vi "LaundryLab.vi"() -> ()   [LabVIEW 2016]
uses:
  Type Definitions/ViperHawk/ViperHawk Status.ctl
  Utility/Custom Pallet Controls/Custom Pallet String.ctl
  Utility/LabVIEW GEA2 Toolkit v1.0.0.0/type defs/Data In.ctl
  Utility/LabVIEW GEA2 Toolkit v1.0.0.0/type defs/Data Out.ctl
  Type Definitions/ViperHawk/ViperHawk Plot File.ctl
  Type Definitions/ViperHawk/ViperHawk Diagnostic Data.ctl
  Utility/Save File/Public/Type Definitions/Save File Software Version.ctl
  Type Definitions/ViperHawk/ViperHawk Summary Stats.ctl
  Utility/Save File/File Setup (Public)/Type Definition/Save File DOE File Path Control.ctl
  Utility/Save File/File Setup (Public)/Type Definition/Save File DOE Data Save Filepaths.ctl
  Type Definitions/ViperHawk/ViperHawk Data.ctl
  Type Definitions/ViperHawk/ViperHawk Search Control.ctl
  C:/Technology Lab/NI-2010/Trunk/Utility/LabVIEW GEA2 Toolkit v1.0.0.0/Appliance.NET/GeaCommunication.dll
  Utility/LabVIEW GEA2 Toolkit v1.0.0.0/Appliance.NET/GeaCommunication.dll
  Utility/GEA2 Commands/HEWH/Type Definitions/GEA2 Commands WaterHeater GEA2 Data.ctl
  Utility/GEA2 Commands/HEWH/Type Definitions/GEA2 Commands Button Status.ctl
  Utility/GEA2 Commands/HEWH/Type Definitions/GEA2 Commands Status Query.ctl
  Utility/GEA2 Commands/HEWH/Type Definitions/GEA2 Commands Service Error Codes.ctl
  Type Definitions/HCC Washer Types.ctl
  Utility/Save File/Public/Type Definitions/Save File Washer.ctl
  Utility/Save File/File Setup (Public)/Type Definition/Save File DISH Dishwasher Details.ctl
  <vilib>/Platform/fileVersionInfo.llb/FileVersionInformation.ctl
  Washer DOE/Type Definitions/DOE Appliance Common.ctl
  Utility/Save File/File Setup (Public)/Type Definition/DPT IMC Data.ctl
  Washer DOE/Type Definitions/DOE Dryer Standard.ctl
  Utility/Save File/Public/Type Definitions/Save File Appliance Display.ctl
  Utility/Save File/Public/Type Definitions/Save File Unit Type.ctl
  Type Definitions/2015 Program/Fault_Buffer_Status.ctl
  Type Definitions/2015 Program/Cycle_Diag_Buffer_Status.ctl
  Utility/LabVIEW GEA2 Toolkit v1.0.0.0/type defs/Source_Destination.ctl
  Utility/LabVIEW GEA2 Toolkit v1.0.0.0/type defs/ERD Write Data In.ctl
  Utility/LabVIEW GEA2 Toolkit v1.0.0.0/type defs/Data Type.ctl
  Utility/LabVIEW GEA2 Toolkit v1.0.0.0/type defs/ERD Read Data In.ctl
  Utility/LabVIEW GEA2 Toolkit v1.0.0.0/type defs/ERD Read Data Out.ctl
  Utility/Save File/Public/Type Definitions/Save File Headers.ctl
  Type Definitions/ViperHawk/ViperHawk Timers.ctl
  Utility/Save File/File Setup (Public)/Type Definition/Save File DOE LabView Program.ctl
  <vilib>/event_ctls.llb/lveventtype.ctl
  Type Definitions/ViperHawk/ViperHawk logData.ctl
  <vilib>/Utility/file.llb/Write Delimited Spreadsheet (string).vi
  Utility/LabVIEW GEA2 Toolkit v1.0.0.0/library/GEA2_Toolkit.lvlib
  user32.dll
  Utility/Save File/Save File.lvlib
  Utility/Save File/File Setup.lvlib
panel:
  out "Network Var Set":u8
  out "Diagnostic Data Output":T1={"Speed (RPM)"=39, "Load Size"=0, "Temperature"=105, "Water Pressure"=4130.0, "Detergent"=11000, "Fabric Softener"=11000, "Tub Direction"="CCW", "Detergent Valve"=FALSE, "Fabric Softener Valve"=FALSE, "Recirculating Pump"=FALSE, "Drain Valve"=FALSE, "Hot Valve"=FALSE, "Cold Valve"=FALSE, "Lid Closed Status"="", "Lid Lock Status"="", "Error Count"=0, "IGBT Temperature (Deg C)"=65, "Motor Speed"=21, "Latched OOB"=0, "Raw OOB"=2525, "Plaster Status"=0, "Inverter Power (W)"=453, "Target Speed(BRPM)"=0, "Latched Agitate Motor Temp (Deg C)"=123, "Current Motor Temp (Deg C)"=123, "Profiler Status"="A899", "Current Inverter Action"="Profiler", "Error Codes"="Door UnlockDoor Open", "Lid Locked"=TRUE, "Lid Closed"=TRUE, "9E Diagnostic Data"={"Total Cycle Time (Min)"=3002, "Total Cycle Count (Current)"=34, "Total Error Count"=21, "Machine Error History"=0, "Washer UI History"=0, "Inverter Error History"=342101761, "Cycle Storage Limit"=1, "Error Storage Limit"=0, "Cycle Pages Supported"=0, "Error Pages Supported"=129, "Inverter Reset Count"=0}, "9F Diagnostic Data"={"Cycle Buffer Index"="", "Page Number"="", "Total Cycle Count"=0, "Delay Start Time"=0, "Stain Selected"="", "Selected Cycle"=0, "eWash"="", "Soil Level"="", "Temperature"="", "Overnight Ready"="", "Spin Setting"="", "Control Lock Status"="", "Stain Remover"="", "Steam Assist"="", "My Cycle"="", "PreWash"="", "Debug Log Enabled"="", "Rinse"="", "Signal Level"="", "PreSoak"=""}}
  out "Diagnostic Data Local":T1={"Speed (RPM)"=0, "Load Size"=0, "Temperature"=0, "Water Pressure"=0.0, "Detergent"=0, "Fabric Softener"=0, "Tub Direction"="", "Detergent Valve"=FALSE, "Fabric Softener Valve"=FALSE, "Recirculating Pump"=FALSE, "Drain Valve"=FALSE, "Hot Valve"=FALSE, "Cold Valve"=FALSE, "Lid Closed Status"="", "Lid Lock Status"="", "Error Count"=0, "IGBT Temperature (Deg C)"=0, "Motor Speed"=0, "Latched OOB"=0, "Raw OOB"=0, "Plaster Status"=0, "Inverter Power (W)"=0, "Target Speed(BRPM)"=0, "Latched Agitate Motor Temp (Deg C)"=0, "Current Motor Temp (Deg C)"=0, "Profiler Status"="", "Current Inverter Action"="", "Error Codes"="", "Lid Locked"=FALSE, "Lid Closed"=FALSE, "9E Diagnostic Data"={"Total Cycle Time (Min)"=3002, "Total Cycle Count (Current)"=34, "Total Error Count"=21, "Machine Error History"=0, "Washer UI History"=0, "Inverter Error History"=342101761, "Cycle Storage Limit"=1, "Error Storage Limit"=0, "Cycle Pages Supported"=0, "Error Pages Supported"=129, "Inverter Reset Count"=0}, "9F Diagnostic Data"={"Cycle Buffer Index"="", "Page Number"="", "Total Cycle Count"=0, "Delay Start Time"=0, "Stain Selected"="", "Selected Cycle"=0, "eWash"="", "Soil Level"="", "Temperature"="", "Overnight Ready"="", "Spin Setting"="", "Control Lock Status"="", "Stain Remover"="", "Steam Assist"="", "My Cycle"="", "PreWash"="", "Debug Log Enabled"="", "Rinse"="", "Signal Level"="", "PreSoak"=""}}
  out "GEA Information Out":T2={"GEA Diagnostic Data - Washer"={"Speed (RPM)"=39, "Load Size"=0, "Temperature"=105, "Water Pressure"=4130.0, "Detergent"=11000, "Fabric Softener"=11000, "Tub Direction"="CCW", "Detergent Valve"=FALSE, "Fabric Softener Valve"=FALSE, "Recirculating Pump"=FALSE, "Drain Valve"=FALSE, "Hot Valve"=FALSE, "Cold Valve"=FALSE, "Lid Closed Status"="", "Lid Lock Status"="", "Error Count"=0, "IGBT Temperature (Deg C)"=65, "Motor Speed"=21, "Latched OOB"=0, "Raw OOB"=2525, "Plaster Status"=0, "Inverter Power (W)"=453, "Target Speed(BRPM)"=0, "Latched Agitate Motor Temp (Deg C)"=123, "Current Motor Temp (Deg C)"=123, "Profiler Status"="A899", "Current Inverter Action"="Profiler", "Error Codes"="Door UnlockDoor Open", "Lid Locked"=TRUE, "Lid Closed"=TRUE, "9E Diagnostic Data"={"Total Cycle Time (Min)"=3002, "Total Cycle Count (Current)"=34, "Total Error Count"=21, "Machine Error History"=0, "Washer UI History"=0, "Inverter Error History"=342101761, "Cycle Storage Limit"=1, "Error Storage Limit"=0, "Cycle Pages Supported"=0, "Error Pages Supported"=129, "Inverter Reset Count"=0}, "9F Diagnostic Data"={"Cycle Buffer Index"="", "Page Number"="", "Total Cycle Count"=0, "Delay Start Time"=0, "Stain Selected"="", "Selected Cycle"=0, "eWash"="", "Soil Level"="", "Temperature"="", "Overnight Ready"="", "Spin Setting"="", "Control Lock Status"="", "Stain Remover"="", "Steam Assist"="", "My Cycle"="", "PreWash"="", "Debug Log Enabled"="", "Rinse"="", "Signal Level"="", "PreSoak"=""}}, "Software Version"={"Critical Major SW Version"="0", "Critical Minor SW Version"="0", "Major SW Version"="41", "Minor SW Version"="1", "Parametric Data Ver. Major"="1", "Parametric Data Ver. Minor"="1", "Diagnostics Data Ver. Major"="", "Diagnostics Data Ver. Minor"="", "Current Personality Setting"=""}, "Debug Search Parameters"={"Pause"=["MchStdby", "MchPz", "MchIdl", "Machine Standby", "Machine Pause", "Machine Idle"], "Run"=["MchRn", "Machine Run", "Resume Process"], "EOC"=["EOC"], "Error Codes"=["Error1", "try", "rty", "inverr"]}, "Message Count"=0, "Number of Messages"=0, "Partial Message String"="", "Full Message to Save"="117 1MnPwrDtaStrd", "Board ID"="", "Board Index"=0, "Source Address"=228, "Destination Address"=35, "Data to send"=[], "ReceivedData"=[1, 0, 21, 0, 0, 0, 0, 9, 221, 65, 0, 1, 197, 1, 168, 153, 9, 0, 0, 123, 123], "Debug/GEA Data"=["11/06/2015", "10:20:16.735", "117 1MnPwrDtaStrd"], "Command"=0, "GEA2 Reference Out"=refnum, "GEA2 Event Registration"=refnum, "Bus Data"="11/06/15 10:20:40.531 RECV 3F E4 60 7B 7B 00 00 09 99 A8 01 C5 01 00 41 DD 09 00 00 00 00 15 00 01\r\n11/06/15 10:20:40.466 RECV 21 E4 41 27 00 00 00 06 00 EA 00 F8 2A F8 2A 01 08 00 00 0B C7 00 22 10 00 00 00 00 69\r\n11/06/15 10:20:39.988 RECV 23 FF A4 16 03 02\r\n11/06/15 10:20:39.537 RECV 3F E4 60 7B 7B 6E 00 09 99 A8 01 B7 01 00 41 64 14 00 00 00 00 69 00 01\r\n11/06/15 10:20:39.472 RECV 21 E4 41 68 00 00 00 06 00 EA 00 F8 2A F8 2A 11 08 00 00 0B C7 00 19 10 00 00 00 00 69\r\n11/06/15 10:20:38.996 RECV 23 FF A4 16 03 02\r\n11/06/15 10:20:38.871 RECV 23 E4 9E 81 00 00 01 01 0F 64 14 00 00 00 00 00 00 00 00 15 00 22 00 BA 0B 00 00\r\n11/06/15 10:20:38.577 RECV 3F E4 60 7B 7B 00 00 09 99 A8 01 96 01 00 41 87 01 00 00 00 00 24 00 00\r\n11/06/15 10:20:38.512 RECV 21 E4 41 35 00 00 00 06 00 EA 00 F8 2A F8 2A 11 08 00 00 0B C7 00 1A 10 00 00 00 00 69\r\n11/06/15 10:20:38.005 RECV 23 FF A4 16 03 02\r\n11/06/15 10:20:37.553 RECV 3F E4 60 7B 7B 6E 00 09 99 A8 01 9E 01 00 41 56 02 00 00 00 00 64 00 00\r\n11/06/15 10:20:37.486 RECV 21 E4 41 64 00 00 00 06 00 EA 00 F8 2A F8 2A 11 08 00 00 0B C7 00 21 10 00 00 00 00 6A\r\n11/06/15 10:20:37.010 RECV 23 FF A4 16 03 02\r\n11/06/15 10:20:36.558 RECV 3F E4 60 7B 7B 00 00 09 99 A8 01 C7 01 00 41 8C 3D 00 00 00 00 35 00 01\r\n11/06/15 10:20:36.493 RECV 21 E4 41 38 00 00 00 06 00 EA 00 F8 2A F8 2A 11 08 00 00 0B C7 00 1F 10 00 00 00 00 6A\r\n11/06/15 10:20:36.312 RECV 23 E4 9E 81 00 00 01 01 0F 64 14 00 00 00 00 00 00 00 00 15 00 22 00 BA 0B 00 00\r\n11/06/15 10:20:36.017 RECV 23 FF A4 16 03 02\r\n11/06/15 10:20:35.567 RECV 3F E4 60 7B 7B 6E 00 09 99 A8 01 6B 01 00 41 5F 08 00 00 00 00 5F 00 01\r\n11/06/15 10:20:35.501 RECV 21 E4 41 63 00 00 00 06 00 EA 00 F8 2A F8 2A 11 08 00 00 0B C7 00 18 10 00 00 00 00 6A\r\n11/06/15 10:20:35.024 RECV 23 FF A4 16 03 02\r\n11/06/15 10:20:34.573 RECV 3F E4 60 7B 7B 00 00 09 99 A8 01 FF 01 00 41 30 05 00 00 00 00 3D 00 00\r\n11/06/15 10:20:34.505 RECV 21 E4 41 52 00 00 00 06 00 EA 00 F8 2A F8 2A 11 08 00 00 0B C7 00 1D 10 00 00 00 00 6A\r\n11/06/15 10:20:34.031 RECV 23 FF A4 16 03 02\r\n11/06/15 10:20:33.877 RECV 23 E4 9E 81 00 00 01 01 0F 64 14 00 00 00 00 00 00 00 00 15 00 22 00 BA 0B 00 00\r\n11/06/15 10:20:33.581 RECV 3F E4 60 7B 7B 6E 00 09 99 A8 01 95 01 00 41 20 09 00 00 00 00 66 00 00\r\n11/06/15 10:20:33.515 RECV 21 E4 41 5F 00 00 00 06 00 EA 00 F8 2A F8 2A 11 08 00 00 0B C7 00 1F 10 00 00 00 00 6A\r\n11/06/15 10:20:33.038 RECV 23 FF A4 16 03 02\r\n11/06/15 10:20:32.585 RECV 3F E4 60 7B 7B 1E 00 09 99 A8 01 13 02 00 40 4C 0E 00 00 00 00 4C 00 01\r\n11/06/15 10:20:32.519 RECV 21 E4 41 5C 00 00 00 06 00 EA 00 F8 2A F8 2A 11 08 00 00 0B C7 00 1D 10 00 00 00 00 6A\r\n11/06/15 10:20:32.045 RECV 23 FF A4 16 03 02\r\n11/06/15 10:20:31.594 RECV 3F E4 60 7B 7B 6E 00 09 99 A8 01 42 01 00 40 A6 01 00 00 00 00 5F 00 01\r\n11/06/15 10:20:31.527 RECV 21 E4 41 54 00 00 00 06 00 EA 00 F8 2A F8 2A 11 08 00 00 0B C7 00 17 10 00 00 00 00 6A\r\n11/06/15 10:20:31.347 RECV 23 E4 9E 81 00 00 01 01 0F 64 14 00 00 00 00 00 00 00 00 15 00 22 00 BA 0B 00 00\r\n11/06/15 10:20:31.052 RECV 23 FF A4 16 03 02\r\n11/06/15 10:20:30.603 RECV 3F E4 60 7B 7B 1E 00 09 99 A8 01 0B 02 00 40 91 0A 00 00 00 00 6A 00 00\r\n11/06/15 10:20:30.534 RECV 21 E4 41 6E 00 00 00 06 00 EA 00 F8 2A F8 2A 11 08 00 00 0B C7 00 1C 10 00 00 00 00 6A\r\n11/06/15 10:20:30.060 RECV 23 FF A4 16 03 02\r\n11/06/15 10:20:29.607 RECV 3F E4 60 7B 7B 6E 00 09 99 A8 01 45 01 00 40 47 21 00 00 00 00 47 00 00\r\n11/06/15 10:20:29.541 RECV 21 E4 41 2C 00 00 00 06 00 EA 00 F8 2A F8 2A 01 08 00 00 0B C7 00 25 10 00 00 00 00 6A\r\n11/06/15 10:20:29.066 RECV 23 FF A4 16 03 02\r\n11/06/15 10:20:28.912 RECV 23 E4 9E 81 00 00 01 01 0F 64 14 00 00 00 00 00 00 00 00 15 00 22 00 BA 0B 00 00\r\n11/06/15 10:20:28.615 RECV 3F E4 60 7B 7B 6E 00 09 99 A8 01 E7 01 00 40 66 1A 00 00 00 00 6B 00 01\r\n11/06/15 10:20:28.549 RECV 21 E4 41 66 00 00 00 06 00 EA 00 F8 2A F8 2A 11 08 00 00 0B C7 00 25 10 00 00 00 00 6A\r\n11/06/15 10:20:28.073 RECV 23 FF A4 16 03 02\r\n11/06/15 10:20:27.619 RECV 3F E4 60 7B 7B 6E 00 09 99 A8 01 99 00 00 40 E4 20 00 00 00 00 15 00 01\r\n11/06/15 10:20:27.555 RECV 21 E4 41 03 00 00 00 06 00 EA 00 F8 2A F8 2A 01 08 00 00 0B C7 00 23 10 00 00 00 00 6A\r\n11/06/15 10:20:27.080 RECV 23 FF A4 16 03 02\r\n11/06/15 10:20:26.628 RECV 3F E4 60 68 68 00 00 09 99 A8 05 66 00 00 40 00 00 00 00 00 00 01 00 02\r\n11/06/15 10:20:26.563 RECV 21 E4 41 04 00 00 00 06 00 EA 00 F8 2A F8 2A 01 08 00 00 0B C7 00 21 10 00 00 00 00 6A\r\n11/06/15 10:20:26.384 RECV 23 E4 9E 81 00 00 01 01 0F 64 14 00 00 00 00 00 00 00 00 15 00 22 00 BA 0B 00 00\r\n11/06/15 10:20:26.086 RECV 23 FF A4 16 03 02\r\n11/06/15 10:20:25.633 RECV 3F E4 60 68 68 00 00 09 99 A8 05 17 00 00 40 0C 00 00 00 00 00 01 00 00\r\n11/06/15 10:20:25.570 RECV 21 E4 41 09 00 00 00 06 00 EA 00 F8 2A F8 2A 01 08 00 00 0B C7 00 23 10 00 00 00 00 6A\r\n11/06/15 10:20:25.093 RECV 23 FF A4 16 03 02\r\n11/06/15 10:20:24.640 RECV 3F E4 60 68 68 00 00 09 99 A8 05 A0 00 00 40 FA 01 00 00 00 00 06 00 00\r\n11/06/15 10:20:24.576 RECV 21 E4 41 0D 00 00 00 06 00 EA 00 F8 2A F8 2A 01 08 00 00 0B C7 00 20 10 00 00 00 00 6A\r\n11/06/15 10:20:24.100 RECV 23 FF A4 16 03 02\r\n11/06/15 10:20:23.947 RECV 23 E4 9E 81 00 00 01 01 0F 64 14 00 00 00 00 00 00 00 00 15 00 22 00 BA 0B 00 00\r\n11/06/15 10:20:23.651 RECV 3F E4 60 68 68 6E 00 09 99 A8 01 FF 01 00 40 8C 08 00 00 00 00 6E 00 00\r\n11/06/15 10:20:23.583 RECV 21 E4 41 6D 00 00 00 06 00 EA 00 F8 2A F8 2A 11 08 00 00 0B C7 00 1E 10 00 00 00 00 6A\r\n11/06/15 10:20:23.110 RECV 23 FF A4 16 03 02\r\n11/06/15 10:20:22.656 RECV 3F E4 60 68 68 6E 00 09 99 A8 01 C2 01 00 40 74 0B 00 00 00 00 23 00 01\r\n11/06/15 10:20:22.590 RECV 21 E4 41 51 00 00 00 06 00 EA 00 F8 2A F8 2A 11 08 00 00 0B C7 00 1B 10 00 00 00 00 6A\r\n11/06/15 10:20:22.115 RECV 23 FF A4 16 03 02\r\n11/06/15 10:20:21.662 RECV 3F E4 60 68 68 6E 00 09 99 A8 01 8D 01 00 40 F5 0D 00 00 00 00 5C 00 01\r\n11/06/15 10:20:21.596 RECV 21 E4 41 5E 00 00 00 06 00 EA 00 F8 2A F8 2A 11 08 00 00 0B C7 00 13 10 00 00 00 00 6A\r\n11/06/15 10:20:21.419 RECV 23 E4 9E 81 00 00 01 01 0F 64 14 00 00 00 00 00 00 00 00 15 00 22 00 BA 0B 00 00\r\n11/06/15 10:20:21.122 RECV 23 FF A4 16 03 02\r\n11/06/15 10:20:20.671 RECV 3F E4 60 68 68 6E 00 09 99 A8 01 F7 01 00 40 EA 0C 00 00 00 00 67 00 00\r\n11/06/15 10:20:20.605 RECV 21 E4 41 6E 00 00 00 06 00 EA 00 F8 2A F8 2A 11 08 00 00 0B C7 00 18 10 00 00 00 00 6A\r\n11/06/15 10:20:20.128 RECV 23 FF A4 16 03 02\r\n11/06/15 10:20:19.678 RECV 3F E4 60 68 68 6E 00 09 99 A8 01 54 01 00 40 96 12 00 00 00 00 35 00 00\r\n11/06/15 10:20:19.611 RECV 21 E4 41 25 00 00 00 06 00 EA 00 F8 2A F8 2A 01 08 00 00 0B C7 00 1B 10 00 00 00 00 6A\r\n11/06/15 10:20:19.135 RECV 23 FF A4 16 03 02\r\n11/06/15 10:20:19.006 RECV 23 E4 9E 81 00 00 01 01 0F 64 14 00 00 00 00 00 00 00 00 15 00 22 00 BA 0B 00 00\r\n11/06/15 10:20:18.699 RECV 3F E4 60 68 68 6E 00 09 99 A8 01 4E 01 00 40 05 05 00 00 00 00 67 00 01\r\n11/06/15 10:20:18.616 RECV 21 E4 41 67 00 00 00 06 00 EA 00 F8 2A F8 2A 11 08 00 00 0B C7 00 1C 10 00 00 00 00 6A\r\n11/06/15 10:20:18.146 RECV 23 FF A4 16 03 02\r\n11/06/15 10:20:17.717 RECV 3F E4 60 68 68 00 00 09 99 A8 01 5D 01 00 40 30 05 00 00 00 00 25 00 00\r\n11/06/15 10:20:17.616 RECV 21 E4 41 34 00 00 00 06 00 EA 00 F8 2A F8 2A 11 08 00 00 0B C7 00 1D 10 00 00 00 00 6A\r\n11/06/15 10:20:17.148 RECV 23 FF A4 16 03 02\r\n11/06/15 10:20:16.729 RECV 23 FF 74 0A 64 72 74 53 61 74 44 72 77 50 6E 4D 31 20 37 31 31\r\n11/06/15 10:20:16.700 RECV 3F E4 60 68 68 6E 00 09 99 A8 01 90 01 00 40 55 12 00 00 00 00 65 00 00\r\n11/06/15 10:20:16.629 RECV 21 E4 41 64 00 00 00 06 00 EA 00 F8 2A F8 2A 11 08 00 00 0B C7 00 17 10 00 00 00 00 6A\r\n11/06/15 10:20:16.450 RECV 23 E4 9E 81 00 00 01 01 0F 64 14 00 00 00 00 00 00 00 00 15 00 22 00 BA 0B 00 00\r\n11/06/15 10:20:16.155 RECV 23 FF A4 16 03 02\r\n11/06/15 10:20:15.738 RECV 3F E4 60 68 68 00 00 09 99 A8 01 D5 01 00 40 7E 32 00 00 00 00 36 00 01\r\n11/06/15 10:20:15.672 RECV 21 E4 41 39 00 00 00 06 00 EA 00 F8 2A F8 2A 11 08 00 00 0B C7 00 1B 10 00 00 00 00 6A\r\n11/06/15 10:20:15.163 RECV 23 FF A4 16 03 02\r\n11/06/15 10:20:14.738 RECV 3F E4 60 68 68 6E 00 09 99 A8 01 45 01 00 40 28 0A 00 00 00 00 68 00 01\r\n11/06/15 10:20:14.644 RECV 21 E4 41 63 00 00 00 06 00 EA 00 F8 2A F8 2A 11 08 00 00 0B C7 00 18 10 00 00 00 00 6A\r\n11/06/15 10:20:14.170 RECV 23 FF A4 16 03 02\r\n11/06/15 10:20:14.013 RECV 23 E4 9E 81 00 00 01 01 0F 64 14 00 00 00 00 00 00 00 00 15 00 22 00 BA 0B 00 00\r\n11/06/15 10:20:13.717 RECV 3F E4 60 68 68 1E 00 09 99 A8 01 7D 01 00 40 57 17 00 00 00 00 3D 00 00\r\n11/06/15 10:20:13.651 RECV 21 E4 41 51 00 00 00 06 00 EA 00 F8 2A F8 2A 11 08 00 00 0B C7 00 16 10 00 00 00 00 6A\r\n11/06/15 10:20:13.176 RECV 23 FF A4 16 03 02\r\n11/06/15 10:20:12.753 RECV 3F E4 60 68 68 6E 00 09 99 A8 01 3F 01 00 40 EC 09 00 00 00 00 58 00 00\r\n11/06/15 10:20:12.658 RECV 21 E4 41 54 00 00 00 06 00 EA 00 F8 2A F8 2A 11 08 00 00 0B C7 00 17 10 00 00 00 00 6A\r\n11/06/15 10:20:12.184 RECV 23 FF A4 16 03 02\r\n11/06/15 10:20:11.733 RECV 3F E4 60 68 68 1E 00 09 99 A8 01 9E 01 00 40 B6 00 00 00 00 00 59 00 01\r\n11/06/15 10:20:11.667 RECV 21 E4 41 64 00 00 00 06 00 EA 00 F8 2A F8 2A 11 08 00 00 0B C7 00 19 10 00 00 00 00 6A\r\n11/06/15 10:20:11.488 RECV 23 E4 9E 81 00 00 01 01 0F 64 14 00 00 00 00 00 00 00 00 15 00 22 00 BA 0B 00 00\r\n11/06/15 10:20:11.191 RECV 23 FF A4 16 03 02\r\n11/06/15 10:20:10.759 RECV 3F E4 60 68 68 6E 00 09 99 A8 01 0C 01 00 40 45 01 00 00 00 00 57 00 01\r\n11/06/15 10:20:10.673 RECV 21 E4 41 50 00 00 00 06 00 EA 00 F8 2A F8 2A 11 08 00 00 0B C7 00 1C 10 00 00 00 00 6A\r\n11/06/15 10:20:10.198 RECV 23 FF A4 16 03 02\r\n11/06/15 10:20:09.749 RECV 3F E4 60 68 68 1E 00 09 99 A8 01 D1 01 00 40 96 0A 00 00 00 00 6D 00 00\r\n11/06/15 10:20:09.681 RECV 21 E4 41 6F 00 00 00 06 00 EA 00 F8 2A F8 2A 11 08 00 00 0B C7 00 24 10 00 00 00 00 6A\r\n11/06/15 10:20:09.205 RECV 23 FF A4 16 03 02\r\n11/06/15 10:20:09.110 RECV 23 E4 9E 81 00 00 01 01 0F 64 14 00 00 00 00 00 00 00 00 15 00 22 00 BA 0B 00 00\r\n11/06/15 10:20:08.813 RECV 3F E4 60 68 68 6E 00 09 99 A8 01 18 01 00 40 64 04 00 00 00 00 4F 00 00\r\n11/06/15 10:20:08.749 RECV 21 E4 41 43 00 00 00 06 00 EA 00 F8 2A F8 2A 11 08 00 00 0B C7 00 1F 10 00 00 00 00 6A\r\n11/06/15 10:20:08.212 RECV 23 FF A4 16 03 02\r\n11/06/15 10:20:07.760 RECV 3F E4 60 68 68 6E 00 09 99 A8 01 C1 01 00 40 51 05 00 00 00 00 6C 00 01\r\n11/06/15 10:20:07.693 RECV 21 E4 41 6C 00 00 00 06 00 EA 00 F8 2A F8 2A 11 08 00 00 0B C7 00 19 10 00 00 00 00 6A\r\n11/06/15 10:20:07.218 RECV 23 FF A4 16 03 02\r\n11/06/15 10:20:06.764 RECV 3F E4 60 68 68 6E 00 09 99 A8 01 08 01 00 40 26 34 00 00 00 00 38 00 01\r\n11/06/15 10:20:06.698 RECV 21 E4 41 19 00 00 00 06 00 EA 00 F8 2A F8 2A 01 08 00 00 0B C7 00 15 10 00 00 00 00 6A\r\n11/06/15 10:20:06.522 RECV 23 E4 9E 81 00 00 01 01 0F 64 14 00 00 00 00 00 00 00 00 15 00 22 00 BA 0B 00 00\r\n11/06/15 10:20:06.226 RECV 23 FF A4 16 03 02\r\n11/06/15 10:20:05.775 RECV 3F E4 60 68 68 6E 00 09 99 A8 01 C9 01 00 40 4A 09 00 00 00 00 6A 00 00\r\n11/06/15 10:20:05.709 RECV 21 E4 41 6B 00 00 00 06 00 EA 00 F8 2A F8 2A 11 08 00 00 0B C7 00 17 10 00 00 00 00 6A\r\n11/06/15 10:20:05.232 RECV 23 FF A4 16 03 02\r\n11/06/15 10:20:04.714 RECV 21 E4 41 1A 00 00 00 06 00 EA 00 F8 2A F8 2A 01 08 00 00 0B C7 00 1B 10 00 00 00 00 6A\r\n11/06/15 10:20:04.239 RECV 23 FF A4 16 03 02\r\n11/06/15 10:20:04.082 RECV 23 E4 9E 81 00 00 01 01 0F 64 14 00 00 00 00 00 00 00 00 15 00 22 00 BA 0B 00 00\r\n11/06/15 10:20:03.787 RECV 3F E4 60 68 68 6E 00 09 99 A8 01 B2 01 00 40 2C 09 00 00 00 00 6B 00 01\r\n11/06/15 10:20:03.723 RECV 21 E4 41 6D 00 00 00 06 00 EA 00 F8 2A F8 2A 11 08 00 00 0B C7 00 1C 10 00 00 00 00 6A\r\n11/06/15 10:20:03.246 RECV 23 FF A4 16 03 02\r\n11/06/15 10:20:02.794 RECV 3F E4 60 68 68 6E 00 09 99 A8 01 0F 01 00 40 16 01 00 00 00 00 0C 00 01\r\n11/06/15 10:20:02.728 RECV 21 E4 41 25 00 00 00 06 00 EA 00 F8 2A F8 2A 01 08 00 00 0B C7 00 1E 10 00 00 00 00 6A\r\n11/06/15 10:20:02.253 RECV 23 FF A4 16 03 02\r\n11/06/15 10:20:01.817 RECV 3F E4 60 68 68 6E 00 09 99 A8 01 D5 01 00 40 F1 07 00 00 00 00 67 00 00\r\n11/06/15 10:20:01.736 RECV 21 E4 41 69 00 00 00 06 00 EA 00 F8 2A F8 2A 11 08 00 00 0B C7 00 1F 10 00 00 00 00 6A\r\n11/06/15 10:20:01.557 RECV 23 E4 9E 81 00 00 01 01 0F 64 14 00 00 00 00 00 00 00 00 15 00 22 00 BA 0B 00 00\r\n11/06/15 10:20:01.261 RECV 23 FF A4 16 03 02\r\n11/06/15 10:20:00.817 RECV 3F E4 60 68 68 00 00 09 99 A8 01 80 01 00 40 59 08 00 00 00 00 16 00 01\r\n11/06/15 10:20:00.741 RECV 21 E4 41 29 00 00 00 06 00 EA 00 F8 2A F8 2A 01 08 00 00 0B C7 00 1F 10 00 00 00 00 6A\r\n11/06/15 10:20:00.267 RECV 23 FF A4 16 03 02\r\n11/06/15 10:19:59.748 RECV 21 E4 41 63 00 00 00 06 00 EA 00 F8 2A F8 2A 11 08 00 00 0B C7 00 19 10 00 00 00 00 6A\r\n11/06/15 10:19:59.275 RECV 23 FF A4 16 03 02\r\n11/06/15 10:19:59.116 RECV 23 E4 9E 81 00 00 01 01 0F 64 14 00 00 00 00 00 00 00 00 15 00 22 00 BA 0B 00 00\r\n11/06/15 10:19:58.821 RECV 3F E4 60 68 68 00 00 09 99 A8 01 5F 01 00 40 AB 06 00 00 00 00 20 00 00\r\n11/06/15 10:19:58.756 RECV 21 E4 41 2E 00 00 00 06 00 EA 00 F8 2A F8 2A 01 08 00 00 0B C7 00 1C 10 00 00 00 00 6A\r\n11/06/15 10:19:58.279 RECV 23 FF A4 16 03 02\r\n11/06/15 10:19:57.869 RECV 3F E4 60 68 68 6E 00 09 99 A8 01 A8 01 00 40 5A 04 00 00 00 00 6F 00 00\r\n11/06/15 10:19:57.763 RECV 21 E4 41 69 00 00 00 06 00 EA 00 F8 2A F8 2A 11 08 00 00 0B C7 00 1C 10 00 00 00 00 6A\r\n11/06/15 10:19:57.288 RECV 23 FF A4 16 03 02\r\n11/06/15 10:19:56.853 RECV 3F E4 60 68 68 00 00 09 99 A8 01 AC 01 00 40 00 08 00 00 00 00 20 00 01\r\n11/06/15 10:19:56.771 RECV 21 E4 41 39 00 00 00 06 00 EA 00 F8 2A F8 2A 11 08 00 00 0B C7 00 1C 10 00 00 00 00 6A\r\n11/06/15 10:19:56.591 RECV 23 E4 9E 81 00 00 01 01 0F 64 14 00 00 00 00 00 00 00 00 15 00 22 00 BA 0B 00 00\r\n11/06/15 10:19:56.294 RECV 23 FF A4 16 03 02\r\n11/06/15 10:19:55.840 RECV 3F E4 60 68 68 6E 00 09 99 A8 01 8D 01 00 40 17 13 00 00 00 00 6A 00 01\r\n11/06/15 10:19:55.773 RECV 21 E4 41 67 00 00 00 06 00 EA 00 F8 2A F8 2A 11 08 00 00 0B C7 00 1C 10 00 00 00 00 6A\r\n11/06/15 10:19:55.298 RECV 23 FF A4 16 03 02\r\n11/06/15 10:19:54.865 RECV 3F E4 60 68 68 00 00 09 99 A8 01 B0 01 00 3F DE 17 00 00 00 00 36 00 00\r\n11/06/15 10:19:54.783 RECV 21 E4 41 48 00 00 00 06 00 EA 00 F8 2A F8 2A 11 08 00 00 0B C7 00 20 10 00 00 00 00 6A\r\n11/06/15 10:19:54.308 RECV 23 FF A4 16 03 02\r\n11/06/15 10:19:54.153 RECV 23 E4 9E 81 00 00 01 01 0F 64 14 00 00 00 00 00 00 00 00 15 00 22 00 BA 0B 00 00\r\n11/06/15 10:19:53.856 RECV 3F E4 60 68 68 6E 00 09 99 A8 01 83 01 00 3F CD 06 00 00 00 00 5F 00 00\r\n11/06/15 10:19:53.790 RECV 21 E4 41 5D 00 00 00 06 00 EA 00 F8 2A F8 2A 11 08 00 00 0B C7 00 1C 10 00 00 00 00 6A\r\n11/06/15 10:19:53.316 RECV 23 FF A4 16 03 02\r\n11/06/15 10:19:52.865 RECV 3F E4 60 68 68 1E 00 09 99 A8 01 DA 01 00 3F EB 22 00 00 00 00 40 00 01\r\n11/06/15 10:19:52.798 RECV 21 E4 41 5E 00 00 00 06 00 EA 00 F8 2A F8 2A 11 08 00 00 0B C7 00 1E 10 00 00 00 00 6A\r\n11/06/15 10:19:52.322 RECV 23 FF A4 16 03 02\r\n11/06/15 10:19:51.871 RECV 3F E4 60 68 68 6E 00 09 99 A8 01 48 01 00 3F EF 00 00 00 00 00 57 00 01\r\n11/06/15 10:19:51.807 RECV 21 E4 41 53 00 00 00 06 00 EA 00 F8 2A F8 2A 11 08 00 00 0B C7 00 20 10 00 00 00 00 6A\r\n11/06/15 10:19:51.626 RECV 23 E4 9E 81 00 00 01 01 0F 64 14 00 00 00 00 00 00 00 00 15 00 22 00 BA 0B 00 00\r\n11/06/15 10:19:51.329 RECV 23 FF A4 16 03 02\r\n11/06/15 10:19:50.878 RECV 3F E4 60 68 68 1E 00 09 99 A8 01 D7 01 00 3F 97 06 00 00 00 00 66 00 00\r\n11/06/15 10:19:50.811 RECV 21 E4 41 69 00 00 00 06 00 EA 00 F8 2A F8 2A 11 08 00 00 0B C7 00 1E 10 00 00 00 00 6A\r\n11/06/15 10:19:50.337 RECV 23 FF A4 16 03 02\r\n11/06/15 10:19:49.884 RECV 3F E4 60 68 68 6E 00 09 99 A8 01 3D 01 00 3F 5C 17 00 00 00 00 4D 00 00\r\n11/06/15 10:19:49.819 RECV 21 E4 41 45 00 00 00 06 00 EA 00 F8 2A F8 2A 11 08 00 00 0B C7 00 1B 10 00 00 00 00 6A\r\n11/06/15 10:19:49.343 RECV 23 FF A4 16 03 02\r\n11/06/15 10:19:49.191 RECV 23 E4 9E 81 00 00 01 01 0F 64 14 00 00 00 00 00 00 00 00 15 00 22 00 BA 0B 00 00\r\n11/06/15 10:19:48.893 RECV 3F E4 60 68 68 6E 00 09 99 A8 01 CA 01 00 3F EB 03 00 00 00 00 6C 00 01\r\n11/06/15 10:19:48.826 RECV 21 E4 41 70 00 00 00 06 00 EA 00 F8 2A F8 2A 11 08 00 00 0B C7 00 1C 10 00 00 00 00 6A\r\n11/06/15 10:19:48.350 RECV 23 FF A4 16 03 02\r\n11/06/15 10:19:47.898 RECV 3F E4 60 68 68 6E 00 09 99 A8 01 14 01 00 3F 88 08 00 00 00 00 47 00 01\r\n11/06/15 10:19:47.833 RECV 21 E4 41 24 00 00 00 06 00 EA 00 F8 2A F8 2A 01 08 00 00 0B C7 00 1C 10 00 00 00 00 6A\r\n11/06/15 10:19:47.357 RECV 23 FF A4 16 03 02\r\n11/06/15 10:19:46.906 RECV 3F E4 60 68 68 6E 00 09 99 A8 01 E3 01 00 3F 78 13 00 00 00 00 6B 00 00\r\n11/06/15 10:19:46.838 RECV 21 E4 41 6D 00 00 00 06 00 EA 00 F8 2A F8 2A 11 08 00 00 0B C7 00 1B 10 00 00 00 00 6A\r\n11/06/15 10:19:46.659 RECV 23 E4 9E 81 00 00 01 01 0F 64 14 00 00 00 00 00 00 00 00 15 00 22 00 BA 0B 00 00\r\n11/06/15 10:19:46.363 RECV 23 FF A4 16 03 02\r\n11/06/15 10:19:45.910 RECV 3F E4 60 68 68 6E 00 09 99 A8 01 2F 01 00 3F D7 1C 00 00 00 00 36 00 00\r\n11/06/15 10:19:45.845 RECV 21 E4 41 1A 00 00 00 06 00 EA 00 F8 2A F8 2A 01 08 00 00 0B C7 00 14 10 00 00 00 00 6A\r\n11/06/15 10:19:45.370 RECV 23 FF A4 16 03 02\r\n11/06/15 10:19:44.919 RECV 3F E4 60 68 68 6E 00 09 99 A8 01 1A 02 00 3F 1D 29 00 00 00 00 4E 00 01\r\n11/06/15 10:19:44.852 RECV 21 E4 41 63 00 00 00 06 00 EA 00 F8 2A F8 2A 11 08 00 00 0B C7 00 16 10 00 00 00 00 6A\r\n11/06/15 10:19:44.377 RECV 23 FF A4 16 03 02\r\n11/06/15 10:19:44.221 RECV 23 E4 9E 81 00 00 01 01 0F 64 14 00 00 00 00 00 00 00 00 15 00 22 00 BA 0B 00 00\r\n11/06/15 10:19:43.925 RECV 3F E4 60 68 68 6E 00 09 99 A8 01 1C 01 00 3F 7A 0C 00 00 00 00 0A 00 01\r\n11/06/15 10:19:43.859 RECV 21 E4 41 22 00 00 00 06 00 EA 00 F8 2A F8 2A 01 08 00 00 0B C7 00 18 10 00 00 00 00 6A\r\n11/06/15 10:19:43.384 RECV 23 FF A4 16 03 02\r\n11/06/15 10:19:42.950 RECV 3F E4 60 68 68 6E 00 09 99 A8 01 F3 01 00 3F B0 0F 00 00 00 00 69 00 00\r\n11/06/15 10:19:42.867 RECV 21 E4 41 6C 00 00 00 06 00 EA 00 F8 2A F8 2A 11 08 00 00 0B C7 00 1C 10 00 00 00 00 6A\r\n11/06/15 10:19:42.391 RECV 23 FF A4 16 03 02\r\n11/06/15 10:19:41.939 RECV 3F E4 60 68 68 6E 00 09 99 A8 01 60 01 00 3F 28 00 00 00 00 00 11 00 00\r\n11/06/15 10:19:41.875 RECV 21 E4 41 21 00 00 00 06 00 EA 00 F8 2A F8 2A 01 08 00 00 0B C7 00 1C 10 00 00 00 00 6A\r\n11/06/15 10:19:41.694 RECV 23 E4 9E 81 00 00 01 01 0F 64 14 00 00 00 00 00 00 00 00 15 00 22 00 BA 0B 00 00\r\n11/06/15 10:19:41.398 RECV 23 FF A4 16 03 02\r\n11/06/15 10:19:40.974 RECV 3F E4 60 68 68 6E 00 09 99 A8 01 BD 01 00 3F 5F 02 00 00 00 00 5E 00 01\r\n11/06/15 10:19:40.880 RECV 21 E4 41 6B 00 00 00 06 00 EA 00 F8 2A F8 2A 11 08 00 00 0B C7 00 1C 10 00 00 00 00 6A\r\n11/06/15 10:19:40.406 RECV 23 FF A4 16 03 02\r\n11/06/15 10:19:39.952 RECV 3F E4 60 68 68 00 00 09 99 A8 01 54 01 00 3F 70 07 00 00 00 00 14 00 00\r\n11/06/15 10:19:39.885 RECV 21 E4 41 30 00 00 00 06 00 EA 00 F8 2A F8 2A 01 08 00 00 0B C7 00 1C 10 00 00 00 00 6A\r\n11/06/15 10:19:39.413 RECV 23 FF A4 16 03 02\r\n11/06/15 10:19:39.255 RECV 23 E4 9E 81 00 00 01 01 0F 64 14 00 00 00 00 00 00 00 00 15 00 22 00 BA 0B 00 00\r\n11/06/15 10:19:38.959 RECV 3F E4 60 68 68 6E 00 09 99 A8 01 CE 01 00 3F B4 15 00 00 00 00 66 00 00\r\n11/06/15 10:19:38.893 RECV 21 E4 41 6B 00 00 00 06 00 EA 00 F8 2A F8 2A 11 08 00 00 0B C7 00 11 10 00 00 00 00 6A\r\n11/06/15 10:19:38.419 RECV 23 FF A4 16 03 02\r\n11/06/15 10:19:37.969 RECV 3F E4 60 68 68 00 00 09 99 A8 01 9F 01 00 3F E2 07 00 00 00 00 20 00 01\r\n11/06/15 10:19:37.901 RECV 21 E4 41 2C 00 00 00 06 00 EA 00 F8 2A F8 2A 01 08 00 00 0B C7 00 1A 10 00 00 00 00 6A\r\n11/06/15 10:19:37.425 RECV 23 FF A4 16 03 02\r\n11/06/15 10:19:37.003 RECV 3F E4 60 68 68 6E 00 09 99 A8 01 90 01 00 3F C3 11 00 00 00 00 5F 00 01\r\n11/06/15 10:19:36.910 RECV 21 E4 41 64 00 00 00 06 00 EA 00 F8 2A F8 2A 11 08 00 00 0B C7 00 26 10 00 00 00 00 6A\r\n11/06/15 10:19:36.741 RECV 23 E4 9E 81 00 00 01 01 0F 64 14 00 00 00 00 00 00 00 00 15 00 22 00 BA 0B 00 00\r\n11/06/15 10:19:36.433 RECV 23 FF A4 16 03 02\r\n11/06/15 10:19:35.981 RECV 3F E4 60 68 68 00 00 09 99 A8 01 B1 01 00 3F 08 14 00 00 00 00 2D 00 00\r\n11/06/15 10:19:35.914 RECV 21 E4 41 42 00 00 00 06 00 EA 00 F8 2A F8 2A 11 08 00 00 0B C7 00 23 10 00 00 00 00 6A\r\n11/06/15 10:19:35.440 RECV 23 FF A4 16 03 02\r\n11/06/15 10:19:34.989 RECV 3F E4 60 68 68 6E 00 09 99 A8 01 8A 01 00 3F 7C 05 00 00 00 00 67 00 00\r\n11/06/15 10:19:34.923 RECV 21 E4 41 64 00 00 00 06 00 EA 00 F8 2A F8 2A 11 08 00 00 0B C7 00 1E 10 00 00 00 00 6A\r\n11/06/15 10:19:34.446 RECV 23 FF A4 16 03 02\r\n11/06/15 10:19:34.286 RECV 23 E4 9E 81 00 00 01 01 0F 64 14 00 00 00 00 00 00 00 00 15 00 22 00 BA 0B 00 00\r\n11/06/15 10:19:33.992 RECV 3F E4 60 68 68 00 00 09 99 A8 01 A1 01 00 3F 7B 01 00 00 00 00 21 00 01\r\n11/06/15 10:19:33.928 RECV 21 E4 41 3E 00 00 00 06 00 EA 00 F8 2A F8 2A 11 08 00 00 0B C7 00 23 10 00 00 00 00 6A\r\n11/06/15 10:19:33.452 RECV 23 FF A4 16 03 02\r\n11/06/15 10:19:32.998 RECV 3F E4 60 68 68 6E 00 09 99 A8 01 4F 01 00 3F AC 08 00 00 00 00 62 00 01\r\n11/06/15 10:19:32.934 RECV 21 E4 41 60 00 00 00 06 00 EA 00 F8 2A F8 2A 11 08 00 00 0B C7 00 22 10 00 00 00 00 6A\r\n11/06/15 10:19:32.461 RECV 23 FF A4 16 03 02\r\n11/06/15 10:19:32.009 RECV 3F E4 60 68 68 1E 00 09 99 A8 01 BE 01 00 3F 02 1B 00 00 00 00 4E 00 00\r\n11/06/15 10:19:31.942 RECV 21 E4 41 60 00 00 00 06 00 EA 00 F8 2A F8 2A 11 08 00 00 0B C7 00 26 10 00 00 00 00 6A\r\n11/06/15 10:19:31.764 RECV 23 E4 9E 81 00 00 01 01 0F 64 14 00 00 00 00 00 00 00 00 15 00 22 00 BA 0B 00 00\r\n11/06/15 10:19:31.467 RECV 23 FF A4 16 03 02\r\n11/06/15 10:19:31.015 RECV 3F E4 60 68 68 6E 00 09 99 A8 01 45 01 00 3F 43 09 00 00 00 00 50 00 00\r\n11/06/15 10:19:30.949 RECV 21 E4 41 50 00 00 00 06 00 EA 00 F8 2A F8 2A 11 08 00 00 0B C7 00 20 10 00 00 00 00 6A\r\n11/06/15 10:19:30.475 RECV 23 FF A4 16 03 02\r\n11/06/15 10:19:30.026 RECV 3F E4 60 68 68 1E 00 09 99 A8 01 E3 01 00 3F FF 00 00 00 00 00 5B 00 01\r\n11/06/15 10:19:29.956 RECV 21 E4 41 69 00 00 00 06 00 EA 00 F8 2A F8 2A 11 08 00 00 0B C7 00 1C 10 00 00 00 00 6A\r\n11/06/15 10:19:29.481 RECV 23 FF A4 16 03 02\r\n11/06/15 10:19:29.327 RECV 23 E4 9E 81 00 00 01 01 0F 64 14 00 00 00 00 00 00 00 00 15 00 22 00 BA 0B 00 00\r\n11/06/15 10:19:29.030 RECV 3F E4 60 68 68 6E 00 09 99 A8 01 8F 01 00 3F 52 0E 00 00 00 00 4E 00 01\r\n11/06/15 10:19:28.966 RECV 21 E4 41 41 00 00 00 06 00 EA 00 F8 2A F8 2A 11 08 00 00 0B C7 00 1B 10 00 00 00 00 6A\r\n11/06/15 10:19:28.489 RECV 23 FF A4 16 03 02\r\n11/06/15 10:19:28.038 RECV 3F E4 60 68 68 6E 00 09 99 A8 01 07 02 00 3E 10 15 00 00 00 00 66 00 00\r\n11/06/15 10:19:27.973 RECV 21 E4 41 67 00 00 00 06 00 EA 00 F8 2A F8 2A 11 08 00 00 0B C7 00 1A 10 00 00 00 00 6A\r\n11/06/15 10:19:27.494 RECV 23 FF A4 16 03 02\r\n11/06/15 10:19:27.042 RECV 3F E4 60 68 68 6E 00 09 99 A8 01 CD 01 00 3E F4 25 00 00 00 00 1A 00 00\r\n11/06/15 10:19:26.977 RECV 21 E4 41 43 00 00 00 06 00 EA 00 F8 2A F8 2A 11 08 00 00 0B C7 00 20 10 00 00 00 00 6A\r\n11/06/15 10:19:26.798 RECV 23 E4 9E 81 00 00 01 01 0F 64 14 00 00 00 00 00 00 00 00 15 00 22 00 BA 0B 00 00\r\n11/06/15 10:19:26.502 RECV 23 FF A4 16 03 02\r\n11/06/15 10:19:26.049 RECV 3F E4 60 68 68 6E 00 09 99 A8 01 DE 01 00 3E FE 04 00 00 00 00 65 00 01\r\n11/06/15 10:19:25.983 RECV 21 E4 41 62 00 00 00 06 00 EA 00 F8 2A F8 2A 11 08 00 00 0B C7 00 10 10 00 00 00 00 6B\r\n11/06/15 10:19:25.508 RECV 23 FF A4 16 03 02\r\n11/06/15 10:19:25.058 RECV 3F E4 60 68 68 6E 00 09 99 A8 01 57 02 00 3E E4 0C 00 00 00 00 6E 00 00\r\n11/06/15 10:19:24.991 RECV 21 E4 41 71 00 00 00 06 00 EA 00 F8 2A F8 2A 11 08 00 00 0B C7 00 19 10 00 00 00 00 6B\r\n11/06/15 10:19:24.516 RECV 23 FF A4 16 03 02\r\n11/06/15 10:19:24.356 RECV 23 E4 9E 81 00 00 01 01 0F 64 14 00 00 00 00 00 00 00 00 15 00 22 00 BA 0B 00 00\r\n11/06/15 10:19:24.061 RECV 3F E4 60 68 68 6E 00 09 99 A8 01 AE 01 00 3E 65 10 00 00 00 00 40 00 00\r\n11/06/15 10:19:23.995 RECV 21 E4 41 33 00 00 00 06 00 EA 00 F8 2A F8 2A 11 08 00 00 0B C7 00 1B 10 00 00 00 00 6A\r\n11/06/15 10:19:23.522 RECV 23 FF A4 16 03 02\r\n11/06/15 10:19:23.072 RECV 3F E4 60 68 68 6E 00 09 99 A8 01 9F 01 00 3E D7 0F 00 00 00 00 6C 00 01\r\n11/06/15 10:19:23.004 RECV 21 E4 41 6A 00 00 00 06 00 EA 00 F8 2A F8 2A 11 08 00 00 0B C7 00 19 10 00 00 00 00 6A\r\n11/06/15 10:19:22.529 RECV 23 FF A4 16 03 02\r\n11/06/15 10:19:22.077 RECV 3F E4 60 68 68 00 00 09 99 A8 01 75 01 00 3E F5 06 00 00 00 00 25 00 00\r\n11/06/15 10:19:22.011 RECV 21 E4 41 2E 00 00 00 06 00 EA 00 F8 2A F8 2A 01 08 00 00 0B C7 00 1D 10 00 00 00 00 68\r\n11/06/15 10:19:21.834 RECV 23 E4 9E 81 00 00 01 01 0F 64 14 00 00 00 00 00 00 00 00 15 00 22 00 BA 0B 00 00\r\n11/06/15 10:19:21.538 RECV 23 FF A4 16 03 02\r\n11/06/15 10:19:21.228 RECV 3F E4 60 68 68 6E 00 09 99 A8 01 81 01 00 3E 4A 05 00 00 00 00 69 00 00\r\n11/06/15 10:19:21.021 RECV 21 E4 41 64 00 00 00 06 00 EA 00 F8 2A F8 2A 11 08 00 00 1B C7 00 18 10 00 00 00 00 68\r\n11/06/15 10:19:20.544 RECV 23 FF A4 16 03 02\r\n11/06/15 10:19:20.090 RECV 3F E4 60 68 68 00 00 09 99 A8 01 7B 01 00 3E 22 13 00 00 00 00 25 00 01\r\n11/06/15 10:19:20.027 RECV 21 E4 41 3E 00 00 00 06 00 EA 00 F8 2A F8 2A 11 08 00 00 1B C7 00 19 10 00 00 00 00 68\r\n11/06/15 10:19:19.550 RECV 23 FF A4 16 03 02\r\n11/06/15 10:19:19.396 RECV 23 E4 9E 81 00 00 01 01 0F 64 14 00 00 00 00 00 00 00 00 15 00 22 00 BA 0B 00 00\r\n11/06/15 10:19:19.034 RECV 21 E4 41 61 00 00 00 06 00 EA 00 F8 2A F8 2A 11 08 00 00 1B C7 00 16 10 00 00 00 00 68\r\n11/06/15 10:19:18.562 RECV 23 FF A4 16 03 02\r\n11/06/15 10:19:18.126 RECV 3F E4 60 68 68 00 00 09 99 A8 01 A0 01 00 3E F1 0E 00 00 00 00 3B 00 00\r\n11/06/15 10:19:18.059 RECV 21 E4 41 46 00 00 00 06 00 EA 00 F8 2A F8 2A 11 08 00 00 1B C7 00 1B 10 00 00 00 00 68\r\n11/06/15 10:19:17.566 RECV 23 FF A4 16 03 02\r\n11/06/15 10:19:17.150 RECV 23 FF 74 0A 64 72 74 53 61 74 44 72 77 50 6E 4D 31 20 36 31 31\r\n11/06/15 10:19:17.117 RECV 3F E4 60 68 68 6E 00 09 99 A8 01 6E 01 00 3E 31 0C 00 00 00 00 5F 00 00\r\n11/06/15 10:19:17.047 RECV 21 E4 41 5C 00 00 00 06 00 EA 00 F8 2A F8 2A 11 08 00 00 1B C7 00 1D 10 00 00 00 00 68\r\n11/06/15 10:19:16.868 RECV 23 E4 9E 81 00 00 01 01 0F 64 14 00 00 00 00 00 00 00 00 15 00 22 00 BA 0B 00 00\r\n11/06/15 10:19:16.571 RECV 23 FF A4 16 03 02\r\n11/06/15 10:19:16.119 RECV 3F E4 60 68 68 1E 00 09 99 A8 01 04 02 00 3E 95 1A 00 00 00 00 3E 00 01\r\n11/06/15 10:19:16.053 RECV 21 E4 41 62 00 00 00 06 00 EA 00 F8 2A F8 2A 11 08 00 00 1B C7 00 23 10 00 00 00 00 68\r\n11/06/15 10:19:15.578 RECV 23 FF A4 16 03 02\r\n11/06/15 10:19:15.126 RECV 3F E4 60 68 68 6E 00 09 99 A8 01 56 01 00 3E F5 08 00 00 00 00 5D 00 01\r\n11/06/15 10:19:15.061 RECV 21 E4 41 57 00 00 00 06 00 EA 00 F8 2A F8 2A 11 08 00 00 1B C7 00 18 10 00 00 00 00 68\r\n11/06/15 10:19:14.586 RECV 23 FF A4 16 03 02\r\n11/06/15 10:19:14.432 RECV 23 E4 9E 81 00 00 01 01 0F 64 14 00 00 00 00 00 00 00 00 15 00 22 00 BA 0B 00 00\r\n11/06/15 10:19:14.135 RECV 3F E4 60 68 68 1E 00 09 99 A8 01 FA 01 00 3E A3 03 00 00 00 00 6A 00 00\r\n11/06/15 10:19:14.067 RECV 21 E4 41 6A 00 00 00 06 00 EA 00 F8 2A F8 2A 11 08 00 00 1B C7 00 1E 10 00 00 00 00 68\r\n11/06/15 10:19:13.591 RECV 23 FF A4 16 03 02\r\n11/06/15 10:19:13.141 RECV 3F E4 60 68 68 6E 00 09 99 A8 01 43 01 00 3E 9A 07 00 00 00 00 59 00 00\r\n11/06/15 10:19:13.075 RECV 21 E4 41 4C 00 00 00 06 00 EA 00 F8 2A F8 2A 11 08 00 00 1B C7 00 1D 10 00 00 00 00 68\r\n11/06/15 10:19:12.599 RECV 23 FF A4 16 03 02\r\n11/06/15 10:19:12.144 RECV 3F E4 60 68 68 6E 00 09 99 A8 01 D3 01 00 3E 8A 2A 00 00 00 00 7A 00 01\r\n11/06/15 10:19:12.080 RECV 21 E4 41 6F 00 00 00 06 00 EA 00 F8 2A F8 2A 11 08 00 00 1B C7 00 1E 10 00 00 00 00 68\r\n11/06/15 10:19:11.897 RECV 23 E4 9E 81 00 00 01 01 0F 64 14 00 00 00 00 00 00 00 00 15 00 22 00 BA 0B 00 00\r\n11/06/15 10:19:11.603 RECV 23 FF A4 16 03 02\r\n11/06/15 10:19:11.152 RECV 3F E4 60 68 68 6E 00 09 99 A8 01 07 01 00 3E BD 12 00 00 00 00 3F 00 01\r\n11/06/15 10:19:11.088 RECV 21 E4 41 19 00 00 00 06 00 EA 00 F8 2A F8 2A 01 08 00 00 1B C7 00 1E 10 00 00 00 00 68\r\n11/06/15 10:19:10.614 RECV 23 FF A4 16 03 02\r\n11/06/15 10:19:10.162 RECV 3F E4 60 68 68 6E 00 09 99 A8 01 D5 01 00 3E 58 02 00 00 00 00 68 00 00\r\n11/06/15 10:19:10.096 RECV 21 E4 41 6D 00 00 00 06 00 EA 00 F8 2A F8 2A 11 08 00 00 1B C7 00 19 10 00 00 00 00 68\r\n11/06/15 10:19:09.620 RECV 23 FF A4 16 03 02\r\n11/06/15 10:19:09.465 RECV 23 E4 9E 81 00 00 01 01 0F 64 14 00 00 00 00 00 00 00 00 15 00 22 00 BA 0B 00 00\r\n11/06/15 10:19:09.169 RECV 3F E4 60 68 68 6E 00 09 99 A8 01 31 01 00 3E E1 30 00 00 00 00 34 00 00\r\n11/06/15 10:19:09.102 RECV 21 E4 41 1E 00 00 00 06 00 EA 00 F8 2A F8 2A 01 08 00 00 1B C7 00 1E 10 00 00 00 00 68\r\n11/06/15 10:19:08.627 RECV 23 FF A4 16 03 02\r\n11/06/15 10:19:08.210 RECV 3F E4 60 68 68 6E 00 09 99 A8 01 F6 01 00 3E 2D 30 00 00 00 00 77 00 01\r\n11/06/15 10:19:08.145 RECV 21 E4 41 6A 00 00 00 06 00 EA 00 F8 2A F8 2A 11 08 00 00 1B C7 00 1C 10 00 00 00 00 68\r\n11/06/15 10:19:07.633 RECV 23 FF A4 16 03 02\r\n11/06/15 10:19:07.181 RECV 3F E4 60 68 68 6E 00 09 99 A8 01 30 01 00 3E F5 04 00 00 00 00 09 00 01\r\n11/06/15 10:19:07.116 RECV 21 E4 41 21 00 00 00 06 00 EA 00 F8 2A F8 2A 01 08 00 00 1B C7 00 1B 10 00 00 00 00 68\r\n11/06/15 10:19:06.937 RECV 23 E4 9E 81 00 00 01 01 0F 64 14 00 00 00 00 00 00 00 00 15 00 22 00 BA 0B 00 00\r\n11/06/15 10:19:06.640 RECV 23 FF A4 16 03 02\r\n11/06/15 10:19:06.204 RECV 3F E4 60 68 68 6E 00 09 99 A8 01 DA 01 00 3E C4 09 00 00 00 00 6C 00 00\r\n11/06/15 10:19:06.121 RECV 21 E4 41 6C 00 00 00 06 00 EA 00 F8 2A F8 2A 11 08 00 00 1B C7 00 12 10 00 00 00 00 68\r\n11/06/15 10:19:05.647 RECV 23 FF A4 16 03 02\r\n11/06/15 10:19:05.196 RECV 3F E4 60 68 68 6E 00 09 99 A8 01 53 01 00 3E 59 02 00 00 00 00 10 00 00\r\n11/06/15 10:19:05.130 RECV 21 E4 41 24 00 00 00 06 00 EA 00 F8 2A F8 2A 01 08 00 00 1B C7 00 16 10 00 00 00 00 68\r\n11/06/15 10:19:04.654 RECV 23 FF A4 16 03 02\r\n11/06/15 10:19:04.498 RECV 23 E4 9E 81 00 00 01 01 0F 64 14 00 00 00 00 00 00 00 00 15 00 22 00 BA 0B 00 00\r\n11/06/15 10:19:04.201 RECV 3F E4 60 68 68 6E 00 09 99 A8 01 BC 01 00 3E AA 00 00 00 00 00 6E 00 01\r\n11/06/15 10:19:04.136 RECV 21 E4 41 6B 00 00 00 06 00 EA 00 F8 2A F8 2A 11 08 00 00 1B C7 00 1F 10 00 00 00 00 68\r\n11/06/15 10:19:03.661 RECV 23 FF A4 16 03 02\r\n11/06/15 10:19:03.209 RECV 3F E4 60 68 68 00 00 09 99 A8 01 3B 01 00 3E 4D 02 00 00 00 00 14 00 00\r\n11/06/15 10:19:03.143 RECV 21 E4 41 2C 00 00 00 06 00 EA 00 F8 2A F8 2A 01 08 00 00 1B C7 00 1C 10 00 00 00 00 68\r\n11/06/15 10:19:02.668 RECV 23 FF A4 16 03 02\r\n11/06/15 10:19:02.216 RECV 3F E4 60 68 68 6E 00 09 99 A8 01 B1 01 00 3E 5D 01 00 00 00 00 65 00 00\r\n11/06/15 10:19:02.150 RECV 21 E4 41 65 00 00 00 06 00 EA 00 F8 2A F8 2A 11 08 00 00 1B C7 00 19 10 00 00 00 00 68\r\n11/06/15 10:19:01.973 RECV 23 E4 9E 81 00 00 01 01 0F 64 14 00 00 00 00 00 00 00 00 15 00 22 00 BA 0B 00 00\r\n11/06/15 10:19:01.676 RECV 23 FF A4 16 03 02\r\n11/06/15 10:19:01.259 RECV 3F E4 60 68 68 00 00 09 99 A8 01 54 01 00 3E CC 03 00 00 00 00 1A 00 01\r\n11/06/15 10:19:01.192 RECV 21 E4 41 35 00 00 00 06 00 EA 00 F8 2A F8 2A 11 08 00 00 1B C7 00 1C 10 00 00 00 00 68\r\n11/06/15 10:19:00.683 RECV 23 FF A4 16 03 02\r\n11/06/15 10:19:00.249 RECV 3F E4 60 68 68 6E 00 09 99 A8 01 73 01 00 3E 48 06 00 00 00 00 66 00 01\r\n11/06/15 10:19:00.166 RECV 21 E4 41 65 00 00 00 06 00 EA 00 F8 2A F8 2A 11 08 00 00 1B C7 00 18 10 00 00 00 00 68\r\n11/06/15 10:18:59.536 RECV 23 E4 9E 81 00 00 01 01 0F 64 14 00 00 00 00 00 00 00 00 15 00 22 00 BA 0B 00 00\r\n11/06/15 10:18:59.239 RECV 3F E4 60 68 68 00 00 09 99 A8 01 79 01 00 3D C1 0F 00 00 00 00 2D 00 00\r\n11/06/15 10:18:59.173 RECV 21 E4 41 3F 00 00 00 06 00 EA 00 F8 2A F8 2A 11 08 00 00 1B C7 00 1A 10 00 00 00 00 68\r\n11/06/15 10:18:58.695 RECV 23 FF A4 16 03 02\r\n11/06/15 10:18:58.248 RECV 3F E4 60 68 68 6E 00 09 99 A8 01 7A 01 00 3D 4A 08 00 00 00 00 62 00 00\r\n11/06/15 10:18:58.178 RECV 21 E4 41 5F 00 00 00 06 00 EA 00 F8 2A F8 2A 11 08 00 00 1B C7 00 1C 10 00 00 00 00 68\r\n11/06/15 10:18:57.702 RECV 23 FF A4 16 03 02\r\n11/06/15 10:18:57.250 RECV 3F E4 60 68 68 00 00 09 99 A8 01 CC 01 00 3D F4 23 00 00 00 00 39 00 01\r\n11/06/15 10:18:57.184 RECV 21 E4 41 50 00 00 00 06 00 EA 00 F8 2A F8 2A 11 08 00 00 1B C7 00 1F 10 00 00 00 00 68\r\n11/06/15 10:18:57.008 RECV 23 E4 9E 81 00 00 01 01 0F 64 14 00 00 00 00 00 00 00 00 15 00 22 00 BA 0B 00 00\r\n11/06/15 10:18:56.710 RECV 23 FF A4 16 03 02\r\n11/06/15 10:18:56.260 RECV 3F E4 60 68 68 6E 00 09 99 A8 01 7E 01 00 3D E2 00 00 00 00 00 68 00 01\r\n11/06/15 10:18:56.193 RECV 21 E4 41 60 00 00 00 06 00 EA 00 F8 2A F8 2A 11 08 00 00 1B C7 00 19 10 00 00 00 00 68\r\n11/06/15 10:18:55.717 RECV 23 FF A4 16 03 02\r\n11/06/15 10:18:55.264 RECV 3F E4 60 68 68 1E 00 09 99 A8 01 F7 01 00 3D 6C 24 00 00 00 00 56 00 00\r\n11/06/15 10:18:55.199 RECV 21 E4 41 58 00 00 00 06 00 EA 00 F8 2A F8 2A 11 08 00 00 1B C7 00 1D 10 00 00 00 00 68\r\n11/06/15 10:18:54.724 RECV 23 FF A4 16 03 02\r\n11/06/15 10:18:54.569 RECV 23 E4 9E 81 00 00 01 01 0F 64 14 00 00 00 00 00 00 00 00 15 00 22 00 BA 0B 00 00\r\n11/06/15 10:18:54.271 RECV 3F E4 60 68 68 6E 00 09 99 A8 01 6F 01 00 3D 41 03 00 00 00 00 5B 00 00\r\n11/06/15 10:18:54.204 RECV 21 E4 41 54 00 00 00 06 00 EA 00 F8 2A F8 2A 11 08 00 00 1B C7 00 19 10 00 00 00 00 68\r\n11/06/15 10:18:53.730 RECV 23 FF A4 16 03 02\r\n11/06/15 10:18:53.711 RECV 3F E4 60 68 68 1E 00 09 99 A8 01 F6 01 00 3D D3 1E 00 00 00 00 5A 00 01\r\n11/06/15 10:18:53.214 RECV 21 E4 41 68 00 00 00 06 00 EA 00 F8 2A F8 2A 11 08 00 00 1B C7 00 1B 10 00 00 00 00 68\r\n11/06/15 10:18:52.737 RECV 23 FF A4 16 03 02\r\n11/06/15 10:18:52.286 RECV 3F E4 60 68 68 6E 00 09 99 A8 01 36 01 00 3D C4 02 00 00 00 00 56 00 01\r\n11/06/15 10:18:52.220 RECV 21 E4 41 4A 00 00 00 06 00 EA 00 F8 2A F8 2A 11 08 00 00 1B C7 00 15 10 00 00 00 00 68\r\n11/06/15 10:18:52.040 RECV 23 E4 9E 81 00 00 01 01 0F 64 14 00 00 00 00 00 00 00 00 15 00 22 00 BA 0B 00 00\r\n11/06/15 10:18:51.745 RECV 23 FF A4 16 03 02\r\n11/06/15 10:18:51.295 RECV 3F E4 60 68 68 6E 00 09 99 A8 01 04 02 00 3D 5D 17 00 00 00 00 6F 00 00\r\n11/06/15 10:18:51.227 RECV 21 E4 41 6D 00 00 00 06 00 EA 00 F8 2A F8 2A 11 08 00 00 1B C7 00 1B 10 00 00 00 00 6A\r\n11/06/15 10:18:50.751 RECV 23 FF A4 16 03 02\r\n11/06/15 10:18:50.300 RECV 3F E4 60 68 68 6E 00 09 99 A8 01 29 01 00 3D D6 05 00 00 00 00 47 00 00\r\n11/06/15 10:18:50.233 RECV 21 E4 41 22 00 00 00 06 00 EA 00 F8 2A F8 2A 01 08 00 00 1B C7 00 19 10 00 00 00 00 6A\r\n11/06/15 10:18:49.757 RECV 23 FF A4 16 03 02\r\n11/06/15 10:18:49.597 RECV 23 E4 9E 81 00 00 01 01 0F 64 14 00 00 00 00 00 00 00 00 15 00 22 00 BA 0B 00 00\r\n11/06/15 10:18:49.303 RECV 3F E4 60 68 68 6E 00 09 99 A8 01 AD 01 00 3D 96 07 00 00 00 00 6F 00 01\r\n11/06/15 10:18:49.239 RECV 21 E4 41 6A 00 00 00 06 00 EA 00 F8 2A F8 2A 11 08 00 00 1B C7 00 1E 10 00 00 00 00 6A\r\n11/06/15 10:18:48.764 RECV 23 FF A4 16 03 02\r\n11/06/15 10:18:48.311 RECV 3F E4 60 68 68 6E 00 09 99 A8 01 F7 00 00 3D CE 09 00 00 00 00 31 00 01\r\n11/06/15 10:18:48.245 RECV 21 E4 41 19 00 00 00 06 00 EA 00 F8 2A F8 2A 01 08 00 00 1B C7 00 1D 10 00 00 00 00 6A\r\n11/06/15 10:18:47.773 RECV 23 FF A4 16 03 02\r\n11/06/15 10:18:47.319 RECV 3F E4 60 68 68 6E 00 09 99 A8 01 AC 01 00 3D 8D 07 00 00 00 00 69 00 00\r\n11/06/15 10:18:47.255 RECV 21 E4 41 69 00 00 00 06 00 EA 00 F8 2A F8 2A 11 08 00 00 1B C7 00 1E 10 00 00 00 00 6A\r\n11/06/15 10:18:47.074 RECV 23 E4 9E 81 00 00 01 01 0F 64 14 00 00 00 00 00 00 00 00 15 00 22 00 BA 0B 00 00\r\n11/06/15 10:18:46.778 RECV 23 FF A4 16 03 02\r\n11/06/15 10:18:46.327 RECV 3F E4 60 68 68 6E 00 09 99 A8 01 3D 01 00 3D D0 03 00 00 00 00 09 00 00\r\n11/06/15 10:18:46.263 RECV 21 E4 41 1C 00 00 00 06 00 EA 00 F8 2A F8 2A 01 08 00 00 1B C7 00 26 10 00 00 00 00 6A\r\n11/06/15 10:18:45.785 RECV 23 FF A4 16 03 02\r\n11/06/15 10:18:45.334 RECV 3F E4 60 68 68 6E 00 09 99 A8 01 C9 01 00 3D 14 07 00 00 00 00 69 00 01\r\n11/06/15 10:18:45.268 RECV 21 E4 41 6C 00 00 00 06 00 EA 00 F8 2A F8 2A 11 08 00 00 1B C7 00 24 10 00 00 00 00 6A\r\n11/06/15 10:18:44.792 RECV 23 FF A4 16 03 02\r\n11/06/15 10:18:44.639 RECV 23 E4 9E 81 00 00 01 01 0F 64 14 00 00 00 00 00 00 00 00 15 00 22 00 BA 0B 00 00\r\n11/06/15 10:18:44.343 RECV 3F E4 60 68 68 6E 00 09 99 A8 01 18 01 00 3D 72 06 00 00 00 00 13 00 01\r\n11/06/15 10:18:44.275 RECV 21 E4 41 20 00 00 00 06 00 EA 00 F8 2A F8 2A 01 08 00 00 1B C7 00 1E 10 00 00 00 00 6A\r\n11/06/15 10:18:43.800 RECV 23 FF A4 16 03 02\r\n11/06/15 10:18:43.375 RECV 3F E4 60 68 68 6E 00 09 99 A8 01 DA 01 00 3D 5F 04 00 00 00 00 6D 00 00\r\n11/06/15 10:18:43.283 RECV 21 E4 41 67 00 00 00 06 00 EA 00 F8 2A F8 2A 11 08 00 00 1B C7 00 10 10 00 00 00 00 6A\r\n11/06/15 10:18:42.806 RECV 23 FF A4 16 03 02\r\n11/06/15 10:18:42.454 RECV 3F E4 60 68 68 00 00 09 99 A8 01 3D 01 00 3D 3B 02 00 00 00 00 14 00 01\r\n11/06/15 10:18:42.359 RECV 21 E4 41 29 00 00 00 06 00 EA 00 F8 2A F8 2A 01 08 00 00 1B C7 00 18 10 00 00 00 00 6A\r\n11/06/15 10:18:42.110 RECV 23 E4 9E 81 00 00 01 01 0F 64 14 00 00 00 00 00 00 00 00 15 00 22 00 BA 0B 00 00\r\n11/06/15 10:18:41.814 RECV 23 FF A4 16 03 02\r\n11/06/15 10:18:41.397 RECV 3F E4 60 68 68 6E 00 09 99 A8 01 84 01 00 3D 06 08 00 00 00 00 67 00 01\r\n11/06/15 10:18:41.332 RECV 21 E4 41 69 00 00 00 06 00 EA 00 F8 2A F8 2A 11 08 00 00 1B C7 00 22 10 00 00 00 00 6A\r\n11/06/15 10:18:40.821 RECV 23 FF A4 16 03 02\r\n11/06/15 10:18:40.370 RECV 3F E4 60 68 68 00 00 09 99 A8 01 7F 01 00 3D 00 04 00 00 00 00 27 00 00\r\n11/06/15 10:18:40.302 RECV 21 E4 41 39 00 00 00 06 00 EA 00 F8 2A F8 2A 11 08 00 00 1B C7 00 16 10 00 00 00 00 6B\r\n11/06/15 10:18:39.828 RECV 23 FF A4 16 03 02\r\n11/06/15 10:18:39.655 RECV 23 E4 9E 81 00 00 01 01 0F 64 14 00 00 00 00 00 00 00 00 15 00 22 00 BA 0B 00 00\r\n11/06/15 10:18:39.359 RECV 3F E4 60 68 68 6E 00 09 99 A8 01 9A 01 00 3D 5D 04 00 00 00 00 66 00 00\r\n11/06/15 10:18:39.324 RECV 21 E4 41 66 00 00 00 06 00 EA 00 F8 2A F8 2A 11 08 00 00 1B C7 00 0D 10 00 00 00 00 6A\r\n11/06/15 10:18:38.834 RECV 23 FF A4 16 03 02\r\n11/06/15 10:18:38.384 RECV 3F E4 60 68 68 00 00 09 99 A8 01 A1 01 00 3D 99 24 00 00 00 00 2F 00 01\r\n11/06/15 10:18:38.318 RECV 21 E4 41 3E 00 00 00 06 00 EA 00 F8 2A F8 2A 11 08 00 00 1B C7 00 19 10 00 00 00 00 6A\r\n11/06/15 10:18:37.842 RECV 23 FF A4 16 03 02\r\n11/06/15 10:18:37.389 RECV 3F E4 60 68 68 6E 00 09 99 A8 01 88 01 00 3D 52 0B 00 00 00 00 63 00 01\r\n11/06/15 10:18:37.323 RECV 21 E4 41 61 00 00 00 06 00 EA 00 F8 2A F8 2A 11 08 00 00 1B C7 00 21 10 00 00 00 00 6A\r\n11/06/15 10:18:37.145 RECV 23 E4 9E 81 00 00 01 01 0F 64 14 00 00 00 00 00 00 00 00 15 00 22 00 BA 0B 00 00\r\n11/06/15 10:18:36.848 RECV 23 FF A4 16 03 02\r\n11/06/15 10:18:36.396 RECV 3F E4 60 68 68 00 00 09 99 A8 01 E7 01 00 3D C2 06 00 00 00 00 43 00 00\r\n11/06/15 10:18:36.331 RECV 21 E4 41 4F 00 00 00 06 00 EA 00 F8 2A F8 2A 11 08 00 00 1B C7 00 20 10 00 00 00 00 6A\r\n11/06/15 10:18:35.854 RECV 23 FF A4 16 03 02\r\n11/06/15 10:18:35.430 RECV 3F E4 60 68 68 6E 00 09 99 A8 01 80 01 00 3C 95 12 00 00 00 00 57 00 00\r\n11/06/15 10:18:35.337 RECV 21 E4 41 5C 00 00 00 06 00 EA 00 F8 2A F8 2A 11 08 00 00 1B C7 00 1C 10 00 00 00 00 6A\r\n11/06/15 10:18:34.862 RECV 23 FF A4 16 03 02\r\n11/06/15 10:18:34.705 RECV 23 E4 9E 81 00 00 01 01 0F 64 14 00 00 00 00 00 00 00 00 15 00 22 00 BA 0B 00 00\r\n11/06/15 10:18:34.410 RECV 3F E4 60 68 68 1E 00 09 99 A8 01 F6 01 00 3C 1C 0C 00 00 00 00 58 00 01\r\n11/06/15 10:18:34.344 RECV 21 E4 41 61 00 00 00 06 00 EA 00 F8 2A F8 2A 11 08 00 00 1B C7 00 1D 10 00 00 00 00 6A\r\n11/06/15 10:18:33.870 RECV 23 FF A4 16 03 02\r\n11/06/15 10:18:33.417 RECV 3F E4 60 68 68 6E 00 09 99 A8 01 B5 01 00 3C B9 06 00 00 00 00 55 00 01\r\n11/06/15 10:18:33.351 RECV 21 E4 41 51 00 00 00 06 00 EA 00 F8 2A F8 2A 11 08 00 00 1B C7 00 1E 10 00 00 00 00 6A\r\n11/06/15 10:18:32.876 RECV 23 FF A4 16 03 02\r\n11/06/15 10:18:32.423 RECV 3F E4 60 68 68 6E 00 09 99 A8 01 FB 01 00 3C 5B 00 00 00 00 00 6B 00 00\r\n11/06/15 10:18:32.357 RECV 21 E4 41 6A 00 00 00 06 00 EA 00 F8 2A F8 2A 11 08 00 00 1B C7 00 15 10 00 00 00 00 6A\r\n11/06/15 10:18:32.192 RECV 23 E4 9E 81 00 00 01 01 0F 64 14 00 00 00 00 00 00 00 00 15 00 22 00 BA 0B 00 00\r\n11/06/15 10:18:31.882 RECV 23 FF A4 16 03 02\r\n11/06/15 10:18:31.432 RECV 3F E4 60 68 68 6E 00 09 99 A8 01 C1 01 00 3C F5 2F 00 00 00 00 0F 00 00\r\n11/06/15 10:18:31.366 RECV 21 E4 41 2F 00 00 00 06 00 EA 00 F8 2A F8 2A 01 08 00 00 1B C7 00 1B 10 00 00 00 00 6A\r\n11/06/15 10:18:30.890 RECV 23 FF A4 16 03 02\r\n11/06/15 10:18:30.437 RECV 3F E4 60 68 68 6E 00 09 99 A8 01 8D 01 00 3C 7F 0C 00 00 00 00 60 00 01\r\n11/06/15 10:18:30.372 RECV 21 E4 41 61 00 00 00 06 00 EA 00 F8 2A F8 2A 11 08 00 00 1B C7 00 1C 10 00 00 00 00 6A\r\n11/06/15 10:18:29.896 RECV 23 FF A4 16 03 02\r\n11/06/15 10:18:29.741 RECV 23 E4 9E 81 00 00 01 01 0F 64 14 00 00 00 00 00 00 00 00 15 00 22 00 BA 0B 00 00\r\n11/06/15 10:18:29.446 RECV 3F E4 60 68 68 6E 00 09 99 A8 01 E7 01 00 3C DC 03 00 00 00 00 72 00 00\r\n11/06/15 10:18:29.379 RECV 21 E4 41 70 00 00 00 06 00 EA 00 F8 2A F8 2A 11 08 00 00 1B C7 00 17 10 00 00 00 00 6A\r\n11/06/15 10:18:28.903 RECV 23 FF A4 16 03 02\r\n11/06/15 10:18:28.451 RECV 3F E4 60 68 68 6E 00 09 99 A8 01 83 01 00 3C 97 24 00 00 00 00 3D 00 00\r\n11/06/15 10:18:28.385 RECV 21 E4 41 25 00 00 00 06 00 EA 00 F8 2A F8 2A 01 08 00 00 1B C7 00 1B 10 00 00 00 00 6A\r\n11/06/15 10:18:27.911 RECV 23 FF A4 16 03 02\r\n11/06/15 10:18:27.491 RECV 3F E4 60 68 68 6E 00 09 99 A8 01 78 01 00 3C E9 15 00 00 00 00 65 00 01\r\n11/06/15 10:18:27.426 RECV 21 E4 41 69 00 00 00 06 00 EA 00 F8 2A F8 2A 11 08 00 00 1B C7 00 15 10 00 00 00 00 6A\r\n11/06/15 10:18:27.209 RECV 23 E4 9E 81 00 00 01 01 0F 64 14 00 00 00 00 00 00 00 00 15 00 22 00 BA 0B 00 00\r\n11/06/15 10:18:26.914 RECV 23 FF A4 16 03 02\r\n11/06/15 10:18:26.461 RECV 3F E4 60 68 68 00 00 09 99 A8 01 31 01 00 3C EE 03 00 00 00 00 1A 00 00\r\n11/06/15 10:18:26.398 RECV 21 E4 41 2E 00 00 00 06 00 EA 00 F8 2A F8 2A 01 08 00 00 1B C7 00 20 10 00 00 00 00 6A\r\n11/06/15 10:18:25.924 RECV 23 FF A4 16 03 02\r\n11/06/15 10:18:25.506 RECV 3F E4 60 68 68 6E 00 09 99 A8 01 5F 01 00 3C A1 00 00 00 00 00 66 00 00\r\n11/06/15 10:18:25.442 RECV 21 E4 41 68 00 00 00 06 00 EA 00 F8 2A F8 2A 11 08 00 00 1B C7 00 1A 10 00 00 00 00 6A\r\n11/06/15 10:18:24.932 RECV 23 FF A4 16 03 02\r\n11/06/15 10:18:24.777 RECV 23 E4 9E 81 00 00 01 01 0F 64 14 00 00 00 00 00 00 00 00 15 00 22 00 BA 0B 00 00\r\n11/06/15 10:18:24.480 RECV 3F E4 60 68 68 00 00 09 99 A8 01 40 01 00 3C B8 09 00 00 00 00 20 00 01\r\n11/06/15 10:18:24.413 RECV 21 E4 41 39 00 00 00 06 00 EA 00 F8 2A F8 2A 11 08 00 00 1B C7 00 1A 10 00 00 00 00 6A\r\n11/06/15 10:18:23.938 RECV 23 FF A4 16 03 02\r\n11/06/15 10:18:23.487 RECV 3F E4 60 68 68 6E 00 09 99 A8 01 47 01 00 3C 03 0C 00 00 00 00 69 00 01\r\n11/06/15 10:18:23.421 RECV 21 E4 41 67 00 00 00 06 00 EA 00 F8 2A F8 2A 11 08 00 00 1B C7 00 18 10 00 00 00 00 6A\r\n11/06/15 10:18:22.946 RECV 23 FF A4 16 03 02\r\n11/06/15 10:18:22.521 RECV 3F E4 60 68 68 00 00 09 99 A8 01 5F 01 00 3C F7 0A 00 00 00 00 30 00 00\r\n11/06/15 10:18:22.426 RECV 21 E4 41 47 00 00 00 06 00 EA 00 F8 2A F8 2A 11 08 00 00 1B C7 00 18 10 00 00 00 00 6A\r\n11/06/15 10:18:22.249 RECV 23 E4 9E 81 00 00 01 01 0F 64 14 00 00 00 00 00 00 00 00 15 00 22 00 BA 0B 00 00\r\n11/06/15 10:18:21.952 RECV 23 FF A4 16 03 02\r\n11/06/15 10:18:21.501 RECV 3F E4 60 68 68 6E 00 09 99 A8 01 4F 01 00 3C C1 0A 00 00 00 00 60 00 00\r\n11/06/15 10:18:21.434 RECV 21 E4 41 60 00 00 00 06 00 EA 00 F8 2A F8 2A 11 08 00 00 1B C7 00 16 10 00 00 00 00 68\r\n11/06/15 10:18:20.959 RECV 23 FF A4 16 03 02\r\n11/06/15 10:18:20.508 RECV 3F E4 60 68 68 1E 00 09 99 A8 01 4D 01 00 3C 2D 07 00 00 00 00 3A 00 01\r\n11/06/15 10:18:20.442 RECV 21 E4 41 4F 00 00 00 06 00 EA 00 F8 2A F8 2A 11 08 00 00 1B C7 00 19 10 00 00 00 00 68\r\n11/06/15 10:18:19.966 RECV 23 FF A4 16 03 02\r\n11/06/15 10:18:19.812 RECV 23 E4 9E 81 00 00 01 01 0F 64 14 00 00 00 00 00 00 00 00 15 00 22 00 BA 0B 00 00\r\n11/06/15 10:18:19.515 RECV 3F E4 60 68 68 6E 00 09 99 A8 01 27 01 00 3C 48 07 00 00 00 00 61 00 01\r\n11/06/15 10:18:19.449 RECV 21 E4 41 61 00 00 00 06 00 EA 00 F8 2A F8 2A 11 08 00 00 1B C7 00 13 10 00 00 00 00 68\r\n11/06/15 10:18:18.977 RECV 23 FF A4 16 03 02\r\n11/06/15 10:18:18.526 RECV 3F E4 60 68 68 1E 00 09 99 A8 01 A4 01 00 3C F4 08 00 00 00 00 59 00 00\r\n11/06/15 10:18:18.465 RECV 21 E4 41 61 00 00 00 06 00 EA 00 F8 2A F8 2A 11 08 00 00 1B C7 00 17 10 00 00 00 00 68\r\n11/06/15 10:18:17.983 RECV 23 FF A4 16 03 02\r\n11/06/15 10:18:17.561 RECV 23 FF 74 0A 64 72 74 53 61 74 44 72 77 50 6E 4D 31 20 35 31 31\r\n11/06/15 10:18:17.532 RECV 3F E4 60 68 68 6E 00 09 99 A8 01 2D 01 00 3C 54 05 00 00 00 00 5A 00 00\r\n11/06/15 10:18:17.460 RECV 21 E4 41 56 00 00 00 06 00 EA 00 F8 2A F8 2A 11 08 00 00 1B C7 00 17 10 00 00 00 00 68\r\n11/06/15 10:18:17.280 RECV 23 E4 9E 81 00 00 01 01 0F 64 14 00 00 00 00 00 00 00 00 15 00 22 00 BA 0B 00 00\r\n11/06/15 10:18:16.986 RECV 23 FF A4 16 03 02\r\n11/06/15 10:18:16.535 RECV 3F E4 60 68 68 1E 00 09 99 A8 01 92 01 00 3C A4 03 00 00 00 00 6B 00 01\r\n11/06/15 10:18:16.470 RECV 21 E4 41 6D 00 00 00 06 00 EA 00 F8 2A F8 2A 11 08 00 00 1B C7 00 1F 10 00 00 00 00 68\r\n11/06/15 10:18:15.991 RECV 23 FF A4 16 03 02\r\n11/06/15 10:18:15.541 RECV 3F E4 60 68 68 6E 00 09 99 A8 01 09 01 00 3C 3F 01 00 00 00 00 4C 00 01\r\n11/06/15 10:18:15.476 RECV 21 E4 41 2D 00 00 00 06 00 EA 00 F8 2A F8 2A 01 08 00 00 1B C7 00 1D 10 00 00 00 00 68\r\n11/06/15 10:18:15.000 RECV 23 FF A4 16 03 02\r\n11/06/15 10:18:14.845 RECV 23 E4 9E 81 00 00 01 01 0F 64 14 00 00 00 00 00 00 00 00 15 00 22 00 BA 0B 00 00\r\n11/06/15 10:18:14.550 RECV 3F E4 60 68 68 6E 00 09 99 A8 01 D5 01 00 3C 59 0A 00 00 00 00 6C 00 00\r\n11/06/15 10:18:14.482 RECV 21 E4 41 6E 00 00 00 06 00 EA 00 F8 2A F8 2A 11 08 00 00 1B C7 00 1B 10 00 00 00 00 68\r\n11/06/15 10:18:14.006 RECV 23 FF A4 16 03 02\r\n11/06/15 10:18:13.555 RECV 3F E4 60 68 68 6E 00 09 99 A8 01 11 01 00 3C 0D 15 00 00 00 00 38 00 00\r\n11/06/15 10:18:13.488 RECV 21 E4 41 1A 00 00 00 06 00 EA 00 F8 2A F8 2A 01 08 00 00 1B C7 00 0C 10 00 00 00 00 68\r\n11/06/15 10:18:13.014 RECV 23 FF A4 16 03 02\r\n11/06/15 10:18:12.560 RECV 3F E4 60 68 68 6E 00 09 99 A8 01 E5 01 00 3C 62 23 00 00 00 00 66 00 01\r\n11/06/15 10:18:12.494 RECV 21 E4 41 6E 00 00 00 06 00 EA 00 F8 2A F8 2A 11 08 00 00 1B C7 00 14 10 00 00 00 00 68\r\n", "GEA Data"=[["Date", "11/06/2015"], ["Time", "10:20:40.471"], ["Timer", "147.452744"], ["IGBT Temp (Deg C)", "65"], ["Speed", "39"], ["Load Size", "0"], ["Temperature", "105"], ["Water Pressure", "4130"], ["Detergent", "11000"], ["Fabric Softener", "11000"], ["Direction", "CCW"], ["Detergent Valve", "Detergent Off"], ["Fabric Softener Valve", "Fabric Softener Off"], ["Recirculating Pump Valve", "Recirculating Pump Off"], ["Drain Valve", "Drain Off"], ["Hot Valve", "Hot Off"], ["Cold Valve", "Cold Off"], ["Lid Closed", ""], ["Lid Locked", ""], ["Machine Status", "Pause"], ["Serial Number", "15HL2790"], ["Cycle Count", "34"], ["Station Label", "2M1"], ["Board ID", "04125059"], ["Cycle Buffer Index", ""], ["Page Number", ""], ["Delay Start Time", "0"], ["Stain Selected", ""], ["Selected Cycle", "0"], ["eWash", ""], ["Soil Level", ""], ["Temperature", ""], ["Overnight Ready", ""], ["Spin Setting", ""], ["Control Lock Status", ""], ["Stain Remover", ""], ["Steam Assist", ""], ["My Cycle", ""], ["PreWash", ""], ["Debug Log Enabled", ""], ["Rinse", ""], ["Signal Level", ""], ["PreSoak", ""], ["Motor Speed", "105"], ["Latched OOB", "0"], ["Raw OOB", "5220"], ["Plaster Status", "0"], ["Inverter Power (W)", "439"], ["Target Speed (BRPM)", "110"], ["Latched Agitate Motor Temp (Deg C)", "123"], ["Current Motor Temp (Deg C)", "123"], ["Profiler Status", "A899"], ["Current Inverter Action", "Profiler"], ["Error Codes", "Door UnlockDoor Open"], ["Total Cycle Time (Min)", "3002"], ["Total Cycle Count (Current)", "34"], ["Total Error Count", "21"], ["Machine Error History", "0"], ["Washer UI History", "0"], ["Inverter Error History", "342101761"], ["Cycle Storage Limit", "1"], ["Error Storage Limit", "0"], ["Cycle Pages Supported", "0"], ["Error Pages Supported", "129"], ["Inverter Reset Count", "0"]], "Network Variable Location"=0, "Water Heater GEA2 Data"={"GEA2 Label Array"=[], "PID_PARAMETERS"=[], "SUPPORTED_MODES"=[], "Button Status"={"Switch 1"=FALSE, "Switch 2"=FALSE, "Switch 3"=FALSE, "Switch 4"=FALSE, "Switch 5"=FALSE, "Switch 6"=FALSE, "Switch 7"=FALSE, "Switch 8"=FALSE, "Switch 9"=FALSE, "Switch 10"=FALSE, "Switch 11"=FALSE, "Switch 12"=FALSE, "Switch 13"=FALSE, "Switch 14"=FALSE, "Switch 15"=FALSE, "Switch 16"=FALSE}, "Status Query"={"Days Remaining (For Std Electric and Vacation)"=0, "Unit Status"="", "Current Tank Temp in Deg F"=0, "Current Setpoint in Deg F"=0, "Filter Status (% used)"=0, "Fallback Status (Fallback heating mode)"="", "Fallback Temp"=0, "\"Set Mode\" Selection"=""}, "Service Error Codes"={"Reserved"=FALSE, "Reserved 1"=FALSE, "Reserved 2"=FALSE, "Reserved 3"=FALSE, "Reserved 4"=FALSE, "Reserved 5"=FALSE, "Reserved 6"=FALSE, "Reserved 7"=FALSE, "DataFlash Fail Status"=FALSE, "Stuck Key Fail Status"=FALSE, "Dry Tank Fail Status"=FALSE, "Miswire Fail Status"=FALSE, "Reserved 8"=FALSE, "Reserved 9"=FALSE, "Reserved 10"=FALSE, "Reserved 11"=FALSE, "UE Fail Status"=FALSE, "LE Fail Status"=FALSE, "Filter Fail Status"=FALSE, "T3A Fail Status"=FALSE, "T3B Fail Status"=FALSE, "T4 Fail Status"=FALSE, "T5 Fail Status"=FALSE, "T2 Fail Status"=FALSE, "SS Cond A Status"=FALSE, "SS Cond B Status"=FALSE, "SS Cond C Status"=FALSE, "SS Cond D Status"=FALSE, "SS Cond E Status"=FALSE, "SS Cond F Status"=FALSE, "SS Fan Status"=FALSE, "CMP Fail Status"=FALSE}, "HEM_KWH_DATA"=[], "OTHER_FAULT_COUNTS"=[], "GEA2 Raw Message"="", "Hyperterminal Data"={"Source"=0, "Destination"=0, "Command"=0, "Length"=0, "CRC"=0, "UE - state (1/0 on off)"=0, "LE - state (1/0 on off)"=0, "Comp - state (1/0 on off)"=0, "Fan  - state (1/0 on off)"=0, "Setpoint Deg F"=0, "T2(TankSensor)"=0.0, "T3A(EvapIn)"=0.0, "T3B(EvapOut)"=0.0, "T4(CompressorDischarge)"=0.0, "T5(Ambient)"=0.0, "Current"=0.0, "Voltage (Volts)"=0, "EEV Position (0-480)"=0, "Reason for last heating cycle termination"=0, "Reason Data word 1"="", "Reason Data word 2"="", "Reason Data word 3"="", "Reason Data word 4"="", "SW Debug Data"="", "Flow Events (Bit Encoded)"=0, "Heating Control Mode"=0}, "Extra Data"={"Water Capacity (Gallons)"=0, "Max Vacation Duration Days"=0, "Min Vacation Duration Days"=0, "Max Set Point (Deg F)"=0, "Min Set Point (Deg F)"=0, "T5 Resistance"=0, "T4 Resistance"=0, "T3B Resistance"=0, "T2 Resistance"=0, "STD_ELEC_RANGE"="", "SS_FAULT_COUNTS"="", "SERIAL_NUMBER"="", "READ_PERSONALITY"=0, "RQST_OVERRIDE_STATUS"="", "MODEL_SELECT_AD_VALUE"=0, "MODEL NUMBER"="", "IDLB_RESISTANCE"=0, "DSM Override Status"="", "RQST_DATA_FROM_Memory"="", "RQST_DATA_FROM_DATA_FLASH"="", "RQST_CURRENT_PID_SH_TARGET"=0, "Unit System Mode"=""}}} {"Water Heater GEA2 Data"."Hyperterminal Data"."CRC" format="%x"; "Water Heater GEA2 Data"."Hyperterminal Data"."Length" format="%x"; "Water Heater GEA2 Data"."Hyperterminal Data"."Command" format="%x"; "Water Heater GEA2 Data"."Hyperterminal Data"."Destination" format="%x"; "Water Heater GEA2 Data"."Hyperterminal Data"."Source" format="%x"; "Destination Address" format="%x"; "Source Address" format="%x"; "Command" format="%.0x"; "Data to send" format="%x"; "ReceivedData" format="%x"}
  in  "Tab Control 3":enum32{"Main", "Configuration"}(tab)
  in  "Reset Washer":bool
  in  "Personality Number":u8
  in  "Enable Diagnostic Data":T9
  out "Disable 15/17 Washer":bool=TRUE
  in  "Save Data":bool
  in  "Tab Control 4":T10(tab)
  in  "Debug Data":string caption="Debug Log"
  in  "Bus Data":string
  in  "Display Debug":bool=TRUE
  in  "Display Bus Log":bool=TRUE
  out "GEA Data":string[][](array[string])=[["Date", "11/06/2015"], ["Time", "10:20:40.533"], ["Timer", "147.515750"], ["IGBT Temp (Deg C)", "65"], ["Speed", "39"], ["Load Size", "0"], ["Temperature", "105"], ["Water Pressure", "4130"], ["Detergent", "11000"], ["Fabric Softener", "11000"], ["Direction", "CCW"], ["Detergent Valve", "Detergent Off"], ["Fabric Softener Valve", "Fabric Softener Off"], ["Recirculating Pump Valve", "Recirculating Pump Off"], ["Drain Valve", "Drain Off"], ["Hot Valve", "Hot Off"], ["Cold Valve", "Cold Off"], ["Lid Closed", ""], ["Lid Locked", ""], ["Machine Status", "Pause"], ["Serial Number", "15HL2790"], ["Cycle Count", "34"], ["Station Label", "2M1"], ["Board ID", "04125059"], ["Cycle Buffer Index", ""], ["Page Number", ""], ["Delay Start Time", "0"], ["Stain Selected", ""], ["Selected Cycle", "0"], ["eWash", ""], ["Soil Level", ""], ["Temperature", ""], ["Overnight Ready", ""], ["Spin Setting", ""], ["Control Lock Status", ""], ["Stain Remover", ""], ["Steam Assist", ""], ["My Cycle", ""], ["PreWash", ""], ["Debug Log Enabled", ""], ["Rinse", ""], ["Signal Level", ""], ["PreSoak", ""], ["Motor Speed", "21"], ["Latched OOB", "0"], ["Raw OOB", "2525"], ["Plaster Status", "0"], ["Inverter Power (W)", "453"], ["Target Speed (BRPM)", "0"], ["Latched Agitate Motor Temp (Deg C)", "123"], ["Current Motor Temp (Deg C)", "123"], ["Profiler Status", "A899"], ["Current Inverter Action", "Profiler"], ["Error Codes", "Door UnlockDoor Open"], ["Total Cycle Time (Min)", "3002"], ["Total Cycle Count (Current)", "34"], ["Total Error Count", "21"], ["Machine Error History", "0"], ["Washer UI History", "0"], ["Inverter Error History", "342101761"], ["Cycle Storage Limit", "1"], ["Error Storage Limit", "0"], ["Cycle Pages Supported", "0"], ["Error Pages Supported", "129"], ["Inverter Reset Count", "0"]]
  in  "Enable Fault Data":bool
  in  "Clear Table Buffer":bool
  in  "Clear Seq Buffer":bool
  out "Fault Table Buffer":string[][](table)
  out "Fault Sequence Buffer":string
  out "Seq Buffer Status":T11
  out "Fault Set?":bool
  out "Table Buffer Status":T11
  out "Diagnostics Table":string[][](table)
  out "Cycle Buffer Status":T12
  in  "Clear Cycle Buffer Status":bool
  in  "Get Cycle History":bool
  in  "Read ERD":bool
  in  "Write ERD":bool
  in  "GEA Inputs":T13={"Source"=228, "Destination"=35} {"Destination" format="%.0x"; "Source" format="%.0x"}
  in  "Write ERD List":T14[](array[typedef])=[{"ERD Number"=0, "Data Type"=enum."string", "Data"=""}] {"ERD Number" format="%.0x"}
  in  "Read ERD List":T16[](array[typedef])=[{"ERD Number"=0, "Data Type"=enum."string"}] {"ERD Number" format="%.0x"}
  out "Read ERD Data Out":T17[](array[typedef]) {"ERD Number" format="%.0x"}
  in  "Input Data":T18 caption="GEA2 Input Data" {"Command" format="%02x"; "Destination" format="%02x"; "Source" format="%02x"}
  out "GEA2 Output Data":T19 {"CRC" format="%04x"; "Length" format="%02x"; "Command" format="%02x"; "Destination" format="%02x"; "Source" format="%02x"}
  in  "GEA2 Send":bool
  in  "Plot File":T20
  in  "Y-Axis":string(combo)
  out "XY Graph":cluster{"Time Stamp":timestamp[], "DBL":dbl[]}(graph)
  out "Serial Number Front Panel":string="15HL2790" caption="Serial Number"
  out "Lab ID Front Panel":string="15HL2790" caption="Lab ID"
  out "TR Number  Front Panel":string="15HL2790" caption="TR Number"
  out "Board ID.":string
  in  "Personality (0xFF00)":bool
  out "Check Path":bool=TRUE
  out "New File Created":bool
  in  "Run Local 1":bool
  out "UI Events":i32=2
  in  "Cycles/ File":i32=1
  in  "Record Current Status":bool
  in  "File Locations In":T21={"General Setup Paths"={"Calibration File Path"=path "", "DOE Capacity Path"=path "", "Data Folder Path"=path "", "RLT Backup Data Path"=path "", "Tool Base Path"=path "", "General Startup Config Path"=path "", "File Save Previous Run Path"=path "", "File Save Configuration Data Path"=path ""}, "Data File Paths"={"Data File Path"=path "", "Debug File Path"=path "", "Bus Log Path"=path "", "Current"=path "", "Summary"=path ""}, "New Summary Created"=FALSE, "Check Location Interval (Second)"=2}
  out "Number of events discarded":u32
  out "Software Version":T3={"Critical Major SW Version"="0", "Critical Minor SW Version"="0", "Major SW Version"="41", "Minor SW Version"="1", "Parametric Data Ver. Major"="1", "Parametric Data Ver. Minor"="1", "Diagnostics Data Ver. Major"="", "Diagnostics Data Ver. Minor"="", "Current Personality Setting"=""}
  out "UnRead ERDs":i32
  out "File  Version":string="Version"
  out "Status":T23="Not Collecting Data...."
  in  "Tab Control":T24(tab)
  in  "Read Debug States":bool
  out "Control States":string[](array[string])
  in  "Diagnostic Scan Rate":i32=1000
  out "Data Save Loop":i32=197
  out "Data Save Loop":string[](array[string])
  out "HEWH Appliance Data":string[][](array[string])
  out "Cycle Count (0x008E)":i32
  out "Current RMS (Amps) (0xF30D)":dbl
  out "Basket Speed (RPM) (0xF30B)":i32
  out "Machine Status Color":u32(colorbox)
  in  "Use GEA Cycle Counter":bool=TRUE
  in  "#ERDs per message":i32=2
  in  "UI Event SM":string
  out "Last 10 Data Save":string[](array[string])
  out "Last 10 Control":string[](array[string])
  out "Converted Data Out":T19={"Source"=25, "Destination"=228, "Command"=158, "Length"=0, "CRC"=0, "Message"=" 81 00 00 01 01 0F 64 14 00 00 00 00 00 00 00 00 15 00 22 00 BA 0B 00 00"} {"CRC" format="%04x"; "Length" format="%02x"; "Command" format="%02x"; "Destination" format="%02x"; "Source" format="%02x"}
  out "Max Values":T25={"RPM Max"=0, "Cycle Time"=2.4585958321889243, "IGBT Temperature"=0.0, "Load Size"=0.0, "Temperature"=0.0, "Water Pressure"=0.0, "Detergent"=0.0, "Fabric Softener"=0.0, "Inverter Power (W)"=0.0, "Raw OOB"=0.0, "Current Motor Temp (Deg C)"=0.0}
  out "Full Message to Save":string="117 1MnPwrDtaStrd"
  out "Cycle Timer":dbl=148.31282997131348 format="%<%H:%M:%S>t"
  in  "Error In":errorcluster
  out "Washer In":T26={"Appliance Details"={"FileVersionInfo"={"FileVersion"="", "ProductName"="", "InternalName"="", "CompanyName"="", "LegalCopyright"="", "FileDescription"=""}, "Dishwasher Info"={"Open Cup Weight (gm):"=0.0, "Auto Cup Weight (gm):"=0.0, "Detergent-Dish:"="", "Inlet Temperature-Dish:"="", "Cycle Mode-Dish:"="", "Unit Control-Dish:"="", "Manufacturer-Dish:"=""}, "Washer Info"={"Hot Water Temperature (Fahrenheit):"="", "Cold Water Temperature (Fahrenheit):"="", "Capacity (cu.ft):"=0.0, "Initial Cloth Weight:"=0.0, "Cloth Lot:"=0, "Model Family:"="", "Program Name:"="", "Cycle Selection:"="", "Wash Temperature:"="", "Rinse Temperature:"="", "Load Size:"=""}, "File Name Output Array"=[], "Calibration Output Array"=[], "Appliance Common"={"Engineer:"="", "Model Number:"="", "Serial Number:"="", "Comments:"="", "Station ID:"="", "Technician:"="", "TR Number:"="", "Lab ID:"="", "Voltage:"="", "Water Pressure (PSI):"="", "Test Date:"="", "Computer Name:"="", "IP Address:"="", "Ambient RH:"="", "Frequency:"="", "Build:"="", "Filename:"="", "Test Type:"="", "Load Run #:"=0, "Ambient Temperature (F):"="", "File Path:"=path "", "Cycles Per Year"=60}, "Water Heater"={"Heating Mode:"=""}, "Dryer"={"Heat Setting:"="", "Washer Water Temperature (60 ± 5°F):"=60, "Water Hardness (PPM):"=17, "Dryness Setting:"="", "Dryer Type:"="", "Exhaust:"="", "Drying Cycle:"="", "Load Type:"="", "Nominal Load Weight"="", "Dryer Initial IMC Data"={"Measured IMC (lbs)"=7.0, "Actual Initial RMC (%)"=7.0, "RMC (Desired %)"=100.0, "Bone Dry Wt(lbs)"=7.0, "Tolerance(%)"=5.0, "Actual Final RMC (%)"=7.0, "CEF (lbf/kWh)"=0.0, "Minimum Weight (lbf)"=0.0, "Average Weight (lbf)"=0.0, "Maximum Weight (lbf)"=0.0, "Measured IMC In Range?"=FALSE, "Moisture Reduction Factor"=55.5, "Field Use Factor"=1.04, "Empty Dryer Cold Weigth"=0.0, "Energy Standard"=enum."D2-Automatic Dryer", "Weight Cloth (lbs)"=0.0, "Relative Moisture Content (%)"=0.0, "Relative Moisture Content - Avg (%)"=0.0}}}, "Display Data (RLT)"={"Status Color"=0, "Serial Number Display"="", "Cycle Count Display"=0, "Station Label Display"="", "Current Run Start Time Display"=0.0, "Board ID Display"="", "RPM Display"=0, "Current Display"=0.0, "Current Path Display"=path "", "Saving Display"=FALSE, "Unit Type Display"=enum."", "Total Time On Display"=0.0, "UI Button"=FALSE}} {"Display Data (RLT)"."Current Display" format="%.2f"; "Display Data (RLT)"."Cycle Count Display" format="%04d"; "Appliance Details"."Dryer"."Dryer Initial IMC Data"."Maximum Weight (lbf)" format="%03_6g"; "Appliance Details"."Dryer"."Dryer Initial IMC Data"."Average Weight (lbf)" format="%03_6g"; "Appliance Details"."Dryer"."Dryer Initial IMC Data"."Minimum Weight (lbf)" format="%03_6g"; "Appliance Details"."Dryer"."Dryer Initial IMC Data"."CEF (lbf/kWh)" format="%03_6g"; "Appliance Details"."Dryer"."Dryer Initial IMC Data"."Actual Final RMC (%)" format="%03_6g"; "Appliance Details"."Dryer"."Dryer Initial IMC Data"."Tolerance(%)" format="%0#_6g"; "Appliance Details"."Dryer"."Dryer Initial IMC Data"."Bone Dry Wt(lbs)" format="%03_6g"; "Appliance Details"."Dryer"."Dryer Initial IMC Data"."RMC (Desired %)" format="%0#_6g"; "Appliance Details"."Dryer"."Dryer Initial IMC Data"."Actual Initial RMC (%)" format="%03_6g"; "Appliance Details"."Dryer"."Dryer Initial IMC Data"."Measured IMC (lbs)" format="%0#_6g"}
  out "Front Panel Station Label":string="2M1"
  out "Start UI Loop":bool=TRUE
  in  "Status":T34
  out "Handle":dbl
  out "Error":i32
  out "Newfi Timer":dbl=156.3636350631714 format="%<%H:%M:%S>t"
  # "Viper/Hawk"
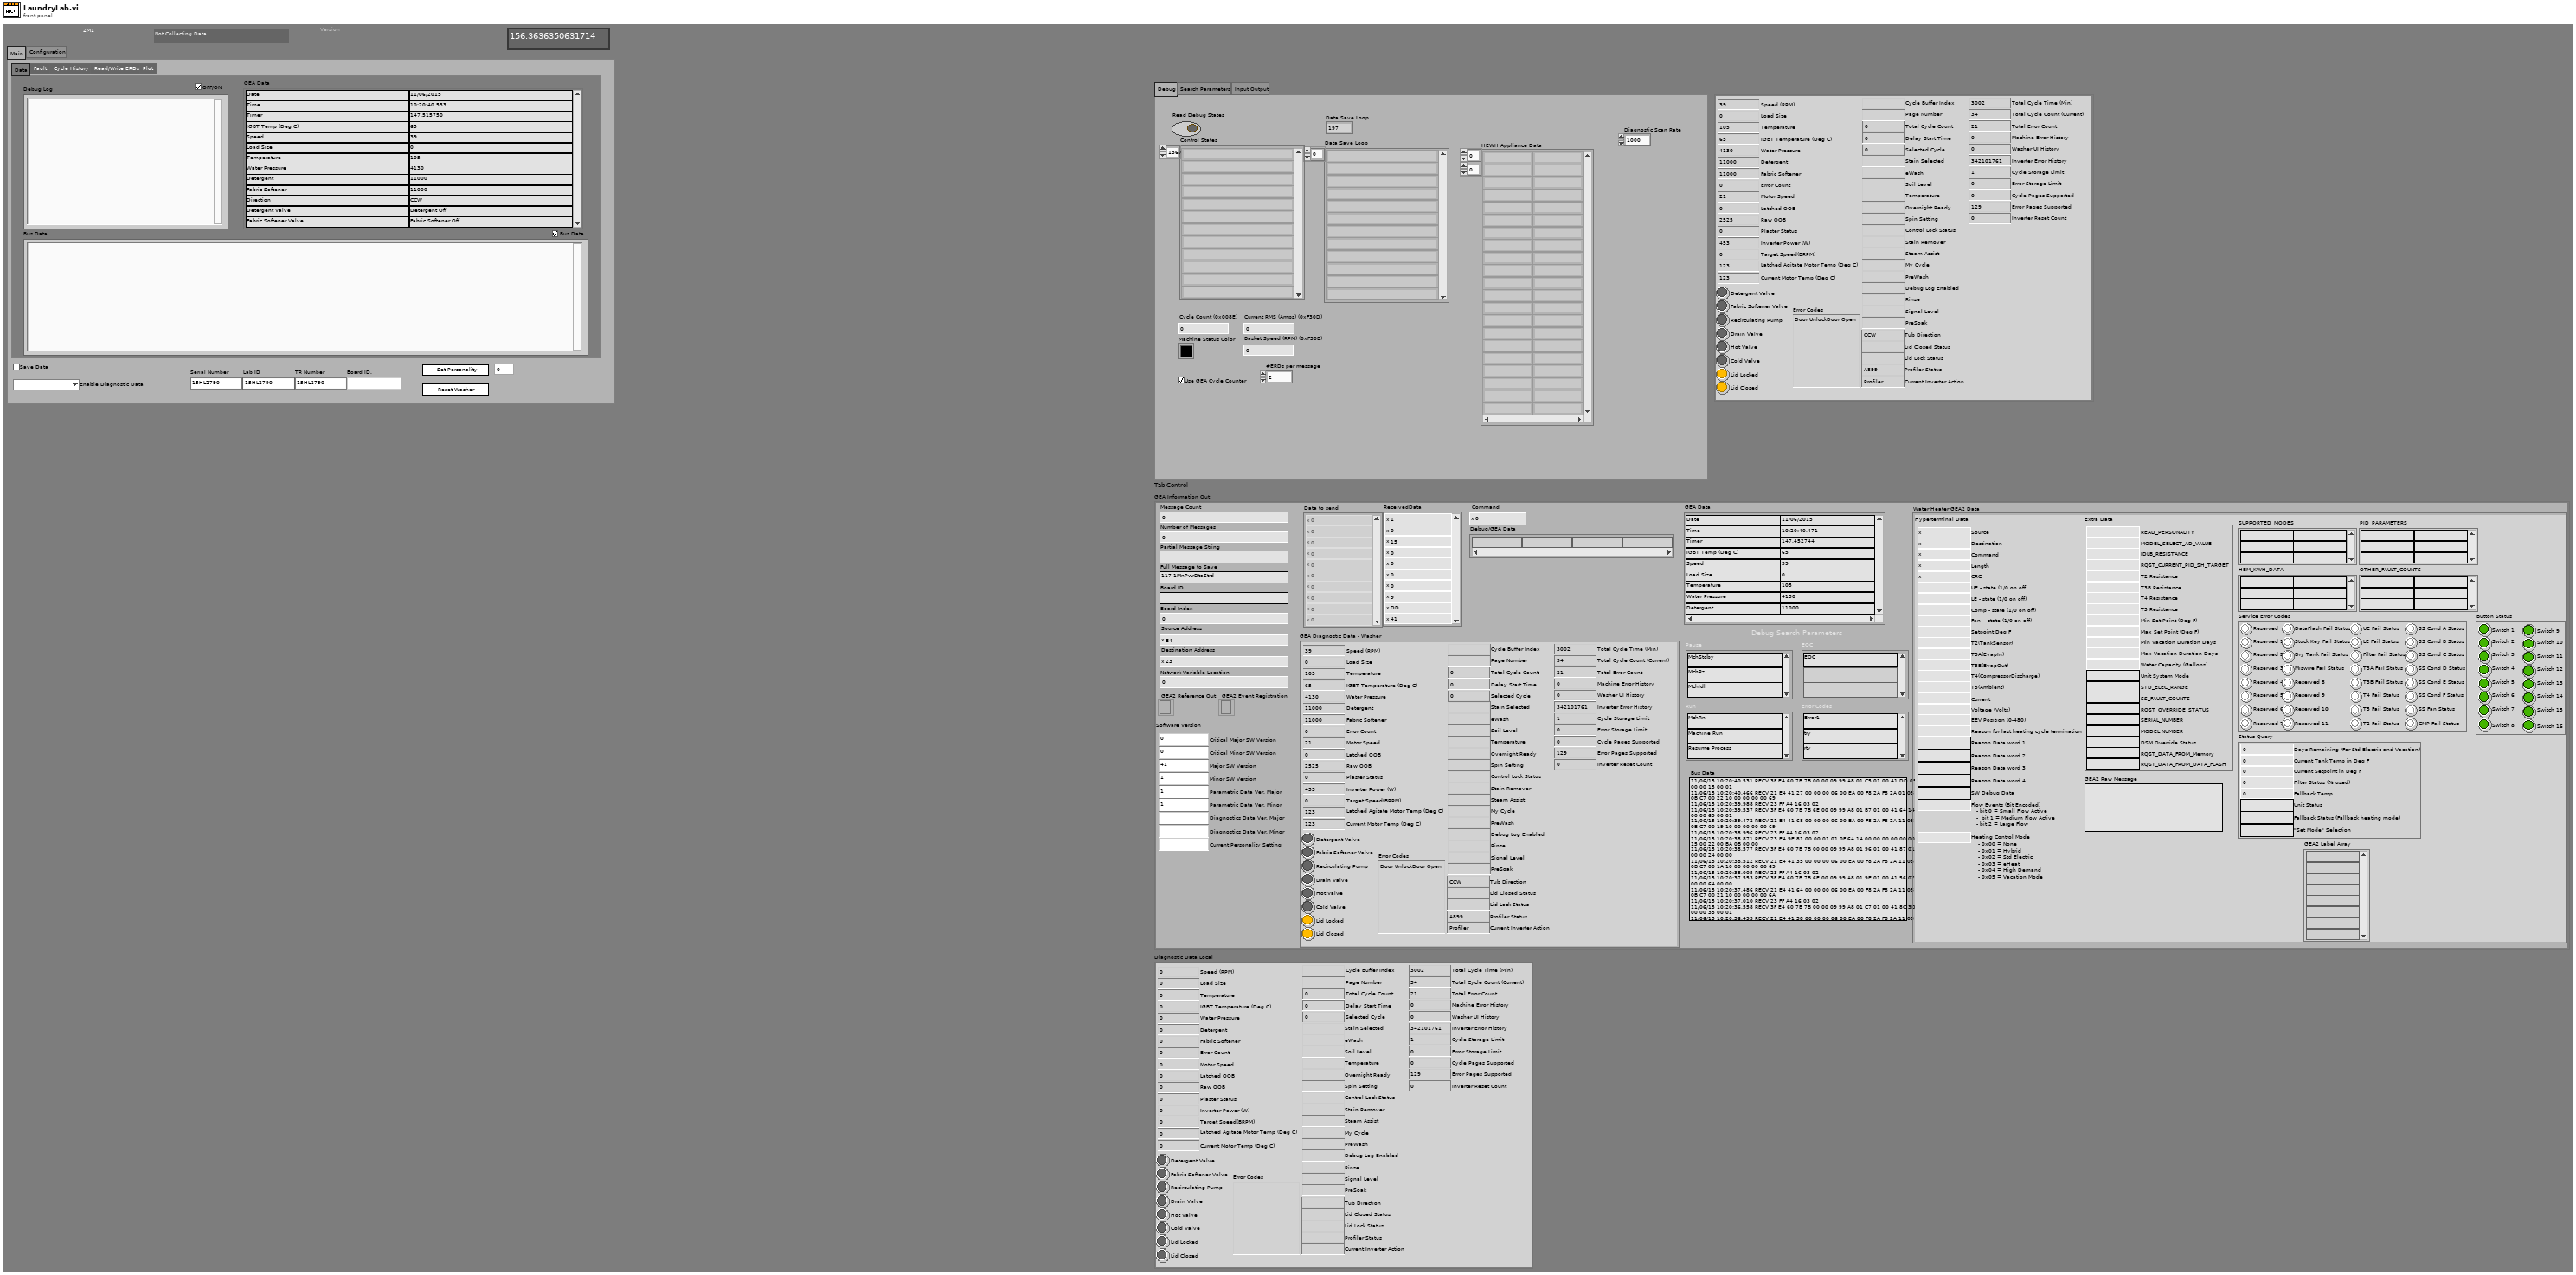
[diagram p1: front panel]
types:
  T1 = typedef "ViperHawk Diagnostic Data.ctl" = cluster{"Speed (RPM)":u32, "Load Size":u32, "Temperature":u32, "Water Pressure":dbl, "Detergent":u32, "Fabric Softener":u32, "Tub Direction":string, "Detergent Valve":bool, "Fabric Softener Valve":bool, "Recirculating Pump":bool, "Drain Valve":bool, "Hot Valve":bool, "Cold Valve":bool, "Lid Closed Status":string, "Lid Lock Status":string, "Error Count":u32, "IGBT Temperature (Deg C)":u32, "Motor Speed":u32, "Latched OOB":u32, "Raw OOB":u32, "Plaster Status":u32, "Inverter Power (W)":u32, "Target Speed(BRPM)":u32, "Latched Agitate Motor Temp (Deg C)":u32, "Current Motor Temp (Deg C)":u32, "Profiler Status":string, "Current Inverter Action":string, "Error Codes":string, "Lid Locked":bool, "Lid Closed":bool, "9E Diagnostic Data":cluster{"Total Cycle Time (Min)":u32, "Total Cycle Count (Current)":u16, "Total Error Count":u16, "Machine Error History":u32, "Washer UI History":u32, "Inverter Error History":u32, "Cycle Storage Limit":u8, "Error Storage Limit":u8, "Cycle Pages Supported":u8, "Error Pages Supported":u8, "Inverter Reset Count":u16}, "9F Diagnostic Data":cluster{"Cycle Buffer Index":string, "Page Number":string, "Total Cycle Count":u32, "Delay Start Time":u32, "Stain Selected":string, "Selected Cycle":u32, "eWash":string, "Soil Level":string, "Temperature":string, "Overnight Ready":string, "Spin Setting":string, "Control Lock Status":string, "Stain Remover":string, "Steam Assist":string, "My Cycle":string, "PreWash":string, "Debug Log Enabled":string, "Rinse":string, "Signal Level":string, "PreSoak":string}}
  T2 = typedef "ViperHawk Data.ctl" = cluster{"GEA Diagnostic Data - Washer":T1, "Software Version":T3, "Debug Search Parameters":T4, "Message Count":i32, "Number of Messages":i32, "Partial Message String":string, "Full Message to Save":string, "Board ID":string, "Board Index":i32, "Source Address":u8, "Destination Address":u8, "Data to send":u8[], "ReceivedData":u8[], "Debug/GEA Data":string[], "Command":u8, "GEA2 Reference Out":refnum<k24>, "GEA2 Event Registration":refnum<event-registration>, "Bus Data":string, "GEA Data":string[][], "Network Variable Location":i32, "Water Heater GEA2 Data":T5}
  T3 = typedef "Save File.lvlib/Save File Software Version.ctl" = cluster{"Critical Major SW Version":string, "Critical Minor SW Version":string, "Major SW Version":string, "Minor SW Version":string, "Parametric Data Ver. Major":string, "Parametric Data Ver. Minor":string, "Diagnostics Data Ver. Major":string, "Diagnostics Data Ver. Minor":string, "Current Personality Setting":string}
  T4 = typedef "ViperHawk Search Control.ctl" = cluster{"Pause":string[], "Run":string[], "EOC":string[], "Error Codes":string[]}
  T5 = typedef "GEA2 Commands WaterHeater GEA2 Data.ctl" = cluster{"GEA2 Label Array":string[], "PID_PARAMETERS":string[][], "SUPPORTED_MODES":string[][], "Button Status":T6, "Status Query":T7, "Service Error Codes":T8, "HEM_KWH_DATA":string[][], "OTHER_FAULT_COUNTS":string[][], "GEA2 Raw Message":string, "Hyperterminal Data":cluster{"Source":u8, "Destination":u8, "Command":u8, "Length":u8, "CRC":u16, "UE - state (1/0 on off)":u8, "LE - state (1/0 on off)":u8, "Comp - state (1/0 on off)":u8, "Fan  - state (1/0 on off)":u8, "Setpoint Deg F":i32, "T2(TankSensor)":dbl, "T3A(EvapIn)":dbl, "T3B(EvapOut)":dbl, "T4(CompressorDischarge)":dbl, "T5(Ambient)":dbl, "Current":dbl, "Voltage (Volts)":u16, "EEV Position (0-480)":u16, "Reason for last heating cycle termination":u16, "Reason Data word 1":string, "Reason Data word 2":string, "Reason Data word 3":string, "Reason Data word 4":string, "SW Debug Data":string, "Flow Events (Bit Encoded)":u16, "Heating Control Mode":u16}, "Extra Data":cluster{"Water Capacity (Gallons)":u32, "Max Vacation Duration Days":u32, "Min Vacation Duration Days":u32, "Max Set Point (Deg F)":u32, "Min Set Point (Deg F)":u32, "T5 Resistance":u32, "T4 Resistance":u32, "T3B Resistance":u32, "T2 Resistance":u32, "STD_ELEC_RANGE":string, "SS_FAULT_COUNTS":string, "SERIAL_NUMBER":string, "READ_PERSONALITY":u8, "RQST_OVERRIDE_STATUS":string, "MODEL_SELECT_AD_VALUE":u32, "MODEL NUMBER":string, "IDLB_RESISTANCE":u32, "DSM Override Status":string, "RQST_DATA_FROM_Memory":string, "RQST_DATA_FROM_DATA_FLASH":string, "RQST_CURRENT_PID_SH_TARGET":u16, "Unit System Mode":string}}
  T6 = typedef "GEA2 Commands Button Status.ctl" = cluster{"Switch 1":bool, "Switch 2":bool, "Switch 3":bool, "Switch 4":bool, "Switch 5":bool, "Switch 6":bool, "Switch 7":bool, "Switch 8":bool, "Switch 9":bool, "Switch 10":bool, "Switch 11":bool, "Switch 12":bool, "Switch 13":bool, "Switch 14":bool, "Switch 15":bool, "Switch 16":bool}
  T7 = typedef "GEA2 Commands Status Query.ctl" = cluster{"Days Remaining (For Std Electric and Vacation)":u8, "Unit Status":string, "Current Tank Temp in Deg F":u8, "Current Setpoint in Deg F":u8, "Filter Status (% used)":u8, "Fallback Status (Fallback heating mode)":string, "Fallback Temp":u8, "\"Set Mode\" Selection":string}
  T8 = typedef "GEA2 Commands Service Error Codes.ctl" = cluster{"Reserved":bool, "Reserved 1":bool, "Reserved 2":bool, "Reserved 3":bool, "Reserved 4":bool, "Reserved 5":bool, "Reserved 6":bool, "Reserved 7":bool, "DataFlash Fail Status":bool, "Stuck Key Fail Status":bool, "Dry Tank Fail Status":bool, "Miswire Fail Status":bool, "Reserved 8":bool, "Reserved 9":bool, "Reserved 10":bool, "Reserved 11":bool, "UE Fail Status":bool, "LE Fail Status":bool, "Filter Fail Status":bool, "T3A Fail Status":bool, "T3B Fail Status":bool, "T4 Fail Status":bool, "T5 Fail Status":bool, "T2 Fail Status":bool, "SS Cond A Status":bool, "SS Cond B Status":bool, "SS Cond C Status":bool, "SS Cond D Status":bool, "SS Cond E Status":bool, "SS Cond F Status":bool, "SS Fan Status":bool, "CMP Fail Status":bool}
  T9 = typedef "HCC Washer Types.ctl" = enum16{"", "Viper Washer", "Hawk Washer", "2015 Washer", "2017 Washer"}
  T10 = enum32{"Data", "Fault", "Cycle History", "Read/Write ERDs", "Plot"}
  T11 = typedef "Fault_Buffer_Status.ctl" = cluster{"Current Index":u16, "Count":u16, "Overwrite Count":u16}
  T12 = typedef "Cycle_Diag_Buffer_Status.ctl" = cluster{"Current Index":u16, "Count":u16, "Overwrite Count":u16}
  T13 = typedef "GEA2_Toolkit.lvlib/Source_Destination.ctl" = cluster{"Source":u8, "Destination":u8}
  T14 = typedef "GEA2_Toolkit.lvlib/ERD Write Data In.ctl" = cluster{"ERD Number":u16, "Data Type":T15, "Data":string}
  T15 = typedef "GEA2_Toolkit.lvlib/Data Type.ctl" = enum16{"string", "boolean", "uint8_t", "uint16_t", "uint32_t", "uint64_t"}
  T16 = typedef "GEA2_Toolkit.lvlib/ERD Read Data In.ctl" = cluster{"ERD Number":u16, "Data Type":T15}
  T17 = typedef "GEA2_Toolkit.lvlib/ERD Read Data Out.ctl" = cluster{"ERD Number":u16, "Data":string}
  T18 = typedef "GEA2_Toolkit.lvlib/Data In.ctl" = cluster{"Source":u8, "Destination":u8, "Command":u8, "Message":string}
  T19 = typedef "GEA2_Toolkit.lvlib/Data Out.ctl" = cluster{"Source":u8, "Destination":u8, "Command":u8, "Length":u8, "CRC":u16, "Message":string}
  T20 = typedef "ViperHawk Plot File.ctl" = enum16{"Summary Data"}
  T21 = typedef "File Setup.lvlib/Save File DOE File Path Control.ctl" = cluster{"General Setup Paths":cluster{"Calibration File Path":path, "DOE Capacity Path":path, "Data Folder Path":path, "RLT Backup Data Path":path, "Tool Base Path":path, "General Startup Config Path":path, "File Save Previous Run Path":path, "File Save Configuration Data Path":path}, "Data File Paths":T22, "New Summary Created":bool, "Check Location Interval (Second)":i32}
  T22 = typedef "File Setup.lvlib/Save File DOE Data Save Filepaths.ctl" = cluster{"Data File Path":path, "Debug File Path":path, "Bus Log Path":path, "Current":path, "Summary":path}
  T23 = typedef "Custom Pallet String.ctl" = string
  T24 = enum32{"Debug", "Search Parameters", "Input Output"}
  T25 = typedef "ViperHawk Summary Stats.ctl" = cluster{"RPM Max":u32, "Cycle Time":dbl, "IGBT Temperature":dbl, "Load Size":dbl, "Temperature":dbl, "Water Pressure":dbl, "Detergent":dbl, "Fabric Softener":dbl, "Inverter Power (W)":dbl, "Raw OOB":dbl, "Current Motor Temp (Deg C)":dbl}
  T26 = typedef "Save File.lvlib/Save File Washer.ctl" = cluster{"Appliance Details":T27, "Display Data (RLT)":T32}
  T27 = typedef "File Setup.lvlib/Save File DISH Dishwasher Details.ctl" = cluster{"FileVersionInfo":T28, "Dishwasher Info":cluster{"Open Cup Weight (gm):":dbl, "Auto Cup Weight (gm):":dbl, "Detergent-Dish:":string, "Inlet Temperature-Dish:":string, "Cycle Mode-Dish:":string, "Unit Control-Dish:":string, "Manufacturer-Dish:":string}, "Washer Info":cluster{"Hot Water Temperature (Fahrenheit):":string, "Cold Water Temperature (Fahrenheit):":string, "Capacity (cu.ft):":dbl, "Initial Cloth Weight:":dbl, "Cloth Lot:":i32, "Model Family:":string, "Program Name:":string, "Cycle Selection:":string, "Wash Temperature:":string, "Rinse Temperature:":string, "Load Size:":string}, "File Name Output Array":string[][], "Calibration Output Array":string[][], "Appliance Common":T29, "Water Heater":cluster{"Heating Mode:":string}, "Dryer":cluster{"Heat Setting:":T23, "Washer Water Temperature (60 ± 5°F):":u16, "Water Hardness (PPM):":u16, "Dryness Setting:":T23, "Dryer Type:":string, "Exhaust:":string, "Drying Cycle:":string, "Load Type:":string, "Nominal Load Weight":string, "Dryer Initial IMC Data":T30}}
  T28 = typedef "FileVersionInformation.ctl" = cluster{"FileVersion":string, "ProductName":string, "InternalName":string, "CompanyName":string, "LegalCopyright":string, "FileDescription":string}
  T29 = typedef "DOE Appliance Common.ctl" = cluster{"Engineer:":string, "Model Number:":string, "Serial Number:":string, "Comments:":string, "Station ID:":string, "Technician:":string, "TR Number:":string, "Lab ID:":string, "Voltage:":string, "Water Pressure (PSI):":string, "Test Date:":string, "Computer Name:":string, "IP Address:":string, "Ambient RH:":string, "Frequency:":string, "Build:":string, "Filename:":string, "Test Type:":string, "Load Run #:":i32, "Ambient Temperature (F):":string, "File Path:":path, "Cycles Per Year":u32}
  T30 = typedef "DPT IMC Data.ctl" = cluster{"Measured IMC (lbs)":dbl, "Actual Initial RMC (%)":dbl, "RMC (Desired %)":dbl, "Bone Dry Wt(lbs)":dbl, "Tolerance(%)":dbl, "Actual Final RMC (%)":dbl, "CEF (lbf/kWh)":dbl, "Minimum Weight (lbf)":dbl, "Average Weight (lbf)":dbl, "Maximum Weight (lbf)":dbl, "Measured IMC In Range?":bool, "Moisture Reduction Factor":dbl, "Field Use Factor":dbl, "Empty Dryer Cold Weigth":dbl, "Energy Standard":T31, "Weight Cloth (lbs)":dbl, "Relative Moisture Content (%)":dbl, "Relative Moisture Content - Avg (%)":dbl}
  T31 = typedef "DOE Dryer Standard.ctl" = enum16{"D2-Automatic Dryer", "D2-Timer Dryer", "D1-Automatic Dryer", "D1-Timer Dryer", "Other"}
  T32 = typedef "Save File Appliance Display.ctl" = cluster{"Status Color":u32, "Serial Number Display":string, "Cycle Count Display":i32, "Station Label Display":string, "Current Run Start Time Display":dbl, "Board ID Display":string, "RPM Display":u32, "Current Display":dbl, "Current Path Display":path, "Saving Display":bool, "Unit Type Display":T33, "Total Time On Display":dbl, "UI Button":bool}
  T33 = typedef "Save File.lvlib/Save File Unit Type.ctl" = enum32{"", "Viper", "Hawk", "2015"}
  T34 = typedef "ViperHawk Status.ctl" = enum16{"Start Data Collection", "Stop Data Collection"}
  T35 = cluster{"ERD Number":u16, "Data Type":enum16{"string", "boolean", "uint8_t", "uint16_t", "uint32_t", "uint64_t", "int8_t", "int16_t", "int32_t", "int64_t"}}[]
  T36 = cluster{"Reset Timer?":bool, "Update Daq Loop":bool, "TR Number":string, "Notes":string, "Serial Number":string, "Lab ID":string, "Status":T34, "Cycle Count":i32, "Plot File":T20}
  T37 = cluster{"Time Stamp":timestamp[], "Data with 0's and 1's":dbl[]}
  T38 = typedef "lveventtype.ctl" = enum32{"Null", "Timeout", "Annotation Menu Selection", "Annotation Menu Selection?", "App Instance Close", "App Instance Close?", "Autoscale Range Change", "Bookmark Info Change", "Cell Edit", "Cell Edit?", "Cursor Grab", "Cursor Grab?", "Cursor Menu Selection", "Cursor Menu Selection?", "Cursor Move", "Cursor Release", "Data Change", "Direction Change", "Display State Change", "Drag Ended", "Drag Enter", "Drag Leave", "Drag Over", "Drag Source Update", "Drag Starting", "Drag Starting?", "Drop", "Exec State Change", "Key Down", "Key Down?", "Key Repeat", "Key Repeat?", "Key Up", "Listbox Double Click", "Menu Activation?", "Menu Selection (App)", "Menu Selection? (App)", "Menu Selection (User)", "Mouse Down", "Mouse Down?", "Mouse Enter", "Mouse Leave", "Mouse Move", "Mouse Up", "Mouse Wheel", "NI Security User Change (App)", "Pane Size", "Panel Close", "Panel Close?", "Panel Resize", "Plot Attribute Change", "Scale Range Change", "Shortcut Menu Activation?", "Shortcut Menu Selection (App)", "Shortcut Menu Selection? (App)", "Shortcut Menu Selection (User)", "Tree Double Click", "Tree Drag", "Tree Drag?", "Tree Drop", "Tree Drop?", "Tree Item Close", "Tree Item Close?", "Tree Item Open", "Tree Item Open?", "User Event", "Value Change"}
  T39 = enum32{"Invalid", "Standard", "Closed", "Hidden", "Minimized", "Maximized"}
  T40 = enum32{"invalid app kind", "Development System", "Run Time System", "Student Edition", "Embedded LabVIEW", "Evaluation", "Custom"}
  T41 = cluster{"Current VI Reference":refnum<vi>, "Close Panel on Exit?":bool}
  T42 = typedef "File Setup.lvlib/Save File DOE LabView Program.ctl" = enum16{"No Name Found", "DOE Stand", "Dishwasher Kitchen", "Portable Stand", "HEWH", "Dryer", "Dryer WILT", "HCC", "PRAT", "HEWH RLT", "Refrigeration"}
  T43 = typedef "ViperHawk Timers.ctl" = cluster{"Cycle Timer":dbl, "Timer":dbl}
  T44 = cluster{"Core":cluster{"Current VI Reference":refnum<vi>, "Close Panel on Exit?":bool}, "GEA Information Out":T2, "Main Washer Display Out":T26, "File Paths Out":T21, "Timers":T43, "Cycle Stats":T25, "Cycles/ File":i32}
  T45 = typedef "sizeaction.ctl" = enum32{"Minimized", "Maximized", "Resized"}
  T46 = typedef "ViperHawk logData.ctl" = cluster{"IGBT Temp (Deg C)":u8, "Speed":u32, "Load Size":u32, "Temperature":u8, "Water Pressure":u32, "Detergent":u32, "Fabric Softener":u32, "Direction":string, "Det":bool, "FS":bool, "Recirc":bool, "Drain":bool, "Hot":bool, "Cold":bool, "LidClosed":bool, "LidLocked":bool, "Motor Speed":u16, "Latched Out Of Balance":u16, "Raw Out Of Balance":u16, "Plaster Status":u8, "Inverter Power (Watts)":u16, "Profiler Status":string, "Profiler CRC":u16, "Current Inverter Action":string, "Target Speed (BRPM)":u16, "Latched Agitate Motor Temp (Deg C)":u8, "Current Motor Temp (Deg C)":u8, "Error Codes 1":string}
  T47 = enum8{"Enabled", "Disabled", "Disabled and Grayed Out"}
  T48 = cluster{"Total Cycle Time (Min)":u32, "Total Cycle Count (Current)":u16, "Total Error Count":u16, "Machine Error History":u32, "Washer UI History":u32, "Inverter Error History":u32, "Cycle Storage Limit":u8, "Error Storage Limit":u8, "Cycle Pages Supported":u8, "Error Pages Supported":u8, "Inverter Reset Count":u16}
  T49 = cluster{"Cycle Buffer Index":string, "Page Number":string, "Total Cycle Count":u32, "Delay Start Time":u32, "Stain Selected":string, "Selected Cycle":u32, "eWash":string, "Soil Level":string, "Temperature":string, "Overnight Ready":string, "Spin Setting":string, "Control Lock Status":string, "Stain Remover":string, "Steam Assist":string, "My Cycle":string, "PreWash":string, "Debug Log Enabled":string, "Rinse":string, "Signal Level":string, "PreSoak":string}
  T50 = typedef "Save File Headers.ctl" = cluster{"Summary Header":string[], "Current Header":string[], "Debug Log Header":string[], "Data Header":string[]}
  T51 = cluster{"GEA Information Out":T2, "Headers":T50, "Timers":T43, "File Locations Out":T21, "Cycle Stats":T25, "Diagnostic":T1}
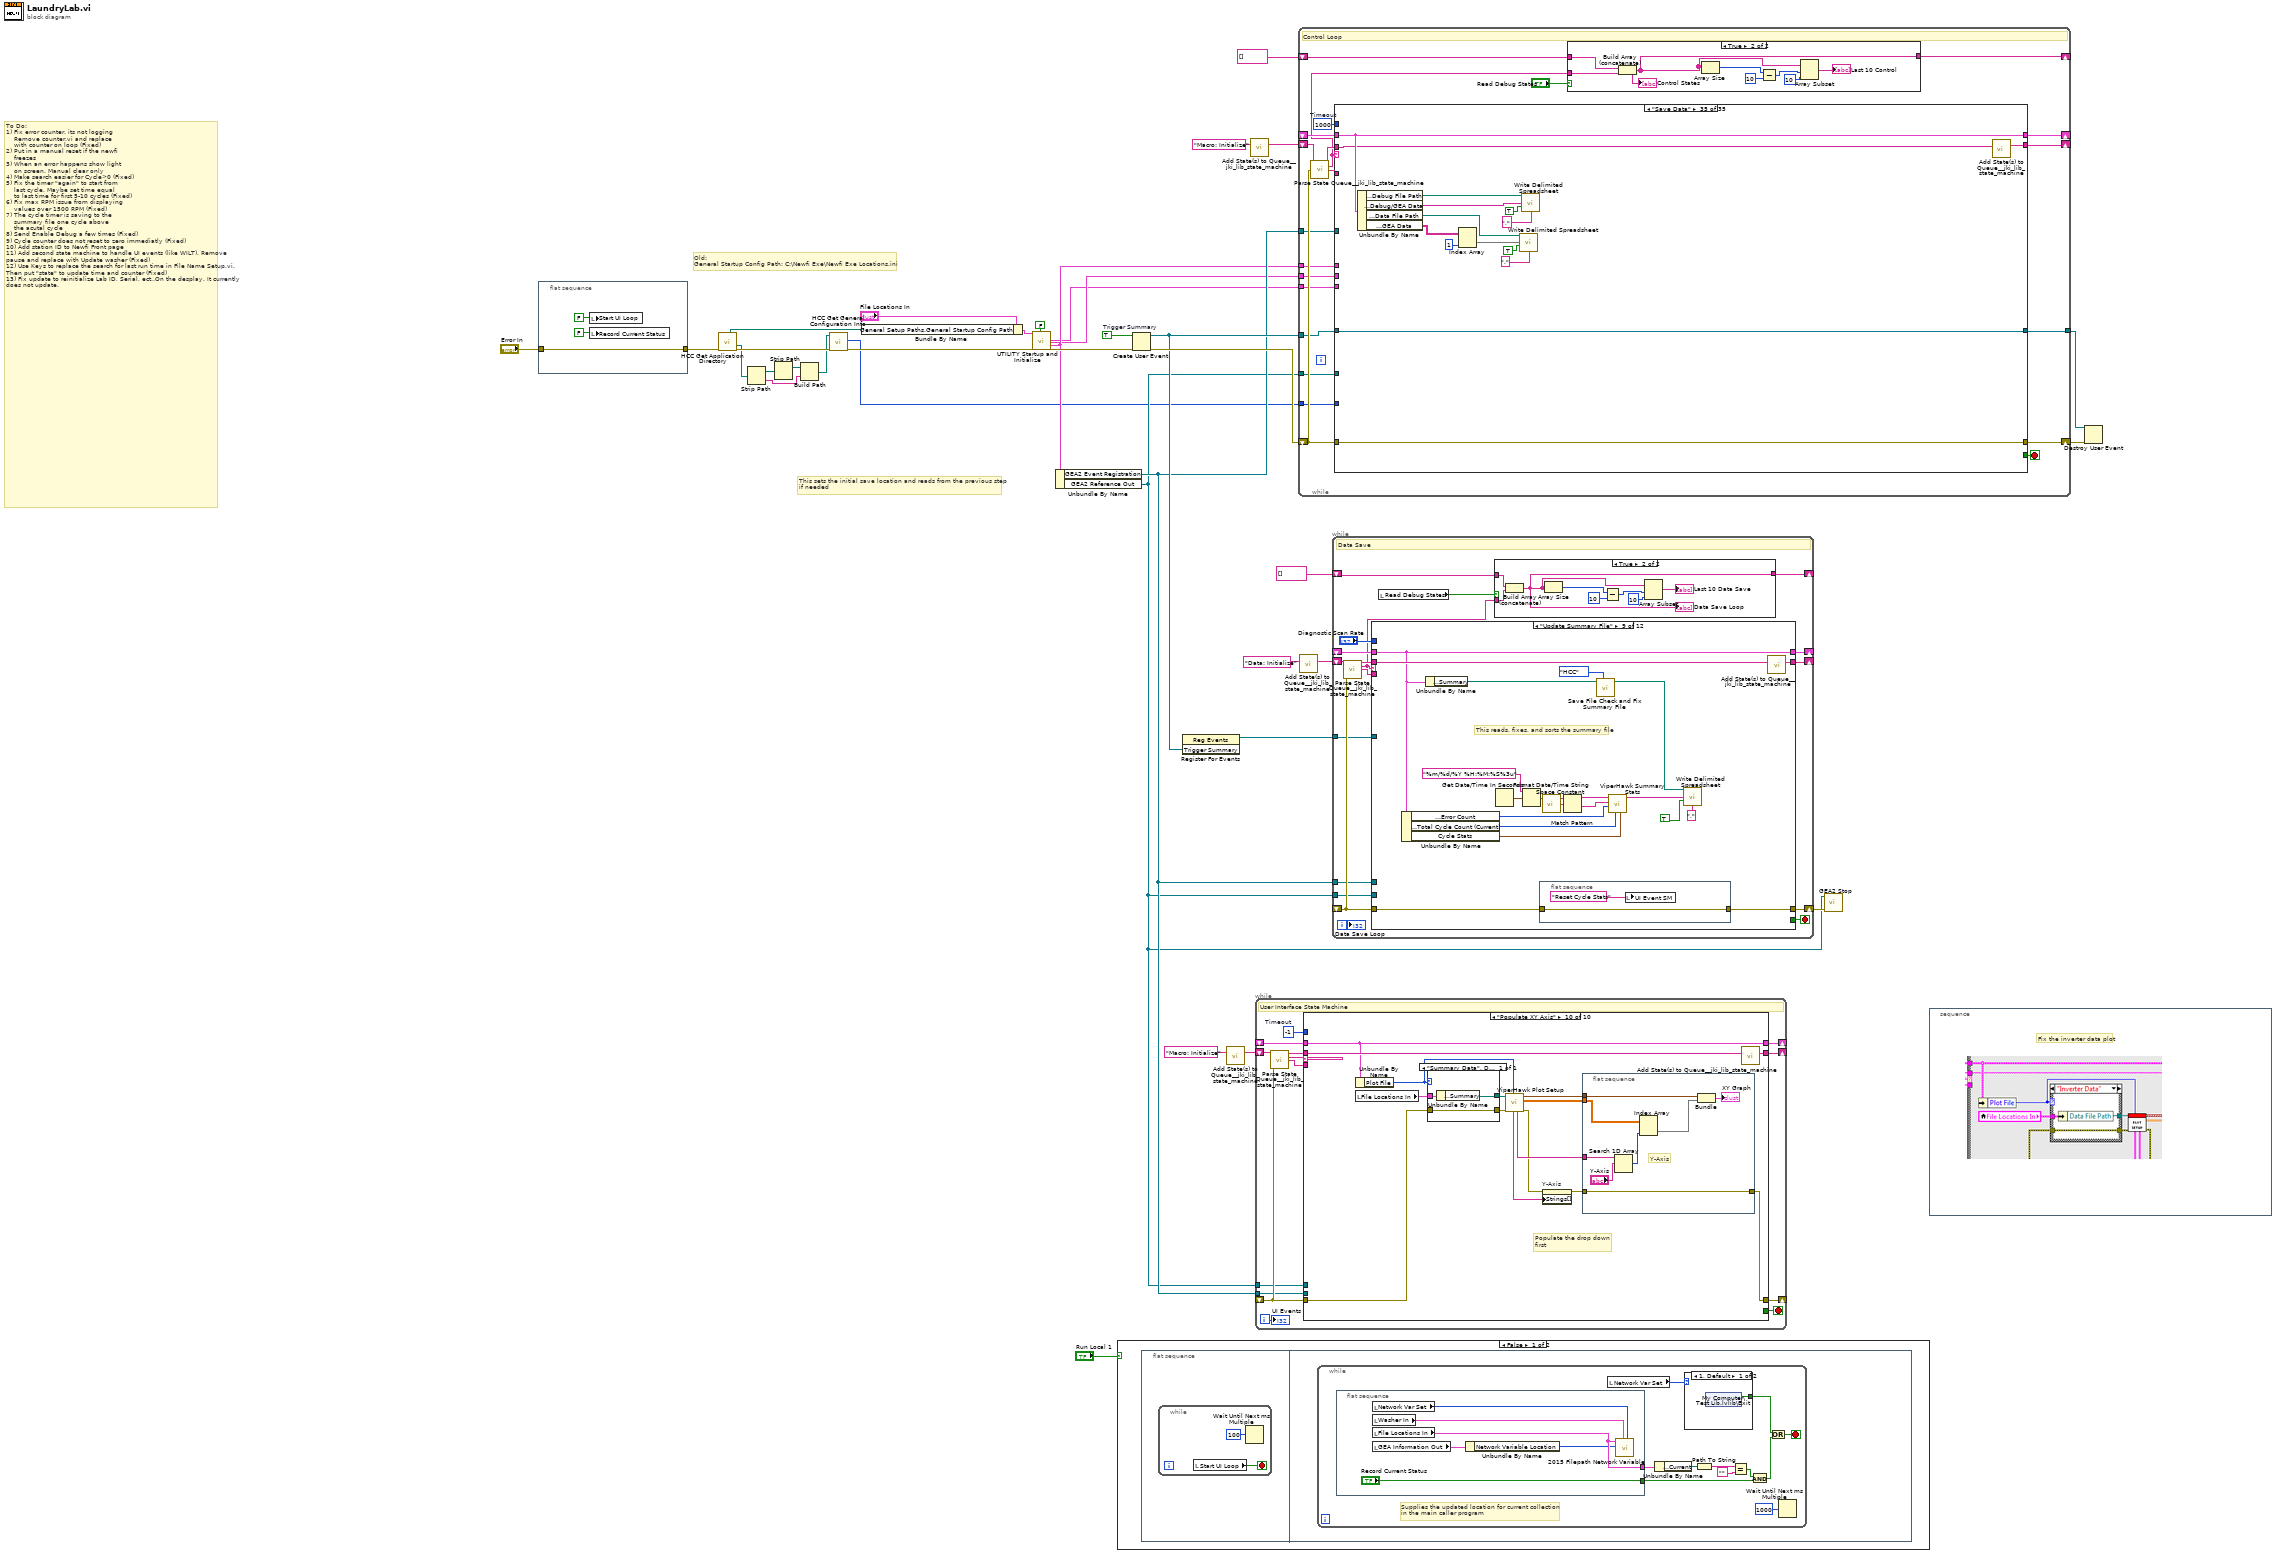
[diagram p0: block diagram]
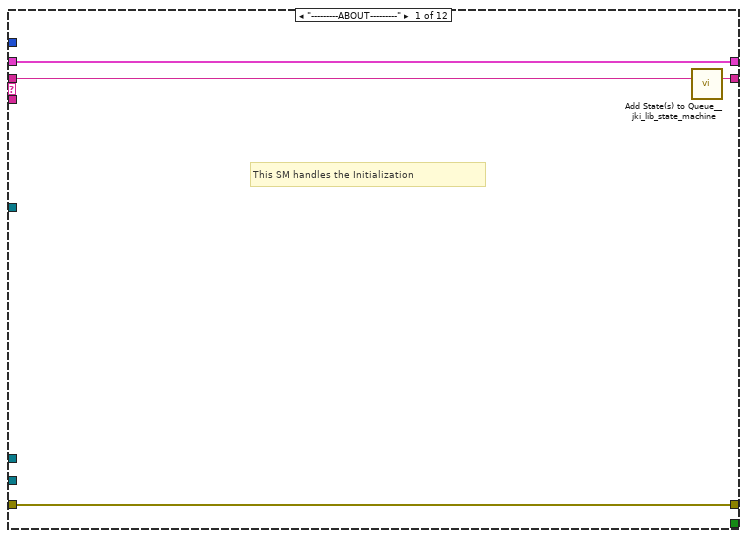
[diagram p3: hidden frame]
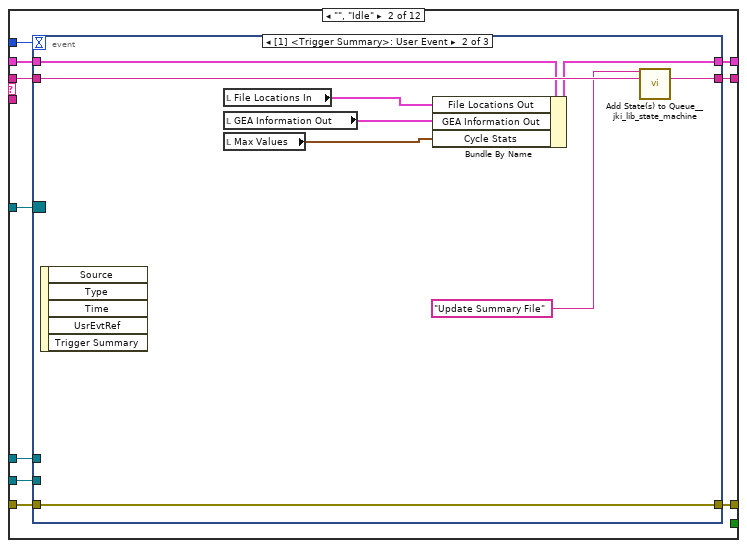
[diagram p4: hidden frame]
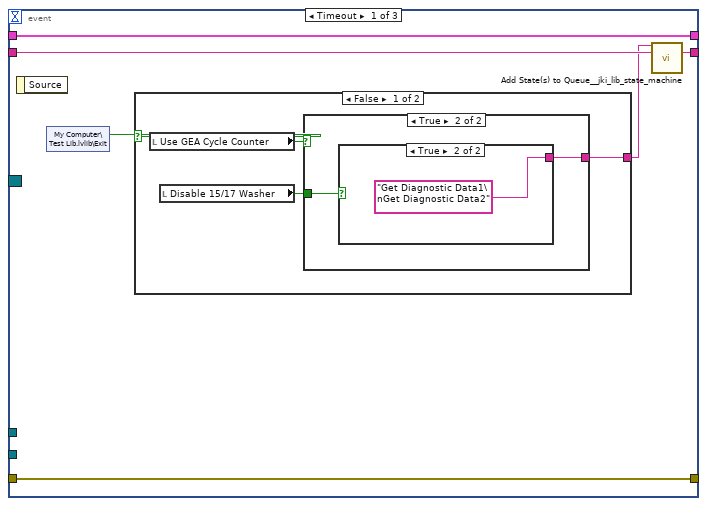
[diagram p5: hidden frame]
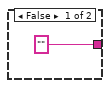
[diagram p6: hidden frame]
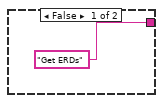
[diagram p7: hidden frame]
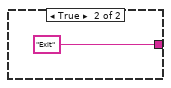
[diagram p8: hidden frame]
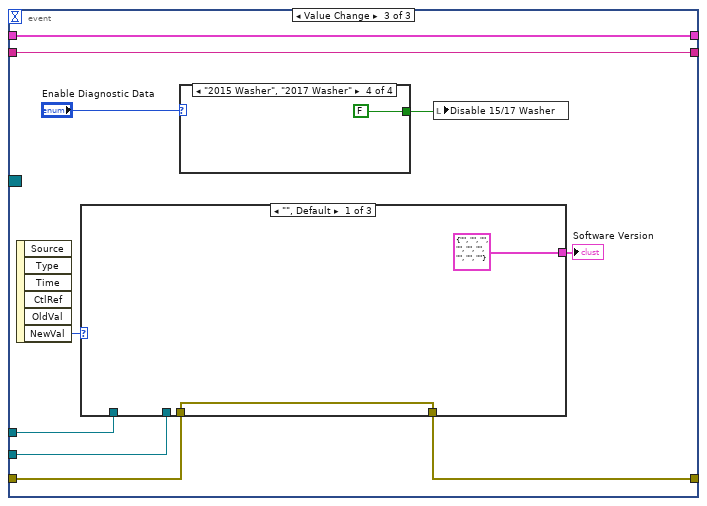
[diagram p9: hidden frame]
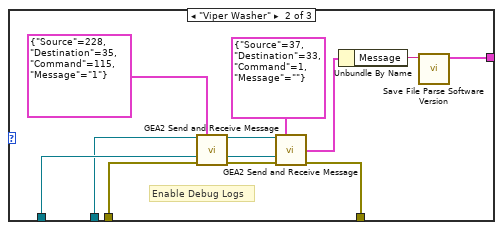
[diagram p10: hidden frame]
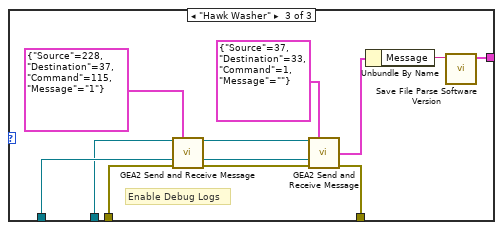
[diagram p11: hidden frame]
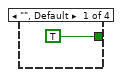
[diagram p12: hidden frame]
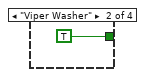
[diagram p13: hidden frame]
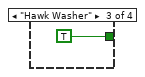
[diagram p14: hidden frame]
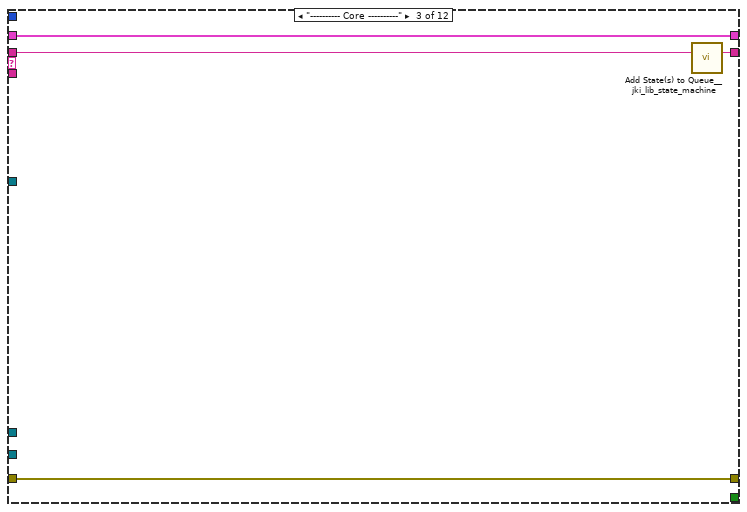
[diagram p15: hidden frame]
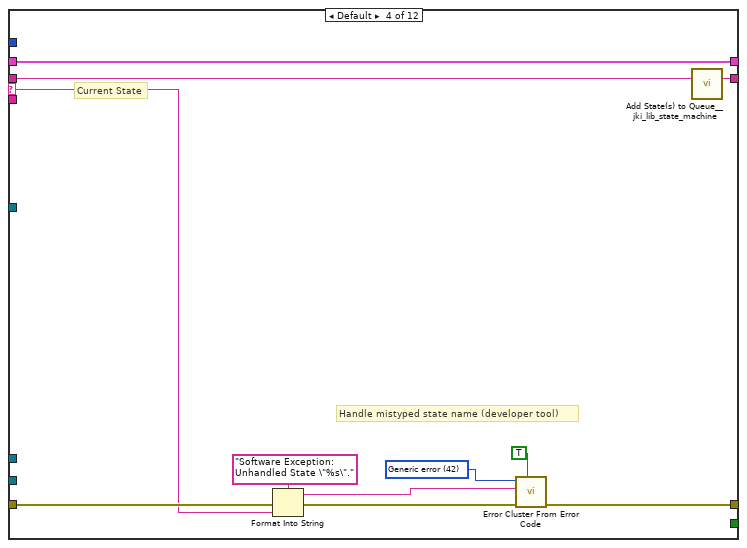
[diagram p16: hidden frame]
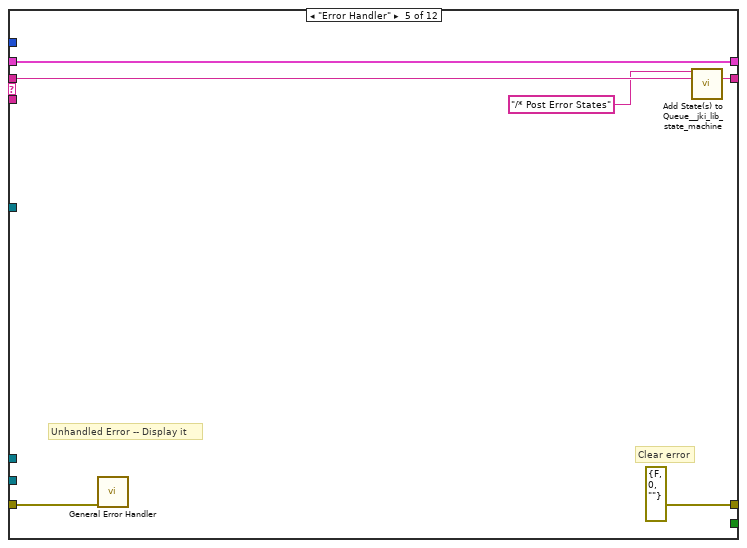
[diagram p17: hidden frame]
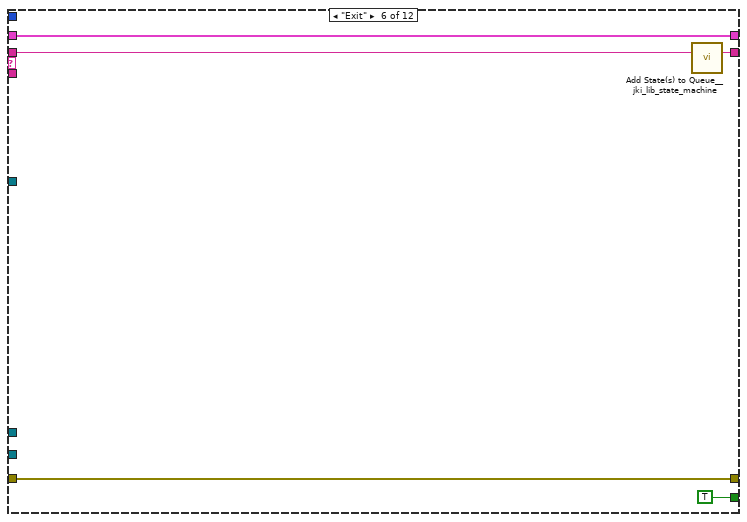
[diagram p18: hidden frame]
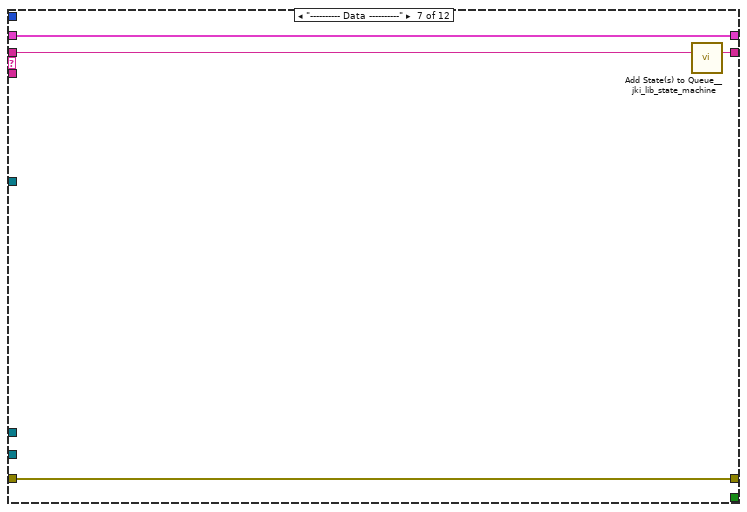
[diagram p19: hidden frame]
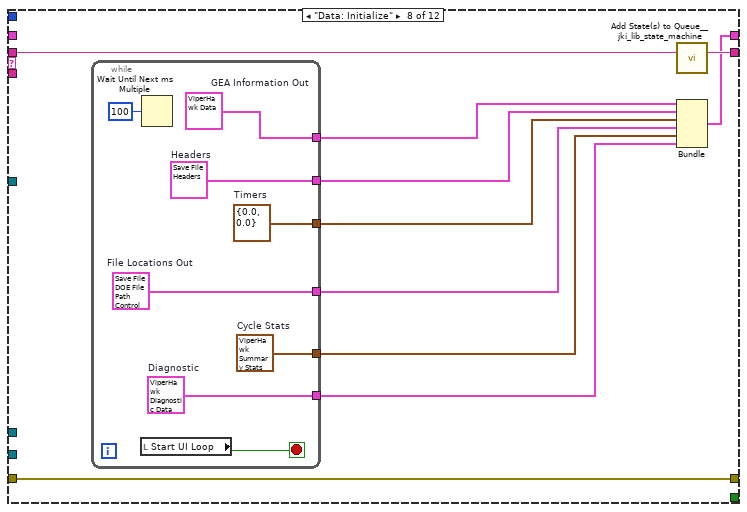
[diagram p20: hidden frame]
diagram:
  w23 = TRUE  # Trigger Summary
  # "Old:\nGeneral Startup Config Path: C:\\Newfi Exe\\Newfi Exe Locations.ini"
  # "This sets the initial save location and reads from the previous step \nif needed"
  # "To Do:\n1) Fix error counter. its not logging\n    Remove counter.vi and replace \n    with counter on loop (Fixed)\n2) Put in a manual reset if the newfi\n    freezes\n3) When an error happens show light\n    on screen. Manual clear only\n4) Make search easier for Cycle>0 (Fixed)\n5) Fix the timer \"again\" to start from \n    last cycle. Maybe set time equal\n    to last time for first 5-10 cycles (Fixed)\n6) Fix max RPM issue from displaying \n    values over 1500 RPM (Fixed)\n7) The cycle timer is saving to the\n    summary file one cycle above \n    the acutal cycle\n8) Send Enable Debug a few times (Fixed)\n9) Cycle counter does not reset to zero immediatly (Fixed)\n10) Add station ID to Newfi Front page\n11) Add second state machine to handle UI events (like WILT). Remove pause and replace with Update washer (Fixed)\n12) Use Keys to replace the search for last run time in File Name Setup.vi. Then put \"state\" to update time and counter (Fixed)\n13) Fix update to reinitialize Lab ID, Serial, ect..On the desplay. It currently does not update."
  n1 = flat-sequence {
    tunnel: [w38] -> w12
    tunnel: "Error In" -> [w38]
    frame #0 {
      n2 = local write "Start UI Loop"(FALSE ("Start UI Loop")) -> ()
      n3 = local write "Record Current Status"(FALSE ("GEA2")) -> ()
    }
  }
  n4 = call "HCC Get Application Directory.vi"("Error In"=w12) -> ("Error Out"=w8:errorcluster, "General Configuration out"=w6:path, "Configuration Path Laundry Lab APP"=w9:path)  [unwired: 5 in, 3 out]
  n5 = Strip Path(path=w6) -> (stripped path=w5:path, name=w3:string)
  n6 = Strip Path(path=w5) -> (stripped path=w4:path)  [unwired: 1 out]
  n7 = Build Path(base path=w4, name or relative path=w3) -> (appended path=w2:path)
  n8 = call "HCC Get General Configuration Info.vi"("Error In"=w8, "General Configuration"=w2) -> ("Error Out"=w7:errorcluster, "Network Var Set"=w1:u8)  [unwired: 7 in, 1 out]
  n9 = Bundle By Name(cluster="File Locations In", "General Setup Paths.General Startup Config Path"=w9) -> (w10:T21)
  n10 = call "UTILITY Startup and Initialize.vi"("File Locations In"=w10, "Error In"=w7, "Read Default Path"=FALSE ("Debug")) -> ("File Paths Out"=w14:T21, "Main Washer Display Out"=w15:T26, "GEA Information Out"=w16:T2, "Error Out"=w17:errorcluster)  [unwired: 21 in]
  n11 = Unbundle By Name(w16) -> ("GEA2 Event Registration"=w18:refnum<event-registration>, "GEA2 Reference Out"=w13:refnum<k24>)
  n12 = case shown="False" "Run Local 1" {
    frame False {
      n13 = flat-sequence {
        frame #0 {
          n14 = while {
            stop <- w41 stop-if-true
            n15 = local read "Start UI Loop"() -> (w41:bool)
            n16 = Wait Until Next ms Multiple(millisecond multiple=u32 100) -> ()  [unwired: 1 out]
          }
        }
        frame #1 {
          n17 = while {
            stop <- w51 stop-if-true
            # "Supplies the updated location for current collection\nin the main caller program"
            n18 = flat-sequence {
              tunnel: ["Record Current Status"] -> w46
              tunnel: [w59] -> w45
              frame #0 {
                n19 = local read "Network Var Set"() -> (w55:u8)
                n20 = local read "Washer In"() -> (w56:T26)
                n21 = local read "File Locations In"() -> (w59:T21)
                n22 = local read "GEA Information Out"() -> (w58:T2)
                n23 = Unbundle By Name(w58) -> ("Network Variable Location"=w57:i32)
                n24 = call "2015 Filepath Network Variable.vi"("Network Var Set"=w55, "Washer In"=w56, "Network Variable Location"=w57, "File Locations In"=w59) -> ()  [unwired: 6 in, 2 out]
              }
            }
            n25 = local read "Network Var Set"() -> (w42:u8)
            n26 = Unbundle By Name(w45) -> ("Data File Paths.Current"=w44:path)
            n27 = case shown="1, Default" w42 {
              tunnel: [w53 w54] -> w52
              frame 1, Default {
                n28 = shared-variable "My Computer\\Test Lib.lvlib\\Exit"() -> (w53:bool)  [unwired: 1 in, 1 out]
              }
              frame 2 {
                n29 = shared-variable "My Computer\\Test Lib.lvlib\\Exit-2"() -> (w54:bool)  [unwired: 1 in, 1 out]
              }
            }
            n30 = Path To String(path=w44) -> (string=w43:string)
            n31 = Equal?(x=w43, y="") -> (x = y?=w47:bool)
            n32 = And(x=w47, y=w46) -> (x .and. y?=w48:bool)
            n33 = Or(x=w52, y=w48) -> (x .or. y?=w51:bool)
            n34 = Wait Until Next ms Multiple(millisecond multiple=u32 1000) -> ()  [unwired: 1 out]
          }
        }
      }
    }
    frame True {
    }
  }
  n35 = Create User Event(user event datatype=w23, error in=w17) -> (user event=w21:refnum<user-event>, error out=w22:errorcluster)
  n36 = register-events(w21) -> (reference out=w20:refnum<event-registration>)  [unwired: 2 in, 1 out]
  n37 = call <vilib>:"Add State(s) to Queue__jki_lib_state_machine.vi"("State(s) in (\"\")"="Macro: Initialize") -> ("States Out"=w35:string)  [unwired: 14 in]
  n38 = call <vilib>:"Add State(s) to Queue__jki_lib_state_machine.vi"("State(s) in (\"\")"="Macro: Initialize" ("State(s) in (\"\")")) -> ("States Out"=w36:string)  [unwired: 14 in]
  n39 = while "UI State Machine" {
    shift-right: [w67] -> _
    shift-left: _ -> [w66]
    shift-right: [w70] -> _
    shift-left: _ -> [w64]
    shift-right: [w69] -> _
    shift-left: w35 -> [w71]
    tunnel: w13 -> [w62]
    tunnel: w18 -> [w61]
    i -> [w63]
    stop <- w68 stop-if-true
    w65 = -1  # Timeout
    # "User Interface State Machine"
    n40 = call <vilib>:"Parse State Queue__jki_lib_state_machine.vi"("State Queue"=w71, "Error In (no error)"=w64) -> ("Remaining States"=w73:string, "Current State"=w74:string, "Arguments"=w72:string)  [unwired: 11 in]
    n41 = case shown="\"Populate XY Axis\"" w74 {
      selector: w74 -> [_ _ _ w217 _ _ _ _ _ _]
      tunnel: w73 -> [w78 w88 w216 w221 w233 w238 w242 w255 w271 w286]
      tunnel: w72 -> [_ _ _ _ _ _ _ _ _ _]
      tunnel: w66 -> [w75 w86 w213 w219 w230 w236 w239 _ w268 w280]
      tunnel: [w76 w85 w214 w223 errorcluster {"status"=FALSE, "code"=0, "source"=""} ("error out") w235 w240 w252 w269 w275] -> w70
      tunnel: w64 -> [w76 w84 w214 w222 w229 w235 w240 w252 w269 w276]
      tunnel: [w77 w87 w215 w220 w232 w237 w241 w254 w270 w285] -> w69
      tunnel: [_ _ _ _ _ TRUE _ _ _ _] -> w68
      tunnel: [w75 w83 w213 w219 w230 w236 w239 w253 w268 w280] -> w67
      tunnel: w65 -> [_ w82 _ _ _ _ _ _ _ _]
      tunnel: w62 -> [_ w81 _ _ _ _ _ _ _ _]
      tunnel: w61 -> [_ w80 _ _ _ _ _ _ _ _]
      frame "---------ABOUT---------" {
        # "This state machine handles most of the UI events. I did this due\nto slow performance and allows me to easily change units \nthroughout the test. (Physically move them from one location\nto another without affecting the program operation)\n\nGoal:\n1) Create new file name without creating unwanted file names"
        n42 = call <vilib>:"Add State(s) to Queue__jki_lib_state_machine.vi"("State(s) in (\"\")"=w78) -> ("States Out"=w77:string)  [unwired: 14 in]
      }
      frame "", "Idle" {
        n43 = event shown="[0] Timeout" {
          selector: _ -> [_ _ _ _ _ _ _ _ _ _ _]
          dyn-events: _ -> [_ _ _ _ _ _ _ _ _ _ _]
          timeout: w82 -> [_ _ _ _ _ _ _ _ _ _ _]
          tunnel: w88 -> [w95 w106 w120 w128 w139 w148 w171 w181 w191 w204 w210]
          tunnel: [w94 w106 w120 w128 w139 w148 w171 w181 w191 w204 w211] -> w87
          tunnel: w86 -> [w92 w107 w121 w129 w140 w149 w172 w182 w192 w205 w208]
          tunnel: [w93 w101 w118 w133 w143 w153 w166 w175 w184 w199 w212] -> w85
          tunnel: w84 -> [w93 w102 w119 w134 w144 w154 w167 w176 w185 w200 w212]
          tunnel: [w92 w107 w121 w129 w140 w149 w172 w182 w192 w205 w206] -> w83
          tunnel: w81 -> [_ w103 w116 w132 w142 w152 w165 w174 w186 w198 _]
          tunnel: w80 -> [_ w100 _ _ _ w151 _ _ _ w197 _]
          tunnel: "GEA Inputs" -> [_ _ _ w131 w141 w150 w164 w173 w183 w196 _]
          event Timeout {
            n44 = event-data() -> ()  [unwired: 1 in, 1 out]
            n45 = local read "Network Var Set"() -> (w89:u8)
            n46 = case shown="1, Default" w89 {
              tunnel: [w96 w97] -> w91
              frame 1, Default {
                n47 = shared-variable "My Computer\\Test Lib.lvlib\\Exit"() -> (w96:bool)  [unwired: 1 in, 1 out]
              }
              frame 2 {
                n48 = shared-variable "My Computer\\Test Lib.lvlib\\Exit-2"() -> (w97:bool)  [unwired: 1 in, 1 out]
              }
            }
            n49 = case shown="True" w91 {
              tunnel: ["" "Exit"] -> w90
              frame False {
              }
              frame True {
              }
            }
            n50 = call <vilib>:"Add State(s) to Queue__jki_lib_state_machine.vi"("State(s) in Front (\"\")"=w90, "State(s) in (\"\")"=w95) -> ("States Out"=w94:string)  [unwired: 13 in]
          }
          event "GEA2 Send": Value Change {
            n51 = event-data() -> ()  [unwired: 1 in, 6 out]
            n52 = call "GEA2 Send and Receive Message.vi"("GEA2 Reference In"=w103, "Input Data"="Input Data", "GEA2 Event Registration"=w100, "Error In"=w102) -> ("Converted Data Out"=→"GEA2 Output Data":T19, "Error Out"=w101:errorcluster)  [unwired: 6 in, 4 out]
          }
          event "Personality (0xFF00)": Value Change {
            w115 = T13 {"Source"=240, "Destination"=35}  # GEA Inputs
            n53 = event-data() -> ()  [unwired: 1 in, 6 out]
            n54 = local read "Enable Diagnostic Data"() -> (w108:T9)
            n55 = case shown="\"2015 Washer\"" w108 {
              tunnel: [T14[] [{"ERD Number"=65280, "Data Type"=enum."uint8_t", "Data"=""}] ("Write ERD List") T14[] [{"ERD Number"=61440, "Data Type"=enum."uint8_t", "Data"=""}] ("Write ERD List")] -> w112
              frame "2017 Washer", Default {
              }
              frame "2015 Washer" {
              }
            }
            n56 = for {
              N: 1 -> [_]
              tunnel: w112 -> [w127] mode=indexing
              tunnel: [w126] -> w111 mode=indexing
              tunnel: "Personality Number" -> [w125]
              n57 = Number To Decimal String(number=w125) -> (decimal integer string=w124:string)  [unwired: 1 in]
              n58 = Bundle By Name(cluster=w127, "Data"=w124) -> (w126:T14)
            }
            n59 = call "GEA2 Write ERD.vi"("GEA2 Reference In"=w116, "Retry Count"=5, "Read Timeout (ms)"=u32 200, "GEA Inputs"=w115, "Write ERD List"=w111, "Error In"=w119, "Verify ERD Response?"=FALSE) -> ("Error Out"=w118:errorcluster)  [unwired: 6 in, 2 out]
          }
          event "Write ERD": Value Change {
            n60 = event-data() -> ()  [unwired: 1 in, 6 out]
            n61 = call "GEA2 Write ERD.vi"("GEA2 Reference In"=w132, "Retry Count"=5, "Read Timeout (ms)"=u32 200, "GEA Inputs"=w131, "Write ERD List"="Write ERD List", "Error In"=w134, "Verify ERD Response?"=FALSE) -> ("Error Out"=w133:errorcluster)  [unwired: 6 in, 2 out]
          }
          event "Reset Washer": Value Change {
            n62 = event-data() -> ()  [unwired: 1 in, 6 out]
            n63 = call "GEA2 Write ERD.vi"("GEA2 Reference In"=w142, "Retry Count"=5, "Read Timeout (ms)"=u32 200, "GEA Inputs"=w141, "Write ERD List"=T14[] [{"ERD Number"=61462, "Data Type"=enum."string", "Data"="0"}], "Error In"=w144, "Verify ERD Response?"=FALSE) -> ("Error Out"=w143:errorcluster)  [unwired: 6 in, 2 out]
          }
          event "Get Cycle History": Value Change {
            # "Cycle History ERDs"
            n64 = event-data() -> ()  [unwired: 1 in, 6 out]
            n65 = call "GEA2 Read ERD Multiple Messages.vi"("GEA2 Reference In"=w152, "Read Timeout (ms)"=u32 500, "GEA Inputs"=w150, "Read ERD List"=T35 [{"ERD Number"=135, "Data Type"=enum."string"}, {"ERD Number"=57344, "Data Type"=enum."string"}, {"ERD Number"=57345, "Data Type"=enum."string"}, {"ERD Number"=57346, "Data Type"=enum."string"}, {"ERD Number"=57347, "Data Type"=enum."string"}, {"ERD Number"=57348, "Data Type"=enum."string"}, {"ERD Number"=57349, "Data Type"=enum."string"}, {"ERD Number"=57350, "Data Type"=enum."string"}, {"ERD Number"=57351, "Data Type"=enum."string"}, {"ERD Number"=57352, "Data Type"=enum."string"}, {"ERD Number"=57353, "Data Type"=enum."string"}], "GEA2 Event Registration"=w151, "Error In"=w154, "#ERDs per message"=4, "Verify ERD Response?"=TRUE) -> ("ERD Data Out"=w158:T17[], "Error Out"=w156:errorcluster)  [unwired: 3 in, 3 out]
            n66 = call "Cycle_Diag_Table_Read.vi"("ERD Data In"=w158, "error in (no error)"=w156) -> ("Cycle Buffer Status"=→"Cycle Buffer Status":T12, "Diag Cycle String Out"=→"Diagnostics Table":string[][], "error out"=w153:errorcluster)  [unwired: 10 in, 1 out]
          }
          event "Clear Cycle Buffer Status": Value Change {
            n67 = event-data() -> ()  [unwired: 1 in, 6 out]
            n68 = call "GEA2 Write ERD.vi"("GEA2 Reference In"=w165, "Retry Count"=5, "Read Timeout (ms)"=u32 200, "GEA Inputs"=w164, "Write ERD List"=T14[] [{"ERD Number"=136, "Data Type"=enum."string", "Data"="FF"}], "Error In"=w167, "Verify ERD Response?"=FALSE) -> ("Error Out"=w166:errorcluster)  [unwired: 6 in, 2 out]
          }
          event "Clear Seq Buffer": Value Change {
            n69 = event-data() -> ()  [unwired: 1 in, 6 out]
            n70 = call "GEA2 Write ERD.vi"("GEA2 Reference In"=w174, "Retry Count"=5, "Read Timeout (ms)"=u32 200, "GEA Inputs"=w173, "Write ERD List"=T14[] [{"ERD Number"=133, "Data Type"=enum."string", "Data"="FF"}], "Error In"=w176, "Verify ERD Response?"=FALSE) -> ("Error Out"=w175:errorcluster)  [unwired: 6 in, 2 out]
          }
          event "Clear Table Buffer": Value Change {
            n71 = event-data() -> ()  [unwired: 1 in, 6 out]
            n72 = call "GEA2 Write ERD.vi"("GEA2 Reference In"=w186, "Retry Count"=5, "Read Timeout (ms)"=u32 200, "GEA Inputs"=w183, "Write ERD List"=T14[] [{"ERD Number"=130, "Data Type"=enum."string", "Data"="FF"}], "Error In"=w185, "Verify ERD Response?"=FALSE) -> ("Error Out"=w184:errorcluster)  [unwired: 6 in, 2 out]
          }
          event "Read ERD": Value Change {
            n73 = event-data() -> ()  [unwired: 1 in, 6 out]
            n74 = call "GEA2 Read ERD Multiple Messages.vi"("GEA2 Reference In"=w198, "Retry Count"=5, "Read Timeout (ms)"=u32 200, "GEA Inputs"=w196, "Read ERD List"="Read ERD List", "GEA2 Event Registration"=w197, "Error In"=w200, "#ERDs per message"=5, "Verify ERD Response?"=FALSE) -> ("ERD Data Out"=→"Read ERD Data Out":T17[], "Error Out"=w199:errorcluster)  [unwired: 2 in, 3 out]
          }
          event "Y-Axis": Value Change {
            n75 = event-data() -> ()  [unwired: 1 in, 6 out]
            n76 = Bundle By Name(cluster=w208, "Plot File"="Plot File") -> (w206:T36)
            n77 = call <vilib>:"Add State(s) to Queue__jki_lib_state_machine.vi"("State(s) in Front (\"\")"="Populate XY Axis", "State(s) in (\"\")"=w210) -> ("States Out"=w211:string)  [unwired: 13 in]
          }
        }
      }
      frame "---------- Core ----------" {
        n78 = call <vilib>:"Add State(s) to Queue__jki_lib_state_machine.vi"("State(s) in (\"\")"=w216) -> ("States Out"=w215:string)  [unwired: 14 in]
      }
      frame Default {
        w226 = 42 items=["No error", "Argument error", "Memory is full", "Out of zone", "End of file", "File already open", "Generic file I/O error", "File not found", "File permission error", "Disk is full", "Duplicate path", "Too many files open", "System feature not enabled", "Resource file not found", "Cannot add resource", "Resource not found", "Image not found", "Image memory error", "Pen does not exist", "Config type invalid", "Config token not found", "Config parse error", "Config memory error", "Bad external code format", "Bad external code offset", "External code not present", "Null window", "Destroy window error", "Null menu", "Print aborted", "Bad print record", "Print driver error", "Windows error during printing", "Memory error during printing", "Print dialog error", "Generic print error", "Invalid device refnum", "Device not found", "Device parameter error", "Device unit error", "Cannot open device", "Device call aborted", "Generic error", "Cancelled by user", "Object ID too low", "Object ID too high", "Object not in heap", "Unknown heap", "Unknown object (invalid DefProc)", "Unknown object (DefProc not in table)", "Message out of range", "Invalid (null) method", "Unknown message", "Manager call not supported", "Bad address", "Network operation in progress", "Network operation timed out", "Connection is busy", "Network attribute not supported", "Network error", "Address in use", "System out of memory", "Connection aborted", "Connection refused", "Not connected", "Already connected", "Connection closed", "Initialization error (interapplication manager)", "Bad occurrence", "Wait on unbound occurrence handler", "Occurrence queue overflow", "Datalog type conflict", "Unused", "Unrecognized type (interapplication manager)", "Memory corrupt", "Failed to make temporary DLL", "Old CIN version", "Drag socket not found", "Failed to load drop-object", "Failed to register OLE object", "Failed to release OLE object", "Format specifier type mismatch", "Unknown format specifier", "Too few format specifiers", "Too many format specifiers", "Scan failed", "Newer CIN version", "Error converting to variant", "Runtime menu error", "Password tampered", "Variant attribute not found", "Incompatible variant data type", "Event data is not available", "Event Store is not present", "Occurrence is not found", "Event Queue is not created", "Event info is not available", "Refnum passed is NULL", "Error retrieving Class GUID", "Error retrieving CoClass GUID", "Error retrieving TypeLib GUID.", "Bad built application magic bytes.", "Specific driver is different from the specific driver associated with the Logical Name.", "There is no session opened to the class driver.", "Max Error", "MAX - Error with config objects", "MAX - Error loading configuration", "MAX - Group not supported"]
        # "Current State"
        # "Handle mistyped state name (developer tool)"
        n79 = Format Into String(format string="Software Exception: Unhandled State \"%s\"." ("message"), error in=w222, w217) -> (resulting string=w225:string, error out=w224:errorcluster)  [unwired: 1 in]
        n80 = call <vilib>:"Error Cluster From Error Code.vi"("show call chain? (False)"=TRUE, "error in (no error)"=w224, "error message (\"\")"=w225, "error code (0)"=w226) -> ("error out"=w223:errorcluster)  [unwired: 5 in]
        n81 = call <vilib>:"Add State(s) to Queue__jki_lib_state_machine.vi"("State(s) in (\"\")"=w221) -> ("States Out"=w220:string)  [unwired: 14 in]
      }
      frame "Error Handler" {
        # "Unhandled Error -- Display it"
        # "Clear error"
        n82 = call <vilib>:"General Error Handler.vi"("error in (no error)"=w229) -> ()  [unwired: 10 in, 5 out]
        n83 = call <vilib>:"Add State(s) to Queue__jki_lib_state_machine.vi"("State(s) in Front (\"\")"="/* Post Error States", "State(s) in (\"\")"=w233) -> ("States Out"=w232:string)  [unwired: 13 in]
      }
      frame "Exit" {
        n84 = call <vilib>:"Add State(s) to Queue__jki_lib_state_machine.vi"("State(s) in (\"\")"=w238) -> ("States Out"=w237:string)  [unwired: 14 in]
      }
      frame "---------- Data ----------" {
        n85 = call <vilib>:"Add State(s) to Queue__jki_lib_state_machine.vi"("State(s) in (\"\")"=w242) -> ("States Out"=w241:string)  [unwired: 14 in]
      }
      frame "Data: Initialize" {
        n86 = flat-sequence {
          tunnel: [FALSE ("Update Daq Loop")] -> w251
          tunnel: ["" ("TR Number")] -> w250
          tunnel: ["" ("Notes")] -> w249
          tunnel: ["" ("Serial Number")] -> w248
          tunnel: ["" ("Lab ID")] -> w247
          tunnel: ["Status"] -> w246
          tunnel: [0 ("Cycle Count")] -> w245
          tunnel: [FALSE ("Reset Timer?")] -> w244
          tunnel: [ViperHawk_Plot_File."Summary Data" ("Plot File")] -> w243
          frame #0 {
            # "Start Loop After Init of Main\nLoop"
            n87 = while {
              stop <- w256 stop-if-true
              n88 = local read "Start UI Loop"() -> (w256:bool)
              n89 = Wait Until Next ms Multiple(millisecond multiple=u32 100) -> ()  [unwired: 1 out]
            }
          }
          frame #1 {
          }
        }
        n90 = Bundle("Reset Timer?"=w244, "Update Daq Loop"=w251, "TR Number"=w250, "Notes"=w249, "Serial Number"=w248, "Lab ID"=w247, "Status"=w246, "Cycle Count"=w245, "Plot File"=w243) -> (w253:T36)  [unwired: 1 in]
        n91 = call <vilib>:"Add State(s) to Queue__jki_lib_state_machine.vi"("State(s) in (\"\")"=w255) -> ("States Out"=w254:string)  [unwired: 14 in]
      }
      frame "Macro: Initialize" {
        # "Initialization Macro\n(This is called once, when the VI starts)"
        n92 = call <vilib>:"Add State(s) to Queue__jki_lib_state_machine.vi"("State(s) in Front (\"\")"="Data: Initialize", "State(s) in (\"\")"=w271) -> ("States Out"=w270:string)  [unwired: 13 in]
      }
      frame "Populate XY Axis" {
        # "Populate the drop down \nfirst"
        n93 = Unbundle By Name(w280) -> ("Plot File"=w273:T20)
        n94 = local read "File Locations In"() -> (w272:T21)
        n95 = case shown="\"Summary Data\", Default" w273 {
          tunnel: [w296] -> w284
          tunnel: w272 -> [w297]
          tunnel: w276 -> [w295]
          tunnel: [w295] -> w279
          frame "Summary Data", Default {
            n96 = Unbundle By Name(w297) -> ("Data File Paths.Summary"=w296:path)
          }
        }
        n97 = call "ViperHawk Plot Setup.vi"("Plot File"=w273, "error in (no error)"=w279, "Log Inverter File"=w284) -> ("error out"=w278:errorcluster, "Data with 0's and 1's"=w282:dbl[][], "Time Stamp"=w281:timestamp[], "Y-Axis Search"=w283:string[], "Y-Axis Drop Down Data"=w274:string[])  [unwired: 4 in]
        n98 = property on="Y-Axis" class="CmbBox"(error in=w278, "Strings[]"=w274) -> (error out=w277:errorcluster)  [unwired: 1 in, 1 out]
        n99 = flat-sequence {
          tunnel: w283 -> [w292]
          tunnel: w282 -> [w288]
          tunnel: w281 -> [w291]
          tunnel: w277 -> [w289]
          tunnel: [w289] -> w275
          frame #0 {
            # "Y-Axis"
            n100 = Search 1D Array(1D array=w292, element="Y-Axis") -> (index of element=w294:i32)  [unwired: 1 in]
            n101 = Index Array(array=w288, index (col)=w294) -> (element=w287:dbl[])  [unwired: 1 in]
            n102 = Bundle("Time Stamp"=w291, "Data with 0's and 1's"=w287) -> (→"XY Graph":T37)  [unwired: 1 in]
          }
        }
        n103 = call <vilib>:"Add State(s) to Queue__jki_lib_state_machine.vi"("State(s) in (\"\")"=w286) -> ("States Out"=w285:string)  [unwired: 14 in]
      }
    }
    "UI Events" <- w63
  }
  n104 = while "Producer Loop" {
    shift-right: [w313] -> _
    shift-left: _ -> [w312]
    shift-right: [w316] -> w25
    shift-left: w22 -> [w310]
    shift-right: [w315] -> _
    shift-left: w36 -> [w317]
    shift-right: [w307] -> _
    shift-left: string[] [] -> [w306]
    tunnel: w18 -> [w305]
    tunnel: w14 -> [w304]
    tunnel: [w303] -> w24
    tunnel: w21 -> [w302]
    tunnel: w16 -> [w301]
    tunnel: w15 -> [w300]
    tunnel: w13 -> [w299]
    tunnel: w1 -> [w298]
    stop <- w314 stop-if-true
    w311 = 1000  # Timeout
    # "Control Loop"
    n105 = call <vilib>:"Parse State Queue__jki_lib_state_machine.vi"("State Queue"=w317, "Error In (no error)"=w310) -> ("Remaining States"=w319:string, "Current State"=w308:string, "Arguments"=w318:string)  [unwired: 11 in]
    n106 = case shown="\"Save Data\"" w308 {
      selector: w308 -> [_ _ w427 _ _ _ _ _ _ _ _ _ _ _ _ _ _ _ _ _ _ _ _ _ _ _ _ _ _ _ _ _ _ _ _]
      tunnel: w319 -> [w332 w425 w431 w450 w457 w463 w468 w485 w492 w500 w517 w525 w530 w541 w550 w596 w609 w623 w628 w634 w639 w650 w654 w680 w732 w758 w767 w771 w793 w812 w825 w839 w874 w937 w970]
      tunnel: w318 -> [_ _ _ _ _ _ _ _ _ _ _ _ _ _ w544 w591 _ _ _ _ _ _ _ _ _ _ _ _ _ _ _ _ _ _ _]
      tunnel: w312 -> [w334 w422 w429 w440 w454 w461 w465 _ w486 w496 w516 w523 w527 w533 w545 w594 w607 w620 w625 w631 w643 w647 w658 w674 w735 w756 w764 w773 w787 w809 w821 w835 w875 w932 w971]
      tunnel: [w336 w423 w433 w448 errorcluster {"status"=FALSE, "code"=0, "source"=""} ("error out") w460 w466 w479 w490 w494 w513 w521 w528 w539 w546 w592 w603 w621 w626 w632 w644 w648 w656 w667 w736 w759 w765 w778 w791 w811 w823 w828 w885 w928 w972] -> w316
      tunnel: w310 -> [w337 w423 w432 w448 w453 w460 w466 w480 w490 w495 w514 w520 w528 w539 w547 w593 w604 w621 w626 w632 w644 w648 w657 w671 w736 w759 w765 w778 w791 w811 w823 w829 w885 w929 w972]
      tunnel: [w331 w424 w430 w449 w456 w462 w467 w484 w491 w499 w518 w524 w529 w540 w549 w595 w608 w622 w627 w633 w645 w649 w652 w679 w737 w760 w766 w770 w792 w810 w824 w838 w870 w936 w969] -> w315
      tunnel: [_ _ _ _ _ TRUE _ _ _ _ _ _ _ _ _ _ _ _ _ _ _ _ _ _ _ _ _ _ _ _ _ _ _ _ _] -> w314
      tunnel: [w333 w422 w429 w439 w454 w461 w465 w469 w489 w496 w515 w523 w527 w533 w545 w594 w606 w619 w625 w631 w643 w647 w658 w678 w735 w756 w764 w772 w786 w808 w817 w837 w880 w931 w971] -> w313
      tunnel: w311 -> [w335 _ _ _ _ _ _ _ _ _ _ _ _ _ _ _ _ _ _ _ _ _ _ _ _ _ _ _ _ _ _ _ _ _ _]
      tunnel: w305 -> [w330 _ _ _ _ _ _ _ _ _ _ _ _ _ _ _ _ _ _ _ _ _ _ _ _ _ _ _ _ _ _ w830 _ _ _]
      tunnel: w304 -> [_ _ _ _ _ _ _ w476 _ _ _ _ _ _ _ _ _ _ _ _ _ _ _ _ _ _ _ _ _ _ _ _ _ _ _]
      tunnel: [w329 w421 w426 w438 w451 w458 w464 w478 w487 w493 w510 w519 w526 w531 w542 w590 w602 w614 w624 w629 w635 w646 w651 w669 w728 w755 w763 w768 w779 w804 w818 w836 w872 w930 w968] -> w303
      tunnel: w302 -> [w329 w421 w426 w438 w451 w458 w464 w478 w487 w493 w510 w519 w526 w531 w542 w590 w602 w614 w624 w629 w635 w646 w651 w668 w728 w755 w763 w768 w779 w804 w818 w836 w872 w930 w968]
      tunnel: w301 -> [_ _ _ _ _ _ _ w477 _ _ _ _ _ _ _ _ _ _ _ _ _ _ _ _ _ _ _ _ _ _ _ _ _ _ _]
      tunnel: w300 -> [_ _ _ _ _ _ _ w474 _ _ _ _ _ _ _ _ _ _ _ _ _ _ _ _ _ _ _ _ _ _ _ _ _ _ _]
      tunnel: w299 -> [_ _ _ _ _ _ _ _ _ _ _ _ _ _ _ _ _ _ _ _ _ _ _ _ _ _ _ _ _ _ _ w831 _ _ _]
      tunnel: w298 -> [_ _ _ _ _ _ _ _ _ _ _ _ _ _ _ _ _ _ _ _ _ _ _ _ w727 _ _ _ _ _ _ _ _ _ _]
      frame "", "Idle" {
        n107 = event shown="[1] <Data>: User Event" {
          selector: w330 -> [_ w363 _ _]
          dyn-events: [_ w362 _ _] -> _
          timeout: w335 -> [_ _ _ _]
          tunnel: w334 -> [w340 w355 w399 w409]
          tunnel: [w339 w344 w397 w407] -> w336
          tunnel: w337 -> [w339 w359 w398 w408]
          tunnel: [w340 w354 w399 w409] -> w333
          tunnel: w332 -> [w341 w360 w400 w410]
          tunnel: [w342 w378 w400 w410] -> w331
          event Timeout {
            n108 = event-data() -> ()  [unwired: 1 in, 3 out]
            n109 = call <vilib>:"Add State(s) to Queue__jki_lib_state_machine.vi"("State(s) in Front (\"\")"="Open Front Panel" ("State(s) in Front (\"\")"), "State(s) in (\"\")"=w341) -> ("States Out"=w342:string)  [unwired: 13 in]
          }
          event User Event {
            n110 = event-data() -> ("Message"=w366:string, "Source"=w373:u8, "Destination"=w371:u8, "Command"=w369:u8)  [unwired: 1 in]
            n111 = Unbundle By Name(w355) -> ("Timers"=w353:T43, "File Paths Out"=w347:T21, "GEA Information Out"=w357:T2)
            n112 = To Unsigned Byte Integer(number=w371) -> (unsigned 8bit integer=w370:u8)
            n113 = To Unsigned Byte Integer(number=w369) -> (unsigned 8bit integer=w368:u8)
            n114 = To Unsigned Byte Integer(number=w373) -> (unsigned 8bit integer=w372:u8)
            n115 = Bundle By Name(cluster=T18 {"Source"=0, "Destination"=0, "Command"=0, "Message"=""} ("GEA2 Data In"), "Message"=w366, "Source"=w372, "Destination"=w370, "Command"=w368) -> (w365:T18)
            n116 = call "HCC Process Event Data.vi"("GEA Information Out in"=w357, "File Locations Out"=w347, "Timers in"=w353, "GEA2 Data In"=w365, "error in (no error)"=w359, "Display Bus Log"="Display Bus Log") -> ("SM States"=w375:string, "Elapsed Time (sec)"=→"Newfi Timer":dbl, "Timers out"=w351:T43, "Check Path"=w376:bool, "GEA Information Out out"=w356:T2, "Bus Data"=w346:string, "error out"=w361:errorcluster)  [unwired: 3 in]
            "Check Path" <- w376
            n117 = call "UTILITY AutoScroll DEBUG and BUS.vi"("Input Data"=w346, "Debug Data"="Bus Data") -> ("Text Scroll Position"=w350:i32, "Output Limit"=w349:string)  [unwired: 8 in]
            n118 = case shown="True" w376 {
              tunnel: ["" "Check File Name\nGet Diagnostic Data"] -> w377
              tunnel: w363 -> [w387 w395]
              tunnel: [w387 w393] -> w362
              tunnel: w361 -> [w386 w392]
              tunnel: [w386 w391] -> w345
              frame False {
              }
              frame True {
                n119 = Flush Event Queue(0:w395, 2:lveventtype."User Event" ("event type or object"), 3:w392, 5:1 ("keep most recent")) -> (8:w393:refnum<event-registration>, 9:→"Number of events discarded":u32, 11:w391:errorcluster)  [unwired: 2 in]
              }
            }
            n120 = property on="Bus Data" class="Str"("Text.Scroll Position"=w350) -> ()  [unwired: 2 in, 2 out]
            n121 = property on="Bus Data" class="Str"("Value"=w349) -> ()  [unwired: 2 in, 2 out]
            n122 = call <vilib>:"Add State(s) to Queue__jki_lib_state_machine.vi"("State(s) in Front (\"\")"="Check UI Event\nOpen Front Panel\nCheck Timer" ("State(s) in Front (\"\")"), "State(s) in (\"\")"=w375) -> ("States Out"=w374:string)  [unwired: 13 in]
            n123 = local read "Save Data"() -> (w343:bool)
            n124 = Bundle By Name(cluster=w355, "Timers"=w351, "GEA Information Out"=w356) -> (w354:T44)
            n125 = call <vilib>:"Add State(s) to Queue__jki_lib_state_machine.vi"("State(s) in Front (\"\")"=w374, "State(s) in (\"\")"=w360, "State(s) at Back (\"\")"=w377) -> ("States Out"=w378:string)  [unwired: 12 in]
            n126 = case shown="True" w343 {
              tunnel: w347 -> [_ w385]
              tunnel: w346 -> [_ w384]
              tunnel: w345 -> [w379 w381]
              tunnel: [w379 w380] -> w344
              frame False {
              }
              frame True {
                n127 = Unbundle By Name(w385) -> ("Data File Paths.Bus Log Path"=w382:path)
                n128 = call <vilib>:"Write Spreadsheet String.vi"("error in"=w381, "append to file? (new file:F)"=TRUE, "spreadsheet string"=w384, "file path (dialog if empty)"=w382) -> ("error out"=w380:errorcluster)  [unwired: 6 in, 1 out]
              }
            }
          }
          event Panel Close; Application Instance Close {
            n129 = event-data() -> ()  [unwired: 1 in, 3 out]
            n130 = Unbundle By Name(w399) -> ("Core.Current VI Reference"=w405:refnum<vi>)
            n131 = invoke class="VI" method="FP.Open"(reference=w405, error in=w398, "Activate"=TRUE ("Activate?"), "State"=T39."Hidden") -> (reference out=w403:refnum<vi>, error out=w404:errorcluster)  [unwired: 1 in, 3 out]
            n132 = Close Reference(reference=w403, error in (no error)=w404) -> (error out=w397:errorcluster)
          }
          event Panel Resize {
            n133 = event-data() -> ("Act"=w406:T45)  [unwired: 1 in, 7 out]
            n134 = case shown="\"Minimized\", Default" w406 {
              tunnel: w409 -> [w414 _ _]
              tunnel: w408 -> [w412 w419 w420]
              tunnel: [w411 w419 w420] -> w407
              frame "Minimized", Default {
                n135 = Unbundle By Name(w414) -> ("Core.Current VI Reference"=w413:refnum<vi>)
                n136 = invoke class="VI" method="FP.Open"(reference=w413, error in=w412, "Activate"=TRUE ("Activate?"), "State"=T39."Hidden") -> (reference out=w417:refnum<vi>, error out=w418:errorcluster)  [unwired: 1 in, 3 out]
                n137 = Close Reference(reference=w417, error in (no error)=w418) -> (error out=w411:errorcluster)
              }
              frame "Maximized" {
              }
              frame "Resized" {
              }
            }
          }
        }
      }
      frame "---------- Core ----------" {
        # "Do not put any code in this frame.\n(it is a separator no-op)"
        n138 = call <vilib>:"Add State(s) to Queue__jki_lib_state_machine.vi"("State(s) in (\"\")"=w425) -> ("States Out"=w424:string)  [unwired: 14 in]
      }
      frame Default {
        w436 = 42 items=["No error", "Argument error", "Memory is full", "Out of zone", "End of file", "File already open", "Generic file I/O error", "File not found", "File permission error", "Disk is full", "Duplicate path", "Too many files open", "System feature not enabled", "Resource file not found", "Cannot add resource", "Resource not found", "Image not found", "Image memory error", "Pen does not exist", "Config type invalid", "Config token not found", "Config parse error", "Config memory error", "Bad external code format", "Bad external code offset", "External code not present", "Null window", "Destroy window error", "Null menu", "Print aborted", "Bad print record", "Print driver error", "Windows error during printing", "Memory error during printing", "Print dialog error", "Generic print error", "Invalid device refnum", "Device not found", "Device parameter error", "Device unit error", "Cannot open device", "Device call aborted", "Generic error", "Cancelled by user", "Object ID too low", "Object ID too high", "Object not in heap", "Unknown heap", "Unknown object (invalid DefProc)", "Unknown object (DefProc not in table)", "Message out of range", "Invalid (null) method", "Unknown message", "Manager call not supported", "Bad address", "Network operation in progress", "Network operation timed out", "Connection is busy", "Network attribute not supported", "Network error", "Address in use", "System out of memory", "Connection aborted", "Connection refused", "Not connected", "Already connected", "Connection closed", "Initialization error (interapplication manager)", "Bad occurrence", "Wait on unbound occurrence handler", "Occurrence queue overflow", "Datalog type conflict", "Unused", "Unrecognized type (interapplication manager)", "Memory corrupt", "Failed to make temporary DLL", "Old CIN version", "Drag socket not found", "Failed to load drop-object", "Failed to register OLE object", "Failed to release OLE object", "Format specifier type mismatch", "Unknown format specifier", "Too few format specifiers", "Too many format specifiers", "Scan failed", "Newer CIN version", "Error converting to variant", "Runtime menu error", "Password tampered", "Variant attribute not found", "Incompatible variant data type", "Event data is not available", "Event Store is not present", "Occurrence is not found", "Event Queue is not created", "Event info is not available", "Refnum passed is NULL", "Error retrieving Class GUID", "Error retrieving CoClass GUID", "Error retrieving TypeLib GUID.", "Bad built application magic bytes.", "Specific driver is different from the specific driver associated with the Logical Name.", "There is no session opened to the class driver.", "Max Error", "MAX - Error with config objects", "MAX - Error loading configuration", "MAX - Group not supported"]
        # "Current State"
        # "Handle mistyped state name (developer tool)"
        n139 = Format Into String(format string="Software Exception: Unhandled State \"%s\"." ("message"), error in=w432, w427) -> (resulting string=w435:string, error out=w434:errorcluster)  [unwired: 1 in]
        n140 = call <vilib>:"Error Cluster From Error Code.vi"("show call chain? (False)"=TRUE, "error in (no error)"=w434, "error message (\"\")"=w435, "error code (0)"=w436) -> ("error out"=w433:errorcluster)  [unwired: 5 in]
        n141 = call <vilib>:"Add State(s) to Queue__jki_lib_state_machine.vi"("State(s) in (\"\")"=w431) -> ("States Out"=w430:string)  [unwired: 14 in]
      }
      frame "Initialize Core Data" {
        # "If panel starts closed or is an EXE, then close it when we exit"
        n142 = property class="VI"() -> ("Front Panel.Open"=w441:bool)  [unwired: 2 in, 2 out]
        n143 = property class="App"() -> ("App.Kind"=w442:T40)  [unwired: 2 in, 2 out]
        n144 = control-ref of="Current VI Reference"() -> (w447:refnum<vi>)
        n145 = Not(x=w441) -> (.not. x?=w444:bool)
        n146 = Equal?(x=w442, y=T40."Run Time System" ("Application:Kind")) -> (x = y?=w445:bool)
        n147 = Or(x=w444, y=w445) -> (x .or. y?=w446:bool)
        n148 = Bundle By Name(cluster=w440, "Core.Current VI Reference"=w447, "Core.Close Panel on Exit?"=w446) -> (w439:T44)
        n149 = call <vilib>:"Add State(s) to Queue__jki_lib_state_machine.vi"("State(s) in (\"\")"=w450) -> ("States Out"=w449:string)  [unwired: 14 in]
      }
      frame "Error Handler" {
        # "Unhandled Error -- Display it"
        # "Clear error"
        n150 = call <vilib>:"General Error Handler.vi"("error in (no error)"=w453) -> ()  [unwired: 10 in, 5 out]
        n151 = call <vilib>:"Add State(s) to Queue__jki_lib_state_machine.vi"("State(s) in Front (\"\")"="/* Post Error States", "State(s) in (\"\")"=w457) -> ("States Out"=w456:string)  [unwired: 13 in]
      }
      frame "Exit" {
        n152 = call <vilib>:"Add State(s) to Queue__jki_lib_state_machine.vi"("State(s) in (\"\")"=w463) -> ("States Out"=w462:string)  [unwired: 14 in]
      }
      frame "------ Startup and Save ------" {
        n153 = call <vilib>:"Add State(s) to Queue__jki_lib_state_machine.vi"("State(s) in (\"\")"=w468) -> ("States Out"=w467:string)  [unwired: 14 in]
      }
      frame "Data: Initialize" {
        w472 = T25 {"RPM Max"=0, "Cycle Time"=0.0, "IGBT Temperature"=0.0, "Load Size"=0.0, "Temperature"=0.0, "Water Pressure"=0.0, "Detergent"=0.0, "Fabric Softener"=0.0, "Inverter Power (W)"=0.0, "Raw OOB"=0.0, "Current Motor Temp (Deg C)"=0.0}  # Cycle Stats
        w473 = T43 {"Cycle Timer"=0.0, "Timer"=0.0}  # Timers
        (unwired) T46 {"IGBT Temp (Deg C)"=0, "Speed"=0, "Load Size"=0, "Temperature"=0, "Water Pressure"=0, "Detergent"=0, "Fabric Softener"=0, "Direction"="", "Det"=FALSE, "FS"=FALSE, "Recirc"=FALSE, "Drain"=FALSE, "Hot"=FALSE, "Cold"=FALSE, "LidClosed"=FALSE, "LidLocked"=FALSE, "Motor Speed"=0, "Latched Out Of Balance"=0, "Raw Out Of Balance"=0, "Plaster Status"=0, "Inverter Power (Watts)"=0, "Profiler Status"="", "Profiler CRC"=0, "Current Inverter Action"="", "Target Speed (BRPM)"=0, "Latched Agitate Motor Temp (Deg C)"=0, "Current Motor Temp (Deg C)"=0, "Error Codes 1"=""} ("logData")
        n154 = Bundle("Core"=T41 {"Current VI Reference"=refnum, "Close Panel on Exit?"=FALSE}, "GEA Information Out"=w477, "Main Washer Display Out"=w474, "File Paths Out"=w476, "Timers"=w473, "Cycle Stats"=w472, "Cycles/ File"="Cycles/ File") -> (w471:T44)  [unwired: 1 in]
        n155 = Current VI's Path() -> (path=w481:path)
        n156 = call "UTILITY This VIs Path.vi"("path"=w481, "error in (no error)"=w480) -> ("FileVersionInfo Out"=w470:T28, "error out"=w479:errorcluster)  [unwired: 7 in, 5 out]
        n157 = Unbundle By Name(w470) -> ("FileVersion"=→"File  Version":string)
        n158 = Bundle By Name(cluster=w471, "Main Washer Display Out.Appliance Details.FileVersionInfo"=w470) -> (w469:T44)
        n159 = call <vilib>:"Add State(s) to Queue__jki_lib_state_machine.vi"("State(s) in (\"\")"=w485) -> ("States Out"=w484:string)  [unwired: 14 in]
      }
      frame "Add Header" {
        # "Clear array to conserve on \nmemory"
        # "Add notes and calibration to the header"
        n160 = Bundle By Name(cluster=w486, "GEA Information Out.Bus Data"="" ("Bus Data")) -> (w489:T44)
        n161 = call <vilib>:"Add State(s) to Queue__jki_lib_state_machine.vi"("State(s) in (\"\")"=w492) -> ("States Out"=w491:string)  [unwired: 14 in]
      }
      frame "Prepare For Save" {
        # "Add notes and calibration to the header"
        n162 = flat-sequence {
          tunnel: w496 -> [w505]
          tunnel: w495 -> [w502]
          tunnel: [w501] -> w498
          tunnel: [w504] -> w497
          tunnel: [w507] -> w494
          tunnel: w498 -> [w507]
          tunnel: w497 -> [w506]
          frame #0 {
            n163 = Unbundle By Name(w505) -> ("File Paths Out"=w504:T21)
            n164 = call "UTILITY Delay mS.vi"("Error In"=w502, "milliseconds to wait"=u32 1000) -> ("Error Out"=w501:errorcluster)  [unwired: 13 in]
          }
          frame #1 {
            n165 = local write "File Locations In"(w506) -> ()
          }
        }
        n166 = call <vilib>:"Add State(s) to Queue__jki_lib_state_machine.vi"("State(s) in (\"\")"=w500) -> ("States Out"=w499:string)  [unwired: 14 in]
      }
      frame "Cluster Write" {
        (unwired) T46 {"IGBT Temp (Deg C)"=0, "Speed"=0, "Load Size"=0, "Temperature"=0, "Water Pressure"=0, "Detergent"=0, "Fabric Softener"=0, "Direction"="", "Det"=FALSE, "FS"=FALSE, "Recirc"=FALSE, "Drain"=FALSE, "Hot"=FALSE, "Cold"=FALSE, "LidClosed"=FALSE, "LidLocked"=FALSE, "Motor Speed"=0, "Latched Out Of Balance"=0, "Raw Out Of Balance"=0, "Plaster Status"=0, "Inverter Power (Watts)"=0, "Profiler Status"="", "Profiler CRC"=0, "Current Inverter Action"="", "Target Speed (BRPM)"=0, "Latched Agitate Motor Temp (Deg C)"=0, "Current Motor Temp (Deg C)"=0, "Error Codes 1"=""} ("logData")
        n167 = Unbundle By Name(w516) -> ("Timers.Timer"=w511:dbl, "File Paths Out"=w508:T21)
        n168 = Bundle By Name(cluster=w516, "Main Washer Display Out.Display Data (RLT).Total Time On Display"=w511) -> (w515:T44)
        n169 = Unbundle By Name(w515) -> ("Main Washer Display Out"=w512:T26)
        n170 = call "HCC Read Write Display.vi"("Read Write Control"=enum16{"Read", "Write"}."Write", "error in (no error)"=w514, "Washer Input"=w512, "File Locations In"=w508) -> ("error out"=w513:errorcluster)  [unwired: 6 in, 1 out]
        n171 = call <vilib>:"Add State(s) to Queue__jki_lib_state_machine.vi"("State(s) in (\"\")"=w517) -> ("States Out"=w518:string)  [unwired: 14 in]
      }
      frame "Data: Cleanup" {
        n172 = Unbundle By Name(w523) -> ("Core.Current VI Reference"=w522:refnum<vi>)
        n173 = Close Reference(reference=w522, error in (no error)=w520) -> (error out=w521:errorcluster)
        n174 = call <vilib>:"Add State(s) to Queue__jki_lib_state_machine.vi"("State(s) in (\"\")"=w525) -> ("States Out"=w524:string)  [unwired: 14 in]
      }
      frame "---------- UI Events ----------" {
        n175 = call <vilib>:"Add State(s) to Queue__jki_lib_state_machine.vi"("State(s) in (\"\")"=w530) -> ("States Out"=w529:string)  [unwired: 14 in]
      }
      frame "UI: Initialize" {
        w532 = T47."Disabled" ("Disabled")
        n176 = Unbundle By Name(w533) -> ("GEA Information Out.Board ID"=→"Board ID.":string, "Main Washer Display Out.Display Data (RLT).Station Label Display"=→"Front Panel Station Label":string)
        n177 = property on="Serial Number Front Panel" class="Str"("DisabledEnum"=w532) -> ()  [unwired: 2 in, 2 out]
        n178 = property on="Lab ID Front Panel" class="Str"("DisabledEnum"=w532) -> ()  [unwired: 2 in, 2 out]
        n179 = property on="TR Number  Front Panel" class="Str"("DisabledEnum"=w532) -> ()  [unwired: 2 in, 2 out]
        n180 = Unbundle By Name(w533) -> ("Main Washer Display Out.Appliance Details.Appliance Common.Serial Number:"=w534:string, "Main Washer Display Out.Appliance Details.Appliance Common.TR Number:"=w536:string, "Main Washer Display Out.Appliance Details.Appliance Common.Lab ID:"=w535:string)
        n181 = local write "Serial Number Front Panel"(w534) -> ()
        n182 = local write "Lab ID Front Panel"(w535) -> ()
        n183 = local write "TR Number  Front Panel"(w536) -> ()
        n184 = call <vilib>:"Add State(s) to Queue__jki_lib_state_machine.vi"("State(s) in (\"\")"=w541) -> ("States Out"=w540:string)  [unwired: 14 in]
      }
      frame "UI: Front Panel State" {
        # "Argument"
        n185 = Unbundle By Name(w545) -> ("Core.Current VI Reference"=w548:refnum<vi>)
        n186 = case shown="\"Close\"" w544 {
          tunnel: w547 -> [w554 w584]
          tunnel: [w556 w585] -> w546
          tunnel: w548 -> [w555 w582]
          frame "Open", Default {
            n187 = property class="VI"(reference=w555, error in=w554) -> (reference out=w552:refnum<vi>, error out=w553:errorcluster, "Front Panel.Open"=w551:bool)
            n188 = case shown="True" w551 {
              tunnel: [w566 w573] -> w556
              tunnel: w553 -> [w571 w577]
              tunnel: w552 -> [w572 w576]
              frame False {
                w563 = 0 items=["NULL"]
                # "Windows API to bring the LaundryLab.vi screen\nto the front. It also allows you to rename the vi, therefore\nbeing a dynamic file name. (You have to rename for\nit to work)"
                n189 = Current VI's Path() -> (path=w562:path)
                n190 = Open VI Reference(vi path=w562) -> (vi reference=w561:refnum<vi>, error out=w558:errorcluster)  [unwired: 5 in]
                n191 = property class="VI"(reference=w561, error in=w558) -> (reference out=w560:refnum<vi>, error out=w559:errorcluster, "Name"=w557:string)
                n192 = Close Reference(reference=w560, error in (no error)=w559) -> ()  [unwired: 1 out]
                n193 = invoke class="VI" method="FP.Open"(reference=w572, error in=w571, "Activate"=TRUE ("Activate?"), "State"=T39."Maximized") -> (reference out=w569:refnum<vi>, error out=w570:errorcluster)  [unwired: 1 in, 3 out]
                n194 = dll-call lib="user32.dll" fn="FindWindowA" label="FindWindow"("lpszClassName"=w563, "lpszWindowName"=w557) -> ("hWnd"=w564:u32)  [unwired: 4 in, 3 out]
                "Handle" <- w564
                n195 = Close Reference(reference=w569, error in (no error)=w570) -> (error out=w566:errorcluster)
                n196 = dll-call lib="user32.dll" fn="SetForegroundWindow"("Handle"=w564) -> (→"Error":i32)  [unwired: 4 in, 2 out]
              }
              frame True {
                n197 = invoke class="VI" method="FP.Open"(reference=w576, error in=w577, "Activate"=TRUE, "State"=T39."Maximized") -> (reference out=w575:refnum<vi>, error out=w574:errorcluster)  [unwired: 1 in, 3 out]
                n198 = Close Reference(reference=w575, error in (no error)=w574) -> (error out=w573:errorcluster)
              }
            }
          }
          frame "Close" {
            n199 = property class="VI"(reference=w582, error in=w584) -> (reference out=w581:refnum<vi>, error out=w583:errorcluster, "Front Panel.Open"=w580:bool)
            n200 = case shown="True" w580 {
              tunnel: [w586 w589] -> w585
              tunnel: w583 -> [w586 w588]
              tunnel: w581 -> [_ w587]
              frame False {
              }
              frame True {
                n201 = invoke class="VI" method="FP.Close"(reference=w587, error in=w588) -> (error out=w589:errorcluster)  [unwired: 1 in, 2 out]
              }
            }
          }
        }
        n202 = call <vilib>:"Add State(s) to Queue__jki_lib_state_machine.vi"("State(s) in (\"\")"=w550) -> ("States Out"=w549:string)  [unwired: 14 in]
        "Start UI Loop" <- TRUE ("Start UI Loop")
      }
      frame "UI: Cursor Set" {
        # "Argument"
        n203 = case shown="\"Idle\", Default" w591 {
          tunnel: w593 -> [w598 w600]
          tunnel: [w597 w599] -> w592
          frame "Idle", Default {
            n204 = call <vilib>:"Unset Busy.vi"("error in (no error)"=w598) -> ("error out"=w597:errorcluster)  [unwired: 10 in]
          }
          frame "Busy" {
            n205 = call <vilib>:"Set Busy.vi"("error in (no error)"=w600) -> ("error out"=w599:errorcluster)  [unwired: 9 in, 1 out]
          }
        }
        n206 = call <vilib>:"Add State(s) to Queue__jki_lib_state_machine.vi"("State(s) in (\"\")"=w596) -> ("States Out"=w595:string)  [unwired: 14 in]
      }
      frame "Reset Cycle Stats" {
        # "This make the debug log run...it will then update the caller  program"
        n207 = flat-sequence {
          tunnel: w604 -> [w610]
          tunnel: [w610] -> w605
          tunnel: [w612] -> w603
          tunnel: w605 -> [w612]
          frame #0 {
            n208 = local write "Full Message to Save"("Resetting Cycle Stats..." ("Front Panel Status Read")) -> ()
          }
          frame #1 {
            n209 = local write "Status"("") -> ()
          }
        }
        n210 = Bundle By Name(cluster=w607, "Cycle Stats"=T25 {"RPM Max"=0, "Cycle Time"=0.0, "IGBT Temperature"=0.0, "Load Size"=0.0, "Temperature"=0.0, "Water Pressure"=0.0, "Detergent"=0.0, "Fabric Softener"=0.0, "Inverter Power (W)"=0.0, "Raw OOB"=0.0, "Current Motor Temp (Deg C)"=0.0} ("Cycle Stats Update")) -> (w606:T44)
        n211 = call <vilib>:"Add State(s) to Queue__jki_lib_state_machine.vi"("State(s) in (\"\")"=w609) -> ("States Out"=w608:string)  [unwired: 14 in]
      }
      frame "Reset Timer" {
        n212 = call "UTILITY E-Time.vi"("Set Start Time (s)"=0.0, "Reset"=TRUE) -> ("Elapsed Time (sec)"=w616:dbl)  [unwired: 7 in, 2 out]
        n213 = local write "Status"("Resetting Timer...") -> ()
        n214 = local write "Newfi Timer"(w616) -> ()
        n215 = Bundle By Name(cluster=w620, "Timers.Cycle Timer"=w616) -> (w619:T44)
        n216 = call <vilib>:"Add State(s) to Queue__jki_lib_state_machine.vi"("State(s) in (\"\")"=w623) -> ("States Out"=w622:string)  [unwired: 14 in]
      }
      frame "---------- Macro ----------" {
        # "Do not put any code in this frame.\n(It is a separator no-op. You can make a copy of this frame to create a new Macro frame)"
        n217 = call <vilib>:"Add State(s) to Queue__jki_lib_state_machine.vi"("State(s) in (\"\")"=w628) -> ("States Out"=w627:string)  [unwired: 14 in]
      }
      frame "Macro: Initialize" {
        # "Initialization Macro\n(This is called once, when the VI starts)"
        n218 = call <vilib>:"Add State(s) to Queue__jki_lib_state_machine.vi"("State(s) in Front (\"\")"="Data: Initialize\nAdd Header\nInitialize Core Data\nUI: Initialize\nUI: Front Panel State >> Open", "State(s) in (\"\")"=w634) -> ("States Out"=w633:string)  [unwired: 13 in]
      }
      frame "Macro: Exit" {
        # "Exit Macro\n(This is called once, when the VI exits)"
        n219 = Unbundle By Name(w643) -> ("Core.Close Panel on Exit?"=w640:bool)
        n220 = Select(t="UI: Front Panel State >> Close", s=w640, f="") -> (s? t:f=w637:string)
        n221 = call <vilib>:"Add State(s) to Queue__jki_lib_state_machine.vi"("State(s) in (\"\")"=w637, "State(s) at Back (\"\")"="Data: Cleanup\nExit") -> ("States Out"=w636:string)  [unwired: 13 in]
        n222 = call <vilib>:"Add State(s) to Queue__jki_lib_state_machine.vi"("State(s) in Front (\"\")"=w636, "State(s) in (\"\")"=w639) -> ("States Out"=w645:string)  [unwired: 13 in]
      }
      frame "---------- Main ----------" {
        # "Template Separator\n(You can make a copy of, or modify, this frame)"
        n223 = call <vilib>:"Add State(s) to Queue__jki_lib_state_machine.vi"("State(s) in (\"\")"=w650) -> ("States Out"=w649:string)  [unwired: 14 in]
      }
      frame "Check UI Event" {
        # "Clears the UI variable after execution (prevents from running routine twice)"
        n224 = flat-sequence {
          tunnel: w657 -> [w662]
          tunnel: [w662] -> w655
          tunnel: w654 -> [w661]
          tunnel: [w660] -> w653
          tunnel: [w665] -> w656
          tunnel: w655 -> [w665]
          tunnel: [w664] -> w652
          tunnel: w653 -> [w664]
          frame #0 {
            n225 = call <vilib>:"Add State(s) to Queue__jki_lib_state_machine.vi"("State(s) in Front (\"\")"="UI Event SM", "State(s) in (\"\")"=w661) -> ("States Out"=w660:string)  [unwired: 13 in]
          }
          frame #1 {
            n226 = local write "UI Event SM"("" ("UI Event")) -> ()
          }
        }
      }
      frame "Check File Name" {
        # "Checks the date/time/serial/lab ID and TR for a change. If detected it will create a\nnew folder and file. After it creates a new file it will send it to the \"Add Header to Files\"\nsection of the code to add a header."
        # "Check if the Serial Number, Lab ID, TR Number , Cycle Count Save Interval\nhas occurred. If so, create the new save path and associated folders."
        n227 = Unbundle By Name(w674) -> ("File Paths Out"=w677:T21, "Main Washer Display Out"=w670:T26, "Cycles/ File"=w676:i32)
        n228 = local read "Save Data"() -> (w666:bool)
        n229 = case shown="True" w666 {
          tunnel: w677 -> [w683 w691]
          tunnel: w676 -> [_ w690]
          tunnel: [w683 w689] -> w675
          tunnel: [FALSE ("New File?") w688] -> w672
          tunnel: w671 -> [w682 w687]
          tunnel: w670 -> [_ w686]
          tunnel: [w682 w684] -> w667
          frame False {
          }
          frame True {
            n230 = First Call?() -> (First Call?: T/F=w685:bool)
            n231 = case shown="False" w685 {
              tunnel: w691 -> [w701 w719]
              tunnel: w690 -> [w700 _]
              tunnel: [w694 FALSE ("New File?")] -> w688
              tunnel: [w696 w718] -> w689
              tunnel: w687 -> [w699 w717]
              tunnel: [w697 w716] -> w684
              tunnel: w686 -> [w692 w712]
              frame False {
                n232 = call "Save File Format All Folders.vi"("Number of Cycles/ File"=w700, "LV Program"=Save_File_DOE_LabView_Program."HCC", "error in (no error)"=w699, "Initialize.Washer In"=w692, "File Locations In"=w701) -> ("error out"=w698:errorcluster, "New File?"=w694:bool, "File Locations Out"=w695:T21)  [unwired: 4 in]
                n233 = case shown="True" w694 {
                  tunnel: w698 -> [w702 w711]
                  tunnel: [w702 w710] -> w697
                  tunnel: [w703 w709] -> w696
                  tunnel: w695 -> [w703 w708]
                  tunnel: w692 -> [_ w704]
                  frame False {
                  }
                  frame True {
                    n234 = local read "GEA Data"() -> (w707:string[][])
                    n235 = Index Array(array=w707, index (col)=0 ("disabled index (col)")) -> (element=w705:string[])  [unwired: 1 in]
                    n236 = call "Save File Write Headers.vi"("Error In"=w711, "GEA Headers"=w705, "Main Washer Display Out"=w704, "File Paths In"=w708) -> ("error out"=w710:errorcluster, "File Paths Out"=w709:T21)  [unwired: 6 in]
                  }
                }
              }
              frame True {
                n237 = local read "GEA Data"() -> (w715:string[][])
                n238 = Index Array(array=w715, index (col)=0 ("disabled index (col)")) -> (element=w713:string[])  [unwired: 1 in]
                n239 = call "Save File Write Headers.vi"("Error In"=w717, "GEA Headers"=w713, "Main Washer Display Out"=w712, "File Paths In"=w719) -> ("error out"=w716:errorcluster, "File Paths Out"=w718:T21)  [unwired: 6 in]
              }
            }
          }
        }
        "New File Created" <- w672
        n240 = case shown="True" w672 {
          tunnel: ["" "Cluster Write\nPrepare For Save"] -> w673
          tunnel: [w721 w724] -> w669
          tunnel: w668 -> [w721 w723]
          frame False {
          }
          frame True {
            # "Only trigger on True"
            n241 = Generate User Event(user event=w723, event data cluster=TRUE ("Trigger")) -> (user event out=w724:refnum<user-event>)  [unwired: 2 in, 1 out]
          }
        }
        n242 = Bundle By Name(cluster=w674, "File Paths Out"=w675) -> (w678:T44)
        n243 = call <vilib>:"Add State(s) to Queue__jki_lib_state_machine.vi"("State(s) in Front (\"\")"=w673, "State(s) in (\"\")"=w680) -> ("States Out"=w679:string)  [unwired: 13 in]
      }
      frame "Open Front Panel" {
        # "Checks the network variable to see if the user wants to open or exit the\napplication."
        n244 = case shown="2" w727 {
          tunnel: [w741 w742] -> w733
          frame 1, Default {
            n245 = shared-variable ".\\Test Lib.lvlib\\Board ID"() -> (w741:string)  [unwired: 1 in, 1 out]
          }
          frame 2 {
            n246 = shared-variable "My Computer\\Test Lib.lvlib\\Board ID-2"() -> (w742:string)  [unwired: 1 in, 1 out]
          }
        }
        n247 = Unbundle By Name(w735) -> ("GEA Information Out.Board ID"=w734:string)
        n248 = call <vilib>:"Trim Whitespace.vi"("string"=w733) -> ("trimmed string"=w738:string)  [unwired: 1 in]
        n249 = Equal?(x=w734, y=w738) -> (x = y?=w739:bool)
        n250 = case shown="True" w739 {
          tunnel: ["" w750] -> w740
          tunnel: w727 -> [_ w748]
          frame False {
          }
          frame True {
            w750 = "UI: Front Panel State >> Open"  # UI: Front Panel State >> Open
            n251 = case shown="2" w748 {
              tunnel: "" -> [w751 w752]
              frame 1, Default {
                n252 = shared-variable ".\\Test Lib.lvlib\\Board ID"(w751) -> ()  [unwired: 1 in, 1 out]
              }
              frame 2 {
                n253 = shared-variable "My Computer\\Test Lib.lvlib\\Board ID-2"(w752) -> ()  [unwired: 1 in, 1 out]
              }
            }
          }
        }
        n254 = case shown="2" w727 {
          tunnel: [w743 w744] -> w729
          frame 1, Default {
            n255 = shared-variable "My Computer\\Test Lib.lvlib\\Exit"() -> (w743:bool)  [unwired: 1 in, 1 out]
          }
          frame 2 {
            n256 = shared-variable "My Computer\\Test Lib.lvlib\\Exit-2"() -> (w744:bool)  [unwired: 1 in, 1 out]
          }
        }
        n257 = case shown="False" w729 {
          tunnel: ["" "Macro: Exit"] -> w731
          frame False {
          }
          frame True {
          }
        }
        n258 = call <vilib>:"Add State(s) to Queue__jki_lib_state_machine.vi"("State(s) in Front (\"\")"=w731, "State(s) in (\"\")"=w732) -> ("States Out"=w730:string)  [unwired: 13 in]
        n259 = call <vilib>:"Add State(s) to Queue__jki_lib_state_machine.vi"("State(s) in Front (\"\")"=w740, "State(s) in (\"\")"=w730) -> ("States Out"=w737:string)  [unwired: 13 in]
        "Network Var Set" <- w727
      }
      frame "Check Timer" {
        n260 = local read "New File Created"() -> (w754:bool)
        n261 = case shown="False" w754 {
          tunnel: [0.0 ("Set Start Time (s)") 0.0 ("Set Start Time (s)")] -> w753
          frame False {
          }
          frame True {
          }
        }
        n262 = call "UTILITY E-Time.vi"("Set Start Time (s)"=w753, "Reset"=w754) -> ("Elapsed Time (sec)"=→"Cycle Timer":dbl)  [unwired: 7 in, 2 out]
        n263 = call <vilib>:"Add State(s) to Queue__jki_lib_state_machine.vi"("State(s) in (\"\")"=w758) -> ("States Out"=w760:string)  [unwired: 14 in]
      }
      frame "------- GEA2 Routine --------" {
        # "Template Separator\n(You can make a copy of, or modify, this frame)"
        n264 = call <vilib>:"Add State(s) to Queue__jki_lib_state_machine.vi"("State(s) in (\"\")"=w767) -> ("States Out"=w766:string)  [unwired: 14 in]
      }
      frame "Get Remaining Messages" {
        # "Sometimes the debug logs send multiple messages with several \"/n\". This section will \ndetect how many \"/n\" are in the string...and then tell the program to get all of the info\nbefore proceeding.\n\nThis typically happens when the machine outputs alot of information in a small time\ninterval"
        n265 = Unbundle By Name(w773) -> ("GEA Information Out.Partial Message String"=w774:string)
        n266 = call "Nufi Dryer Debug Message Buff.vi"("Partial Message String"=w774) -> ("Partial Message FWD"=w776:string, "Full Message to Save"=w775:string, "Number of Messages"=w769:i32)  [unwired: 6 in, 2 out]
        n267 = Bundle By Name(cluster=w773, "GEA Information Out.Full Message to Save"=w775, "GEA Information Out.Partial Message String"=w776, "GEA Information Out.Number of Messages"=w769) -> (w772:T44)
        n268 = call <vilib>:"Add State(s) to Queue__jki_lib_state_machine.vi"("State(s) in Front (\"\")"="Debug Message" ("State(s) in Front (\"\")"), "State(s) in (\"\")"=w771) -> ("States Out"=w770:string)  [unwired: 13 in]
      }
      frame "Read Debug" {
        # "Reads debug and keeps 5000 characters on file. Once 5000 is reached\nit will override. If there is a message to save it will log to file. If not, it goes \nback through the code to collect more information...unitl \"/n\" is received"
        n269 = Unbundle By Name(w787) -> ("GEA Information Out.Partial Message String"=w788:string, "GEA Information Out.ReceivedData"=w781:u8[])
        n270 = Byte Array To String(unsigned byte array=w781) -> (string=w784:string)
        n271 = case shown="True" "Display Debug" {
          tunnel: w784 -> [_ w797]
          frame False {
          }
          frame True {
            n272 = call "UTILITY AutoScroll DEBUG and BUS.vi"("Input Data"=w797, "Debug Data"="Debug Data") -> ("Text Scroll Position"=w794:i32, "Output Limit"=w795:string)  [unwired: 8 in]
            n273 = property on="Debug Data" class="Str"("Value"=w795) -> ()  [unwired: 2 in, 2 out]
            n274 = property on="Debug Data" class="Str"("Text.Scroll Position"=w794) -> ()  [unwired: 2 in, 2 out]
          }
        }
        n275 = call "Nufi Dryer Debug Message Buff.vi"("New String"=w784, "Partial Message String"=w788) -> ("Partial Message FWD"=w789:string, "Full Message to Save"=w790:string, "Message to Save"=w783:bool, "Number of Messages"=w782:i32)  [unwired: 5 in, 1 out]
        n276 = case shown="True" w783 {
          tunnel: ["" "Debug Message"] -> w785
          frame False {
          }
          frame True {
          }
        }
        n277 = Bundle By Name(cluster=w787, "GEA Information Out.Full Message to Save"=w790, "GEA Information Out.Partial Message String"=w789, "GEA Information Out.Number of Messages"=w782) -> (w786:T44)
        n278 = call <vilib>:"Add State(s) to Queue__jki_lib_state_machine.vi"("State(s) in Front (\"\")"=w785, "State(s) in (\"\")"=w793) -> ("States Out"=w792:string)  [unwired: 13 in]
      }
      frame "Read MC Data" {
        # "Filter Erroneous data"
        # "Update the RPM control"
        # "This is a decoder. It take the numeric array and converts to meaningful info"
        n279 = Unbundle By Name(w809) -> ("GEA Information Out.GEA Diagnostic Data - Washer"=w807:T1, "GEA Information Out.ReceivedData"=w805:u8[])
        n280 = call "ViperHawk_Decode MC Data.vi"("Array"=w805, "Diagnostic Data In"=w807) -> ("Diagnostic Data Out"=w806:T1)  [unwired: 9 in]
        n281 = call "ViperHawk Check and Filter Inv Data.vi"("Enum"=enum16{"Inv Data", "MC Data"}."MC Data", "Diagnostic Data In"=w806) -> ("Diagnostic Data Out"=w803:T1)  [unwired: 9 in]
        n282 = Unbundle By Name(w803) -> ("Speed (RPM)"=w802:u32, "9E Diagnostic Data.Total Cycle Count (Current)"=w801:u16)
        n283 = call <vilib>:"Add State(s) to Queue__jki_lib_state_machine.vi"("State(s) in (\"\")"=w812) -> ("States Out"=w810:string)  [unwired: 14 in]
        n284 = Bundle By Name(cluster=w809, "GEA Information Out.GEA Diagnostic Data - Washer"=w803, "Main Washer Display Out.Display Data (RLT).RPM Display"=w802, "Main Washer Display Out.Display Data (RLT).Cycle Count Display"=w801) -> (w808:T44)
      }
      frame "Read Inv Data" {
        # "Filter Erroneous data"
        # "This is a decoder. It take the numeric array and converts to meaningful info"
        n285 = Unbundle By Name(w821) -> ("GEA Information Out.GEA Diagnostic Data - Washer"=w822:T1, "GEA Information Out.ReceivedData"=w815:u8[], "Main Washer Display Out"=w814:T26)
        n286 = call "ViperHawk_Decode Inv Data.vi"("Washer In"=w814, "Data"=w815, "Diagnostic Data In"=w822) -> ("Washer Out"=w813:T26, "Diagnostic Data Out"=w820:T1)  [unwired: 6 in, 1 out]
        n287 = call "ViperHawk Check and Filter Inv Data.vi"("Enum"=enum16{"Inv Data", "MC Data"}."Inv Data", "Diagnostic Data In"=w820) -> ("Diagnostic Data Out"=w819:T1)  [unwired: 9 in]
        n288 = Bundle By Name(cluster=w821, "GEA Information Out.GEA Diagnostic Data - Washer"=w819, "Main Washer Display Out"=w813) -> (w817:T44)
        n289 = call <vilib>:"Add State(s) to Queue__jki_lib_state_machine.vi"("State(s) in (\"\")"=w825) -> ("States Out"=w824:string)  [unwired: 14 in]
      }
      frame "Get Diagnostic Data" {
        n290 = local read "Enable Diagnostic Data"() -> (w827:T9)
        n291 = case shown="\"\", Default" w827 {
          tunnel: w831 -> [_ w846]
          tunnel: w830 -> [_ w845]
          tunnel: w829 -> [w840 w844]
          tunnel: [w840 w842] -> w828
          tunnel: T13 {"Source"=229, "Destination"=35} ("GEA Inputs") -> [_ w843]
          frame "", Default {
          }
          frame "2015 Washer", "2017 Washer" {
            n292 = case shown="True" "Enable Fault Data" {
              tunnel: w846 -> [_ w856]
              tunnel: w845 -> [_ w855]
              tunnel: w844 -> [w847 w850]
              tunnel: w843 -> [_ w849]
              tunnel: [w847 w848] -> w842
              frame False {
              }
              frame True {
                # "Fault ERDs"
                n293 = call "GEA2 Read ERD Multiple Messages.vi"("GEA2 Reference In"=w856, "Read Timeout (ms)"=u32 250, "GEA Inputs"=w849, "Read ERD List"=T35 [{"ERD Number"=132, "Data Type"=enum."string"}, {"ERD Number"=141, "Data Type"=enum."uint32_t"}, {"ERD Number"=57394, "Data Type"=enum."string"}, {"ERD Number"=57395, "Data Type"=enum."string"}, {"ERD Number"=57396, "Data Type"=enum."string"}, {"ERD Number"=57397, "Data Type"=enum."string"}, {"ERD Number"=57398, "Data Type"=enum."string"}, {"ERD Number"=57399, "Data Type"=enum."string"}, {"ERD Number"=57400, "Data Type"=enum."string"}, {"ERD Number"=57401, "Data Type"=enum."string"}, {"ERD Number"=57402, "Data Type"=enum."string"}, {"ERD Number"=57403, "Data Type"=enum."string"}, {"ERD Number"=57404, "Data Type"=enum."string"}, {"ERD Number"=57405, "Data Type"=enum."string"}, {"ERD Number"=57406, "Data Type"=enum."string"}, {"ERD Number"=57407, "Data Type"=enum."string"}, {"ERD Number"=57408, "Data Type"=enum."string"}, {"ERD Number"=129, "Data Type"=enum."string"}, {"ERD Number"=57444, "Data Type"=enum."string"}, {"ERD Number"=57445, "Data Type"=enum."string"}, {"ERD Number"=57446, "Data Type"=enum."string"}, {"ERD Number"=57447, "Data Type"=enum."string"}, {"ERD Number"=57448, "Data Type"=enum."string"}, {"ERD Number"=57449, "Data Type"=enum."string"}, {"ERD Number"=57450, "Data Type"=enum."string"}, {"ERD Number"=57451, "Data Type"=enum."string"}, {"ERD Number"=57452, "Data Type"=enum."string"}, {"ERD Number"=57453, "Data Type"=enum."string"}], "GEA2 Event Registration"=w855, "Error In"=w850, "#ERDs per message"=14, "Verify ERD Response?"=FALSE) -> ("ERD Data Out"=w853:T17[], "Error Out"=w848:errorcluster)  [unwired: 3 in, 3 out]
                n294 = Array Subset(array=w853, index=0, length=17) -> (w852:T17[])
                n295 = Array Subset(array=w853, index=17, length=11) -> (w851:T17[])
                n296 = call "Fault_Seq_Read.vi"("Seq ERD In"=w852) -> ("Seq Buffer Status"=→"Seq Buffer Status":T11, "String"=→"Fault Sequence Buffer":string)  [unwired: 13 in]
                n297 = call "Fault_Table_Read.vi"("ERD Data Out"=w851) -> ("Fault Set?"=→"Fault Set?":bool, "Table Buffer Status"=→"Table Buffer Status":T11, "Fault Table String Out"=→"Fault Table Buffer":string[][])  [unwired: 11 in, 1 out]
              }
            }
          }
        }
        n298 = local read "Diagnostic Data Local"() -> (w833:T1)
        n299 = call <vilib>:"Add State(s) to Queue__jki_lib_state_machine.vi"("State(s) in (\"\")"=w839) -> ("States Out"=w838:string)  [unwired: 14 in]
        n300 = Unbundle By Name(w833) -> ("9E Diagnostic Data"=w834:T48, "9F Diagnostic Data"=w832:T49)
        n301 = Bundle By Name(cluster=w835, "GEA Information Out.GEA Diagnostic Data - Washer.9E Diagnostic Data"=w834, "GEA Information Out.GEA Diagnostic Data - Washer.9F Diagnostic Data"=w832) -> (w837:T44)
      }
      frame "Debug Message" {
        # "If EOC, reset counter\nand Timer. Then save data\nwith Keys"
        n302 = Unbundle By Name(w875) -> ("GEA Information Out.Number of Messages"=w873:i32, "GEA Information Out.Full Message to Save"=w877:string, "GEA Information Out.Debug Search Parameters"=w878:T4, "Main Washer Display Out"=w876:T26)
        n303 = Greater Or Equal?(x=w873, y=1) -> (x >= y?=w884:bool)
        n304 = case shown="True" w884 {
          tunnel: ["" ("State(s) in Front (\"\")") "Get Remaining Messages" ("State(s) in Front (\"\")")] -> w882
          frame False {
          }
          frame True {
          }
        }
        n305 = Equal?(x="", y=w877) -> (x = y?=w879:bool)
        n306 = case shown="False" w879 {
          tunnel: w877 -> [w898 _]
          tunnel: w875 -> [w897 w906]
          tunnel: [w895 w906] -> w880
          tunnel: w876 -> [w891 _]
          tunnel: w878 -> [w892 _]
          tunnel: [w888 "" ("String")] -> w869
          frame False {
            # "Sets Colors"
            n307 = call "ViperHawk Write Network and Summary Files.vi"("Full Message to Save"=w898, "Debug Search Parameters"=w892, "Washer In"=w891) -> ("Debug Info"=w890:string[], "Day Cycle Count"=w894:i32)  [unwired: 9 in, 2 out]
            n308 = case shown="True" "Save Data" {
              tunnel: ["" ("String") "Save Data" ("String")] -> w888
              frame False {
              }
              frame True {
              }
            }
            n309 = Bundle By Name(cluster=w897, "GEA Information Out.Debug/GEA Data"=w890) -> (w896:T44)
            n310 = case shown="False" "Use GEA Cycle Counter" {
              tunnel: w896 -> [w903 w904]
              tunnel: [w902 w904] -> w895
              tunnel: w894 -> [w901 _]
              frame False {
                n311 = Bundle By Name(cluster=w903, "GEA Information Out.GEA Diagnostic Data - Washer.9E Diagnostic Data.Total Cycle Count (Current)"=w901) -> (w902:T44)
              }
              frame True {
              }
            }
            "Full Message to Save" <- w898
          }
          frame True {
          }
        }
        n312 = call <vilib>:"Add State(s) to Queue__jki_lib_state_machine.vi"("State(s) in Front (\"\")"=w882, "State(s) in (\"\")"=w874) -> ("States Out"=w871:string)  [unwired: 13 in]
        n313 = call <vilib>:"Add State(s) to Queue__jki_lib_state_machine.vi"("State(s) in Front (\"\")"=w869, "State(s) in (\"\")"=w871) -> ("States Out"=w870:string)  [unwired: 13 in]
      }
      frame "Update Graphs" {
        # "Update display"
        n314 = Unbundle By Name(w932) -> ("Main Washer Display Out"=w923:T26, "GEA Information Out.GEA Diagnostic Data - Washer"=w922:T1, "File Paths Out"=w925:T21, "Main Washer Display Out.Appliance Details.Appliance Common.Serial Number:"=→"Serial Number Front Panel":string, "Main Washer Display Out.Appliance Details.Appliance Common.Lab ID:"=→"Lab ID Front Panel":string, "Main Washer Display Out.Appliance Details.Appliance Common.TR Number:"=→"TR Number  Front Panel":string, "GEA Information Out"=→"GEA Information Out":T2, "GEA Information Out.GEA Diagnostic Data - Washer"=w908:T1, "Cycle Stats"=w924:T25)
        "Diagnostic Data Output" <- w922
        "Washer In" <- w923
        n315 = local write "File Locations In"(w925) -> ()
        n316 = local read "Cycle Timer"() -> (w921:dbl)
        n317 = local read "Enable Diagnostic Data"() -> (w909:T9)
        n318 = case shown="\"2015 Washer\", \"2017 Washer\"" w909 {
          tunnel: w908 -> [w938 _]
          tunnel: [w938 w939] -> w907
          frame "", Default {
          }
          frame "2015 Washer", "2017 Washer" {
            n319 = local read "Diagnostic Data Local"() -> (w939:T1)
          }
        }
        n320 = local read "HEWH Appliance Data"() -> (w916:string[][])
        n321 = local read "Cycle Count (0x008E)"() -> (w914:i32)
        n322 = local read "Basket Speed (RPM) (0xF30B)"() -> (w913:i32)
        n323 = local read "Current RMS (Amps) (0xF30D)"() -> (w912:dbl)
        n324 = local read "Machine Status Color"() -> (w911:u32)
        n325 = local read "Disable 15/17 Washer"() -> (w915:bool)
        n326 = call "ViperHawk Format Inv Data.vi"("Disable ERDs"=w915, "Timer"=w921, "Diagnostic Data Output"=w922, "Washer"=w923) -> ("Data W\\Header"=w917:string[][])  [unwired: 6 in, 1 out]
        n327 = local read "Save Data"() -> (w918:bool)
        n328 = Build Array (concatenate)(w917, w916) -> (w910:string[][])
        "GEA Data" <- w910
        n329 = call "ViperHawk Find Max Values.vi"("Error In"=w929, "Cycle Timer (Sec)"=w921, "Cycle Stats"=w924, "Diagnostic Data Output"=w907) -> ("Error Out"=w928:errorcluster, "Cycle Stats Output"=w927:T25)  [unwired: 6 in]
        "Max Values" <- w927
        n330 = case shown="False" w915 {
          tunnel: w932 -> [w948 w953]
          tunnel: [w947 w952] -> w931
          tunnel: w927 -> [w942 w951]
          tunnel: w918 -> [w940 w950]
          tunnel: w910 -> [w941 w949]
          tunnel: w914 -> [w946 _]
          tunnel: w913 -> [w945 _]
          tunnel: w912 -> [w944 _]
          tunnel: w911 -> [w943 _]
          frame False {
            n331 = Bundle By Name(cluster=w948, "Main Washer Display Out.Display Data (RLT).Saving Display"=w940, "GEA Information Out.GEA Data"=w941, "Cycle Stats"=w942, "Main Washer Display Out.Display Data (RLT).Cycle Count Display"=w946, "Main Washer Display Out.Display Data (RLT).RPM Display"=w945, "Main Washer Display Out.Display Data (RLT).Current Display"=w944, "Main Washer Display Out.Display Data (RLT).Status Color"=w943) -> (w947:T44)
          }
          frame True {
            n332 = Bundle By Name(cluster=w953, "Main Washer Display Out.Display Data (RLT).Saving Display"=w950, "GEA Information Out.GEA Data"=w949, "Cycle Stats"=w951) -> (w952:T44)
          }
        }
        n333 = case shown="True" w918 {
          tunnel: ["" ("String") "Save Data" ("String")] -> w920
          tunnel: ["Not Collecting Data...." ("Front Panel Status Read") "Collecting Data...." ("Front Panel Status Read")] -> w919
          frame False {
          }
          frame True {
          }
        }
        "Status" <- w919
        n334 = call <vilib>:"Add State(s) to Queue__jki_lib_state_machine.vi"("State(s) in Front (\"\")"=w920, "State(s) in (\"\")"=w937) -> ("States Out"=w936:string)  [unwired: 13 in]
      }
      frame "Save Data" {
        n335 = Unbundle By Name(w971) -> ("File Paths Out.Data File Paths.Debug File Path"=w961:path, "GEA Information Out.Debug/GEA Data"=w958:string[], "File Paths Out.Data File Paths.Data File Path"=w960:path, "GEA Information Out.GEA Data"=w967:string[][])
        n336 = Index Array(array=w967, index (col)=1 ("disabled index (col)")) -> (element=w959:string[])  [unwired: 1 in]
        n337 = call-poly <vilib>:"Write Delimited Spreadsheet.vi"("file path (dialog if empty)"=w960, "1D data"=w959, "append to file? (new file:F)"=TRUE, "delimiter (\\t)"="," ("delimiter (\\t)")) -> ()  [unwired: 10 in, 2 out]
        n338 = call-poly <vilib>:"Write Delimited Spreadsheet.vi"("file path (dialog if empty)"=w961, "1D data"=w958, "append to file? (new file:F)"=TRUE, "delimiter (\\t)"="," ("delimiter (\\t)")) -> ()  [unwired: 10 in, 2 out]
        n339 = call <vilib>:"Add State(s) to Queue__jki_lib_state_machine.vi"("State(s) in (\"\")"=w970) -> ("States Out"=w969:string)  [unwired: 14 in]
      }
    }
    n340 = case shown="True" "Read Debug States" {
      tunnel: w308 -> [_ w327]
      tunnel: w306 -> [w320 w328]
      tunnel: [w320 w321] -> w307
      frame False {
      }
      frame True {
        n341 = Build Array (concatenate)(w328, w327) -> (w321:string[])
        "Control States" <- w321
        n342 = Array Size(array=w321) -> (size(s)=w326:i32)
        n343 = Subtract(x=w326, y=10) -> (x-y=w324:i32)
        n344 = Array Subset(array=w321, index=w324, length=10) -> (→"Last 10 Control":string[])
      }
    }
  }
  n345 = call <vilib>:"Add State(s) to Queue__jki_lib_state_machine.vi"("State(s) in (\"\")"="Data: Initialize" ("State(s) in (\"\")")) -> ("States Out"=w31:string)  [unwired: 14 in]
  n346 = while "Initialize SM" {
    shift-right: [w984] -> _
    shift-left: _ -> [w983]
    shift-right: [w987] -> w26
    shift-left: _ -> [w981]
    shift-right: [w986] -> _
    shift-left: w31 -> [w988]
    shift-right: [w977] -> _
    shift-left: string[] [] -> [w979]
    tunnel: w13 -> [w975]
    tunnel: w20 -> [w974]
    tunnel: w18 -> [w973]
    i -> [w980]
    stop <- w985 stop-if-true
    # "Data Save"
    n347 = call <vilib>:"Parse State Queue__jki_lib_state_machine.vi"("State Queue"=w988, "Error In (no error)"=w981) -> ("Remaining States"=w990:string, "Current State"=w978:string, "Arguments"=w989:string)  [unwired: 11 in]
    n348 = case shown="\"Update Summary File\"" w978 {
      selector: w978 -> [_ _ _ w1082 _ _ _ _ _ _ _ _]
      tunnel: w990 -> [w1003 w1013 w1081 w1086 w1098 w1103 w1107 w1117 w1145 w1166 w1190 w1219]
      tunnel: w989 -> [_ _ _ _ _ _ _ _ _ _ _ _]
      tunnel: w983 -> [w1000 w1011 w1078 w1084 w1095 w1101 w1104 _ w1143 w1153 w1178 w1205]
      tunnel: [w1001 w1010 w1079 w1088 errorcluster {"status"=FALSE, "code"=0, "source"=""} ("error out") w1100 w1105 w1114 w1141 w1162 w1187 w1217] -> w987
      tunnel: w981 -> [w1001 w1009 w1079 w1087 w1094 w1100 w1105 w1114 w1142 w1159 w1184 w1215]
      tunnel: [w1002 w1012 w1080 w1085 w1097 w1102 w1106 w1116 w1144 w1165 w1189 w1218] -> w986
      tunnel: [_ _ _ _ _ TRUE _ _ _ _ _ _] -> w985
      tunnel: [w1000 w1008 w1078 w1084 w1095 w1101 w1104 w1115 w1143 w1152 w1177 w1203] -> w984
      tunnel: "Diagnostic Scan Rate" -> [_ w1007 _ _ _ _ _ _ _ _ _ _]
      tunnel: w975 -> [_ w1004 _ _ _ _ _ _ _ w1158 w1183 w1213]
      tunnel: w974 -> [_ w1006 _ _ _ _ _ _ _ _ _ _]
      tunnel: w973 -> [_ w1005 _ _ _ _ _ _ _ w1154 w1179 w1212]
      frame "---------ABOUT---------" {
        # "This SM handles the Initialization"
        n349 = call <vilib>:"Add State(s) to Queue__jki_lib_state_machine.vi"("State(s) in (\"\")"=w1003) -> ("States Out"=w1002:string)  [unwired: 14 in]
      }
      frame "", "Idle" {
        n350 = event shown="[1] <Trigger Summary>: User Event" {
          selector: w1006 -> [_ _ _]
          dyn-events: _ -> [_ _ _]
          timeout: w1007 -> [_ _ _]
          tunnel: w1013 -> [w1019 w1036 w1044]
          tunnel: [w1018 w1035 w1044] -> w1012
          tunnel: w1011 -> [w1016 w1034 w1045]
          tunnel: [w1017 w1037 w1041] -> w1010
          tunnel: w1009 -> [w1017 w1037 w1042]
          tunnel: [w1016 w1033 w1045] -> w1008
          tunnel: w1005 -> [_ _ w1040]
          tunnel: w1004 -> [_ _ w1039]
          event Timeout {
            n351 = event-data() -> ()  [unwired: 1 in, 1 out]
            n352 = shared-variable "My Computer\\Test Lib.lvlib\\Exit"() -> (w1014:bool)  [unwired: 1 in, 1 out]
            n353 = case shown="False" w1014 {
              tunnel: [w1022 "Exit"] -> w1015
              frame False {
                n354 = local read "Use GEA Cycle Counter"() -> (w1021:bool)
                n355 = local read "Disable 15/17 Washer"() -> (w1020:bool)
                n356 = case shown="True" w1021 {
                  tunnel: ["" w1025] -> w1022
                  tunnel: w1020 -> [_ w1024]
                  frame False {
                  }
                  frame True {
                    n357 = case shown="True" w1024 {
                      tunnel: ["Get ERDs" "Get Diagnostic Data1\nGet Diagnostic Data2"] -> w1025
                      frame False {
                      }
                      frame True {
                      }
                    }
                  }
                }
              }
              frame True {
              }
            }
            n358 = call <vilib>:"Add State(s) to Queue__jki_lib_state_machine.vi"("State(s) in Front (\"\")"=w1015, "State(s) in (\"\")"=w1019) -> ("States Out"=w1018:string)  [unwired: 13 in]
          }
          event User Event {
            n359 = event-data() -> ()  [unwired: 1 in, 5 out]
            n360 = local read "File Locations In"() -> (w1030:T21)
            n361 = local read "GEA Information Out"() -> (w1029:T2)
            n362 = local read "Max Values"() -> (w1031:T25)
            n363 = Bundle By Name(cluster=w1034, "File Locations Out"=w1030, "GEA Information Out"=w1029, "Cycle Stats"=w1031) -> (w1033:T51)
            n364 = call <vilib>:"Add State(s) to Queue__jki_lib_state_machine.vi"("State(s) in Front (\"\")"="Update Summary File" ("State(s) in Front (\"\")"), "State(s) in (\"\")"=w1036) -> ("States Out"=w1035:string)  [unwired: 13 in]
          }
          event Value Change {
            n365 = event-data() -> ("NewVal"=w1043:T9)  [unwired: 1 in, 5 out]
            n366 = case shown="\"\", Default" w1043 {
              tunnel: [T3 {"Critical Major SW Version"="", "Critical Minor SW Version"="", "Major SW Version"="", "Minor SW Version"="", "Parametric Data Ver. Major"="", "Parametric Data Ver. Minor"="", "Diagnostics Data Ver. Major"="", "Diagnostics Data Ver. Minor"="", "Current Personality Setting"=""} ("UI Version") w1054 w1067] -> w1038
              tunnel: w1042 -> [w1049 w1053 w1065]
              tunnel: [w1049 w1052 w1064] -> w1041
              tunnel: w1040 -> [_ w1051 w1063]
              tunnel: w1039 -> [_ w1050 w1062]
              frame "", Default {
              }
              frame "Viper Washer" {
                # "Enable Debug Logs"
                n367 = call "GEA2 Send and Receive Message.vi"("GEA2 Reference In"=w1050, "Input Data"=T18 {"Source"=228, "Destination"=35, "Command"=115, "Message"="1"}, "GEA2 Event Registration"=w1051, "Error In"=w1053) -> ("GEA2 Reference Out"=w1055:refnum<k24>, "Event Registration Out"=w1058:refnum<event-registration>, "Error Out"=w1057:errorcluster)  [unwired: 6 in, 3 out]
                n368 = call "GEA2 Send and Receive Message.vi"("GEA2 Reference In"=w1055, "Input Data"=T18 {"Source"=37, "Destination"=33, "Command"=1, "Message"=""}, "GEA2 Event Registration"=w1058, "Error In"=w1057) -> ("Converted Data Out"=w1060:T19, "Error Out"=w1052:errorcluster)  [unwired: 6 in, 4 out]
                n369 = Unbundle By Name(w1060) -> ("Message"=w1059:string)
                n370 = call "Save File Parse Software Version.vi"("Message"=w1059) -> ("UI Version"=w1054:T3)  [unwired: 10 in]
              }
              frame "Hawk Washer" {
                # "Enable Debug Logs"
                n371 = call "GEA2 Send and Receive Message.vi"("GEA2 Reference In"=w1062, "Input Data"=T18 {"Source"=228, "Destination"=37, "Command"=115, "Message"="1"}, "GEA2 Event Registration"=w1063, "Error In"=w1065) -> ("GEA2 Reference Out"=w1068:refnum<k24>, "Event Registration Out"=w1071:refnum<event-registration>, "Error Out"=w1070:errorcluster)  [unwired: 6 in, 3 out]
                n372 = call "GEA2 Send and Receive Message.vi"("GEA2 Reference In"=w1068, "Input Data"=T18 {"Source"=37, "Destination"=33, "Command"=1, "Message"=""}, "GEA2 Event Registration"=w1071, "Error In"=w1070) -> ("Converted Data Out"=w1073:T19, "Error Out"=w1064:errorcluster)  [unwired: 6 in, 4 out]
                n373 = Unbundle By Name(w1073) -> ("Message"=w1072:string)
                n374 = call "Save File Parse Software Version.vi"("Message"=w1072) -> ("UI Version"=w1067:T3)  [unwired: 10 in]
              }
            }
            "Software Version" <- w1038
            n375 = case shown="\"2015 Washer\", \"2017 Washer\"" "Enable Diagnostic Data" {
              tunnel: [TRUE TRUE TRUE FALSE] -> w1046
              frame "", Default {
              }
              frame "Viper Washer" {
              }
              frame "Hawk Washer" {
              }
              frame "2015 Washer", "2017 Washer" {
              }
            }
            n376 = local write "Disable 15/17 Washer"(w1046) -> ()
          }
        }
      }
      frame "---------- Core ----------" {
        n377 = call <vilib>:"Add State(s) to Queue__jki_lib_state_machine.vi"("State(s) in (\"\")"=w1081) -> ("States Out"=w1080:string)  [unwired: 14 in]
      }
      frame Default {
        w1091 = 42 items=["No error", "Argument error", "Memory is full", "Out of zone", "End of file", "File already open", "Generic file I/O error", "File not found", "File permission error", "Disk is full", "Duplicate path", "Too many files open", "System feature not enabled", "Resource file not found", "Cannot add resource", "Resource not found", "Image not found", "Image memory error", "Pen does not exist", "Config type invalid", "Config token not found", "Config parse error", "Config memory error", "Bad external code format", "Bad external code offset", "External code not present", "Null window", "Destroy window error", "Null menu", "Print aborted", "Bad print record", "Print driver error", "Windows error during printing", "Memory error during printing", "Print dialog error", "Generic print error", "Invalid device refnum", "Device not found", "Device parameter error", "Device unit error", "Cannot open device", "Device call aborted", "Generic error", "Cancelled by user", "Object ID too low", "Object ID too high", "Object not in heap", "Unknown heap", "Unknown object (invalid DefProc)", "Unknown object (DefProc not in table)", "Message out of range", "Invalid (null) method", "Unknown message", "Manager call not supported", "Bad address", "Network operation in progress", "Network operation timed out", "Connection is busy", "Network attribute not supported", "Network error", "Address in use", "System out of memory", "Connection aborted", "Connection refused", "Not connected", "Already connected", "Connection closed", "Initialization error (interapplication manager)", "Bad occurrence", "Wait on unbound occurrence handler", "Occurrence queue overflow", "Datalog type conflict", "Unused", "Unrecognized type (interapplication manager)", "Memory corrupt", "Failed to make temporary DLL", "Old CIN version", "Drag socket not found", "Failed to load drop-object", "Failed to register OLE object", "Failed to release OLE object", "Format specifier type mismatch", "Unknown format specifier", "Too few format specifiers", "Too many format specifiers", "Scan failed", "Newer CIN version", "Error converting to variant", "Runtime menu error", "Password tampered", "Variant attribute not found", "Incompatible variant data type", "Event data is not available", "Event Store is not present", "Occurrence is not found", "Event Queue is not created", "Event info is not available", "Refnum passed is NULL", "Error retrieving Class GUID", "Error retrieving CoClass GUID", "Error retrieving TypeLib GUID.", "Bad built application magic bytes.", "Specific driver is different from the specific driver associated with the Logical Name.", "There is no session opened to the class driver.", "Max Error", "MAX - Error with config objects", "MAX - Error loading configuration", "MAX - Group not supported"]
        # "Current State"
        # "Handle mistyped state name (developer tool)"
        n378 = Format Into String(format string="Software Exception: Unhandled State \"%s\"." ("message"), error in=w1087, w1082) -> (resulting string=w1090:string, error out=w1089:errorcluster)  [unwired: 1 in]
        n379 = call <vilib>:"Error Cluster From Error Code.vi"("show call chain? (False)"=TRUE, "error in (no error)"=w1089, "error message (\"\")"=w1090, "error code (0)"=w1091) -> ("error out"=w1088:errorcluster)  [unwired: 5 in]
        n380 = call <vilib>:"Add State(s) to Queue__jki_lib_state_machine.vi"("State(s) in (\"\")"=w1086) -> ("States Out"=w1085:string)  [unwired: 14 in]
      }
      frame "Error Handler" {
        # "Unhandled Error -- Display it"
        # "Clear error"
        n381 = call <vilib>:"General Error Handler.vi"("error in (no error)"=w1094) -> ()  [unwired: 10 in, 5 out]
        n382 = call <vilib>:"Add State(s) to Queue__jki_lib_state_machine.vi"("State(s) in Front (\"\")"="/* Post Error States", "State(s) in (\"\")"=w1098) -> ("States Out"=w1097:string)  [unwired: 13 in]
      }
      frame "Exit" {
        n383 = call <vilib>:"Add State(s) to Queue__jki_lib_state_machine.vi"("State(s) in (\"\")"=w1103) -> ("States Out"=w1102:string)  [unwired: 14 in]
      }
      frame "---------- Data ----------" {
        n384 = call <vilib>:"Add State(s) to Queue__jki_lib_state_machine.vi"("State(s) in (\"\")"=w1107) -> ("States Out"=w1106:string)  [unwired: 14 in]
      }
      frame "Data: Initialize" {
        n385 = while {
          tunnel: [w1123] -> w1113
          tunnel: [w1122] -> w1112
          tunnel: [w1121] -> w1111
          tunnel: [w1119] -> w1110
          tunnel: [w1120] -> w1109
          tunnel: [w1118] -> w1108
          stop <- w1124 stop-if-true
          w1118 = T2 {"GEA Diagnostic Data - Washer"={"Speed (RPM)"=0, "Load Size"=0, "Temperature"=0, "Water Pressure"=0.0, "Detergent"=0, "Fabric Softener"=0, "Tub Direction"="", "Detergent Valve"=FALSE, "Fabric Softener Valve"=FALSE, "Recirculating Pump"=FALSE, "Drain Valve"=FALSE, "Hot Valve"=FALSE, "Cold Valve"=FALSE, "Lid Closed Status"="", "Lid Lock Status"="", "Error Count"=0, "IGBT Temperature (Deg C)"=0, "Motor Speed"=0, "Latched OOB"=0, "Raw OOB"=0, "Plaster Status"=0, "Inverter Power (W)"=0, "Target Speed(BRPM)"=0, "Latched Agitate Motor Temp (Deg C)"=0, "Current Motor Temp (Deg C)"=0, "Profiler Status"="", "Current Inverter Action"="", "Error Codes"="", "Lid Locked"=FALSE, "Lid Closed"=FALSE, "9E Diagnostic Data"={"Total Cycle Time (Min)"=0, "Total Cycle Count (Current)"=0, "Total Error Count"=0, "Machine Error History"=0, "Washer UI History"=0, "Inverter Error History"=0, "Cycle Storage Limit"=0, "Error Storage Limit"=0, "Cycle Pages Supported"=0, "Error Pages Supported"=0, "Inverter Reset Count"=0}, "9F Diagnostic Data"={"Cycle Buffer Index"="", "Page Number"="", "Total Cycle Count"=0, "Delay Start Time"=0, "Stain Selected"="", "Selected Cycle"=0, "eWash"="", "Soil Level"="", "Temperature"="", "Overnight Ready"="", "Spin Setting"="", "Control Lock Status"="", "Stain Remover"="", "Steam Assist"="", "My Cycle"="", "PreWash"="", "Debug Log Enabled"="", "Rinse"="", "Signal Level"="", "PreSoak"=""}}, "Software Version"={"Critical Major SW Version"="", "Critical Minor SW Version"="", "Major SW Version"="", "Minor SW Version"="", "Parametric Data Ver. Major"="", "Parametric Data Ver. Minor"="", "Diagnostics Data Ver. Major"="", "Diagnostics Data Ver. Minor"="", "Current Personality Setting"=""}, "Debug Search Parameters"={"Pause"=["MchStdby", "MchPz", "MchIdl", "Machine Standby", "Machine Pause", "Machine Idle"], "Run"=["MchRn", "Machine Run", "Resume Process"], "EOC"=["EOC"], "Error Codes"=["Error1", "try", "rty", "inverr"]}, "Message Count"=0, "Number of Messages"=0, "Partial Message String"="", "Full Message to Save"="", "Board ID"="", "Board Index"=0, "Source Address"=0, "Destination Address"=0, "Data to send"=[], "ReceivedData"=[], "Debug/GEA Data"=[], "Command"=0, "GEA2 Reference Out"=refnum, "GEA2 Event Registration"=refnum, "Bus Data"="", "GEA Data"=[], "Network Variable Location"=0, "Water Heater GEA2 Data"={"GEA2 Label Array"=[], "PID_PARAMETERS"=[], "SUPPORTED_MODES"=[], "Button Status"={"Switch 1"=FALSE, "Switch 2"=FALSE, "Switch 3"=FALSE, "Switch 4"=FALSE, "Switch 5"=FALSE, "Switch 6"=FALSE, "Switch 7"=FALSE, "Switch 8"=FALSE, "Switch 9"=FALSE, "Switch 10"=FALSE, "Switch 11"=FALSE, "Switch 12"=FALSE, "Switch 13"=FALSE, "Switch 14"=FALSE, "Switch 15"=FALSE, "Switch 16"=FALSE}, "Status Query"={"Days Remaining (For Std Electric and Vacation)"=0, "Unit Status"="", "Current Tank Temp in Deg F"=0, "Current Setpoint in Deg F"=0, "Filter Status (% used)"=0, "Fallback Status (Fallback heating mode)"="", "Fallback Temp"=0, "\"Set Mode\" Selection"=""}, "Service Error Codes"={"Reserved"=FALSE, "Reserved 1"=FALSE, "Reserved 2"=FALSE, "Reserved 3"=FALSE, "Reserved 4"=FALSE, "Reserved 5"=FALSE, "Reserved 6"=FALSE, "Reserved 7"=FALSE, "DataFlash Fail Status"=FALSE, "Stuck Key Fail Status"=FALSE, "Dry Tank Fail Status"=FALSE, "Miswire Fail Status"=FALSE, "Reserved 8"=FALSE, "Reserved 9"=FALSE, "Reserved 10"=FALSE, "Reserved 11"=FALSE, "UE Fail Status"=FALSE, "LE Fail Status"=FALSE, "Filter Fail Status"=FALSE, "T3A Fail Status"=FALSE, "T3B Fail Status"=FALSE, "T4 Fail Status"=FALSE, "T5 Fail Status"=FALSE, "T2 Fail Status"=FALSE, "SS Cond A Status"=FALSE, "SS Cond B Status"=FALSE, "SS Cond C Status"=FALSE, "SS Cond D Status"=FALSE, "SS Cond E Status"=FALSE, "SS Cond F Status"=FALSE, "SS Fan Status"=FALSE, "CMP Fail Status"=FALSE}, "HEM_KWH_DATA"=[], "OTHER_FAULT_COUNTS"=[], "GEA2 Raw Message"="", "Hyperterminal Data"={"Source"=0, "Destination"=0, "Command"=0, "Length"=0, "CRC"=0, "UE - state (1/0 on off)"=0, "LE - state (1/0 on off)"=0, "Comp - state (1/0 on off)"=0, "Fan  - state (1/0 on off)"=0, "Setpoint Deg F"=0, "T2(TankSensor)"=0.0, "T3A(EvapIn)"=0.0, "T3B(EvapOut)"=0.0, "T4(CompressorDischarge)"=0.0, "T5(Ambient)"=0.0, "Current"=0.0, "Voltage (Volts)"=0, "EEV Position (0-480)"=0, "Reason for last heating cycle termination"=0, "Reason Data word 1"="", "Reason Data word 2"="", "Reason Data word 3"="", "Reason Data word 4"="", "SW Debug Data"="", "Flow Events (Bit Encoded)"=0, "Heating Control Mode"=0}, "Extra Data"={"Water Capacity (Gallons)"=0, "Max Vacation Duration Days"=0, "Min Vacation Duration Days"=0, "Max Set Point (Deg F)"=0, "Min Set Point (Deg F)"=0, "T5 Resistance"=0, "T4 Resistance"=0, "T3B Resistance"=0, "T2 Resistance"=0, "STD_ELEC_RANGE"="", "SS_FAULT_COUNTS"="", "SERIAL_NUMBER"="", "READ_PERSONALITY"=0, "RQST_OVERRIDE_STATUS"="", "MODEL_SELECT_AD_VALUE"=0, "MODEL NUMBER"="", "IDLB_RESISTANCE"=0, "DSM Override Status"="", "RQST_DATA_FROM_Memory"="", "RQST_DATA_FROM_DATA_FLASH"="", "RQST_CURRENT_PID_SH_TARGET"=0, "Unit System Mode"=""}}}  # GEA Information Out
          w1119 = T21 {"General Setup Paths"={"Calibration File Path"=path "", "DOE Capacity Path"=path "", "Data Folder Path"=path "", "RLT Backup Data Path"=path "", "Tool Base Path"=path "", "General Startup Config Path"=path "", "File Save Previous Run Path"=path "", "File Save Configuration Data Path"=path ""}, "Data File Paths"={"Data File Path"=path "", "Debug File Path"=path "", "Bus Log Path"=path "", "Current"=path "", "Summary"=path ""}, "New Summary Created"=FALSE, "Check Location Interval (Second)"=0}  # File Locations Out
          w1120 = T1 {"Speed (RPM)"=0, "Load Size"=0, "Temperature"=0, "Water Pressure"=0.0, "Detergent"=0, "Fabric Softener"=0, "Tub Direction"="", "Detergent Valve"=FALSE, "Fabric Softener Valve"=FALSE, "Recirculating Pump"=FALSE, "Drain Valve"=FALSE, "Hot Valve"=FALSE, "Cold Valve"=FALSE, "Lid Closed Status"="", "Lid Lock Status"="", "Error Count"=0, "IGBT Temperature (Deg C)"=0, "Motor Speed"=0, "Latched OOB"=0, "Raw OOB"=0, "Plaster Status"=0, "Inverter Power (W)"=0, "Target Speed(BRPM)"=0, "Latched Agitate Motor Temp (Deg C)"=0, "Current Motor Temp (Deg C)"=0, "Profiler Status"="", "Current Inverter Action"="", "Error Codes"="", "Lid Locked"=FALSE, "Lid Closed"=FALSE, "9E Diagnostic Data"={"Total Cycle Time (Min)"=0, "Total Cycle Count (Current)"=0, "Total Error Count"=0, "Machine Error History"=0, "Washer UI History"=0, "Inverter Error History"=0, "Cycle Storage Limit"=0, "Error Storage Limit"=0, "Cycle Pages Supported"=0, "Error Pages Supported"=0, "Inverter Reset Count"=0}, "9F Diagnostic Data"={"Cycle Buffer Index"="", "Page Number"="", "Total Cycle Count"=0, "Delay Start Time"=0, "Stain Selected"="", "Selected Cycle"=0, "eWash"="", "Soil Level"="", "Temperature"="", "Overnight Ready"="", "Spin Setting"="", "Control Lock Status"="", "Stain Remover"="", "Steam Assist"="", "My Cycle"="", "PreWash"="", "Debug Log Enabled"="", "Rinse"="", "Signal Level"="", "PreSoak"=""}}  # Diagnostic
          w1121 = T25 {"RPM Max"=0, "Cycle Time"=0.0, "IGBT Temperature"=0.0, "Load Size"=0.0, "Temperature"=0.0, "Water Pressure"=0.0, "Detergent"=0.0, "Fabric Softener"=0.0, "Inverter Power (W)"=0.0, "Raw OOB"=0.0, "Current Motor Temp (Deg C)"=0.0}  # Cycle Stats
          w1122 = T43 {"Cycle Timer"=0.0, "Timer"=0.0}  # Timers
          w1123 = T50 {"Summary Header"=["Date", "Time", "Total Cycle Time (Seconds)", "Cycle Number", "Maximum RPM", "# of Error Codes", "Maximum Current"], "Current Header"=["Date", "Time", "Time (Seconds)", "Current (Amps)"], "Debug Log Header"=["Date", "Time", "Debug Logs"], "Data Header"=["Date", "Time", "Time (Seconds)", "IGBT Temperature", "Speed", "Load Size", "Temperature", "Water Pressure", "Detergent", "Fabric Softener", "Direction", "Detergent Valve", "Fabric Softener Valve", "Recirculating Pump", "Drain Valve", "Hot Water Valve", "Cold Water Valve", "Lid Status", "Lid Lock Status"]}  # Headers
          n386 = local read "Start UI Loop"() -> (w1124:bool)
          n387 = Wait Until Next ms Multiple(millisecond multiple=u32 100) -> ()  [unwired: 1 out]
        }
        n388 = call <vilib>:"Add State(s) to Queue__jki_lib_state_machine.vi"("State(s) in (\"\")"=w1117) -> ("States Out"=w1116:string)  [unwired: 14 in]
        n389 = Bundle("GEA Information Out"=w1108, "Headers"=w1113, "Timers"=w1112, "File Locations Out"=w1110, "Cycle Stats"=w1111, "Diagnostic"=w1109) -> (w1115:T51)  [unwired: 1 in]
      }
      frame "Update Summary File" {
        # "This reads, fixes, and sorts the summary file"
        n390 = Unbundle By Name(w1143) -> ("GEA Information Out.GEA Diagnostic Data - Washer.Error Count"=w1128:u32, "GEA Information Out.GEA Diagnostic Data - Washer.9E Diagnostic Data.Total Cycle Count (Current)"=w1129:u16, "Cycle Stats"=w1130:T25)
        n391 = Unbundle By Name(w1143) -> ("File Locations Out.Data File Paths.Summary"=w1134:path)
        n392 = Get Date/Time In Seconds() -> (seconds since 1Jan1904=w1140:timestamp)
        n393 = Format Date/Time String(time format string (%c)="%m/%d/%Y %H:%M:%S%3u", seconds (now)=w1140) -> (date/time string=w1138:string)  [unwired: 1 in]
        n394 = flat-sequence {
          tunnel: w1142 -> [w1147]
          tunnel: [w1147] -> w1141
          frame #0 {
            n395 = local write "UI Event SM"("Reset Cycle Stats") -> ()
          }
        }
        n396 = call <vilib>:"Space Constant.vi"() -> ("String"=w1137:string)
        n397 = Match Pattern(string=w1138, regular expression=w1137) -> (before substring=w1136:string, after substring=w1135:string)  [unwired: 1 in, 2 out]
        n398 = call "Save File Check and Fix Summary File.vi"("LV Program"=Save_File_DOE_LabView_Program."HCC", "file path (dialog if empty)"=w1134) -> ("Summary Path"=w1133:path)  [unwired: 8 in, 1 out]
        n399 = call "ViperHawk Summary Stats.vi"("Cycle Stats"=w1130, "Day Cycle Count"=w1129, "Error Code Out"=w1128, "Time"=w1135, "Date"=w1136) -> ("Summary Data"=w1126:string[])  [unwired: 6 in]
        n400 = call-poly <vilib>:"Write Delimited Spreadsheet.vi"("file path (dialog if empty)"=w1133, "1D data"=w1126, "append to file? (new file:F)"=TRUE, "delimiter (\\t)"="," ("delimiter (\\t)")) -> ()  [unwired: 10 in, 2 out]
        n401 = call <vilib>:"Add State(s) to Queue__jki_lib_state_machine.vi"("State(s) in (\"\")"=w1145) -> ("States Out"=w1144:string)  [unwired: 14 in]
      }
      frame "Get Diagnostic Data1" {
        n402 = local read "Enable Diagnostic Data"() -> (w1148:T9)
        n403 = Unbundle By Name(w1153) -> ("Diagnostic"=w1163:T1)
        n404 = case shown="\"Viper Washer\"" w1148 {
          tunnel: [u8 0 ("Command") u8 228 ("Command") u8 228 ("Command")] -> w1150
          tunnel: [u8 0 ("Command") u8 35 ("Command") u8 37 ("Command")] -> w1149
          frame Default {
          }
          frame "Viper Washer" {
          }
          frame "Hawk Washer" {
          }
        }
        n405 = Bundle By Name(cluster=T18 {"Source"=0, "Destination"=0, "Command"=0, "Message"=""} ("Input Data"), "Source"=w1150, "Destination"=w1149, "Command"=u8 158) -> (w1155:T18)
        n406 = call "HCC Get Viper Diagnostics.vi"("GEA Ref In"=w1158, "GEA2 Event Registration"=w1154, "Diagnostic"=w1163, "Input Data"=w1155, "error in (no error)"=w1159) -> ("Diagnostic Data Output"=w1151:T1, "Converted Data Out"=→"Converted Data Out":T19, "error out"=w1160:errorcluster)  [unwired: 10 in, 2 out]
        n407 = Bundle By Name(cluster=w1153, "Diagnostic"=w1151) -> (w1152:T51)
        n408 = call "UTILITY Delay mS.vi"("Error In"=w1160, "milliseconds to wait"=u32 500) -> ("Error Out"=w1162:errorcluster)  [unwired: 13 in]
        n409 = call <vilib>:"Add State(s) to Queue__jki_lib_state_machine.vi"("State(s) in (\"\")"=w1166) -> ("States Out"=w1165:string)  [unwired: 14 in]
      }
      frame "Get Diagnostic Data2" {
        n410 = local read "Enable Diagnostic Data"() -> (w1173:T9)
        n411 = case shown="Default" w1173 {
          tunnel: [u8 0 ("Command") u8 228 ("Command") u8 228 ("Command")] -> w1175
          tunnel: [u8 0 ("Command") u8 35 ("Command") u8 37 ("Command")] -> w1174
          frame Default {
          }
          frame "Viper Washer" {
          }
          frame "Hawk Washer" {
          }
        }
        n412 = Unbundle By Name(w1178) -> ("Diagnostic"=w1188:T1)
        n413 = Bundle By Name(cluster=T18 {"Source"=0, "Destination"=0, "Command"=0, "Message"=""} ("Input Data"), "Source"=w1175, "Destination"=w1174, "Command"=u8 159) -> (w1180:T18)
        n414 = call "HCC Get Viper Diagnostics.vi"("GEA Ref In"=w1183, "GEA2 Event Registration"=w1179, "Diagnostic"=w1188, "Input Data"=w1180, "error in (no error)"=w1184) -> ("Diagnostic Data Output"=w1176:T1, "error out"=w1185:errorcluster)  [unwired: 10 in, 3 out]
        "Diagnostic Data Local" <- w1176
        n415 = Bundle By Name(cluster=w1178, "Diagnostic"=w1176) -> (w1177:T51)
        n416 = call "UTILITY Delay mS.vi"("Error In"=w1185, "milliseconds to wait"=u32 500) -> ("Error Out"=w1187:errorcluster)  [unwired: 13 in]
        n417 = call <vilib>:"Add State(s) to Queue__jki_lib_state_machine.vi"("State(s) in (\"\")"=w1190) -> ("States Out"=w1189:string)  [unwired: 14 in]
      }
      frame "Get ERDs" {
        n418 = local read "Enable Diagnostic Data"() -> (w1199:T9)
        n419 = case shown="\"\", Default" w1199 {
          tunnel: [TRUE FALSE] -> w1206
          frame "", Default {
          }
          frame "2015 Washer", "2017 Washer" {
          }
        }
        "Disable 15/17 Washer" <- w1206
        n420 = Unbundle By Name(w1205) -> ("Diagnostic"=w1201:T1)
        n421 = call "GEA2 HEWH Appliance Data.vi"(".NET Refnum in"=w1213, "LV Program"=Save_File_DOE_LabView_Program."Portable Stand", "GEA2 Event Registration In"=w1212, "error in (no error)"=w1215, "Enable Diagnostic Data"=w1199, "#ERDs per message"="#ERDs per message", "Disable ERD A"=w1206) -> ("UnRead ERDs"=→"UnRead ERDs":i32, "HEWH Appliance Data ERD"=w1202:string[][], "error out"=w1214:errorcluster)  [unwired: 6 in, 4 out]
        "HEWH Appliance Data" <- w1202
        n422 = local read "Fault Set?"() -> (w1197:bool)
        n423 = call <vilib>:"Add State(s) to Queue__jki_lib_state_machine.vi"("State(s) in (\"\")"=w1219) -> ("States Out"=w1218:string)  [unwired: 14 in]
        n424 = call "HCC 2015 Parse.vi"("Fault Set?"=w1197, "HEWH Appliance Data"=w1202, "Diagnostic"=w1201) -> ("Basket Speed (RPM) (0xF30B)"=→"Basket Speed (RPM) (0xF30B)":i32, "Current RMS (Amps) (0xF30D)"=→"Current RMS (Amps) (0xF30D)":dbl, "Machine Status Color"=→"Machine Status Color":u32, "Cycle Count (0x008E)"=→"Cycle Count (0x008E)":i32, "Diagnostic Out"=w1200:T1)  [unwired: 4 in]
        n425 = local write "Diagnostic Data Local"(w1200) -> ()
        n426 = Bundle By Name(cluster=w1205, "Diagnostic"=w1200) -> (w1203:T51)
        n427 = call "UTILITY Delay mS.vi"("Error In"=w1214, "milliseconds to wait"=u32 500) -> ("Error Out"=w1217:errorcluster)  [unwired: 13 in]
      }
    }
    n428 = local read "Read Debug States"() -> (w976:bool)
    n429 = case shown="True" w976 {
      tunnel: w978 -> [_ w998]
      tunnel: w979 -> [w991 w999]
      tunnel: [w991 w997] -> w977
      frame False {
      }
      frame True {
        n430 = Build Array (concatenate)(w999, w998) -> (w997:string[])
        "Data Save Loop" <- w997
        n431 = Array Size(array=w997) -> (size(s)=w996:i32)
        n432 = Subtract(x=w996, y=10) -> (x-y=w994:i32)
        n433 = Array Subset(array=w997, index=w994, length=10) -> (→"Last 10 Data Save":string[])
      }
    }
    "Data Save Loop" <- w980
  }
  n434 = call "GEA2 Stop.vi"("GEA2 Reference Out"=w13, "Error In"=w26) -> ()  [unwired: 13 in, 1 out]
  n435 = stacked-sequence {
    frame #0 {
      # "Fix the inverter data plot"
    }
  }
  n436 = Destroy User Event(user event=w24, error in=w25) -> ()  [unwired: 1 out]
